vi "LabviewImageProcess with Matlab.vi"() -> ()   [LabVIEW 2015]
doc: "This is the interface, the one VI which loads all the others. Run this one first.\n\n(the line below ensures settings are saved)\n[Red Tweezers Save Settings]"
uses:
  red_tweezers_1_4_release/subvis/line_trapping.ctl
  red_tweezers_1_4_release/subvis/spot.ctl
  <vilib>/userdefined/High Color/IMAQdx.ctl
  red_tweezers_1_4_release/subvis/selection_element.ctl
  red_tweezers_1_4_release/subvis/mouse_info.ctl
  <vilib>/Analysis/baseanly.llb/Real A x B.vi
  red_tweezers_1_4_release/subvis/red_tweezers_globals_INTERNAL_VOLATILE.vi
  red_tweezers_1_4_release/subvis/red_tweezers_globals.vi
  <vilib>/Analysis/NI_AALBase.lvlib
  <vilib>/vision/driver/NI_Vision_Acquisition_Software.lvlib
  <vilib>/vision/NI_Vision_Development_Module.lvlib
panel:
  out "Spot Storage":T1[](array[typedef]) {"Amplitude Correction" step=0.1; "Line Trapping"."Phase Gradient" step=0.05; "Line Trapping"."Vector"."x" step=1e-06 format="%#_6p"; "Line Trapping"."Vector"."y" step=1e-06 format="%#_6p"; "Line Trapping"."Vector"."z" step=1e-06 format="%#_6p"; "NA Position"."r" step=1e-06; "NA Position"."y" step=1e-06; "NA Position"."x" step=1e-06; "Position"."z" step=1e-06; "Position"."y" step=1e-06; "Position"."x" step=1e-06; "Phase" step=0.7753; "Intensity" step=0.1}
  out "# selected":i16
  out "Last Pattern":T1[](array[typedef]) {"Amplitude Correction" step=0.1; "Line Trapping"."Phase Gradient" step=0.05; "Line Trapping"."Vector"."x" step=1e-06 format="%#_6p"; "Line Trapping"."Vector"."y" step=1e-06 format="%#_6p"; "Line Trapping"."Vector"."z" step=1e-06 format="%#_6p"; "NA Position"."r" step=1e-06; "NA Position"."y" step=1e-06; "NA Position"."x" step=1e-06; "Position"."z" step=1e-06; "Position"."y" step=1e-06; "Position"."x" step=1e-06; "Phase" step=0.7753; "Intensity" step=0.1}
  out "Plugins":T3(array[cluster])=[{"Name"="ASI Stage", "Folder"=path "C:/Users/Richard Bowman/Dropbox/red_tweezers_1_4_rc4/plugins/ASI Stage.llb", "vi reference"=refnum, "Needs to be run"=TRUE, "Error"={"status"=FALSE, "code"=0, "source"=""}}, {"Name"="iTweezers", "Folder"=path "C:/Users/Richard Bowman/Dropbox/red_tweezers_1_4_rc4/plugins/iTweezers.llb", "vi reference"=refnum, "Needs to be run"=TRUE, "Error"={"status"=FALSE, "code"=0, "source"=""}}, {"Name"="MightexLED", "Folder"=path "C:/Users/Richard Bowman/Dropbox/red_tweezers_1_4_rc4/plugins/MightexLED.llb", "vi reference"=refnum, "Needs to be run"=TRUE, "Error"={"status"=FALSE, "code"=0, "source"=""}}]
  in  "Tab":T4(tab)
  out "Play Pressed":bool
  out "Y":dbl
  out "X":dbl
  in  "O Button":bool
  in  "OK Button":bool
  in  "Bubble Size":dbl=50.0002
  out "Hit Indicator":bool
  in  "On":bool
  out "Induce check":bool
  out "Area+ Buffer":dbl
  in  "Area to check":dbl=0.00025
  out "Prev Current Spot":dbl
  out "spots selected 2":i32=4
  out "Spot # Check":dbl
  out "Orig Y SC":dbl
  out "Orig X SC":dbl
  out "ID num check":dbl
  out "Value Check":dbl
  out "ID":dbl[](array[numeric])
  out "Null array":dbl[](array[numeric])
  out "Potential Collisions":dbl
  out "What to Check":dbl[](array[numeric])
  out "Num":dbl
  out "Old Y":dbl
  out "Old X":dbl
  out "init":dbl
  out "Looper":bool
  in  "Output to SLM":bool
  out "Maximum":dbl
  out "Projected Distance":dbl
  out "Previous Distance":dbl
  out "Group ID #":dbl
  in  "Buffer Zone":dbl=7e-05
  out "# of Spots":dbl
  out "Distance":dbl
  out "Hit":bool
  out "Y Displacement":dbl
  out "X Displacement":dbl
  out "Current Spot #":dbl
  out "spots selected":i32=4
  in  "lock aspect ratio":bool=TRUE
  in  "Size":cluster{"x":dbl, "y":dbl, "z":dbl} {"z" step=1e-06 format="%#_4p"; "y" step=1e-06 format="%#_4p"; "x" step=1e-06 format="%#_4p"}
  in  "Position":cluster{"x":dbl, "y":dbl, "z":dbl}={"x"=1e-06, "y"=-6.3e-06, "z"=0.0} {"z" step=1e-06 format="%#_4p"; "y" step=1e-06 format="%#_4p"; "x" step=1e-06 format="%#_4p"}
  in  "phase":dbl step=0.7753
  in  "Vortex Charge":i8
  in  "Intensity":dbl=1.0 step=0.1
  in  "add to selection":bool
  in  "random position":bool
  in  "new spot":bool
  in  "delete":bool
  out "Execution Time":u32
  in  "rotate":bool
  in  "Rotation Axis":u16(ring)=2 items=["Z", "X", "Y", "Custom"]
  in  "Angle (degrees)":dbl=2.0
  in  "Custom Axis":cluster{dbl, dbl, dbl}
  in  "Spot Shape":enum32{"Normal", "Line", "NA", "Mixed"}(tab)=enum."Mixed"
  in  "Line Trapping":T2 {"Phase Gradient" step=0.05; "Vector"."x" step=1e-06 format="%#_4p"; "Vector"."y" step=1e-06 format="%#_4p"; "Vector"."z" step=1e-06 format="%#_4p"}
  in  "Scale back aperture":dbl=1.1 step=0.1
  in  "Scale BA":bool
  in  "Position on back aperture":cluster{"x":dbl, "y":dbl}={"x"=-5.84327907697451e-18, "y"=0.0} {"y" step=0.1 format="%#_4p"; "x" step=0.1 format="%#_4p"}
  in  "Radius on back aperture":dbl=1.1 step=0.1
  in  "Generate":bool
  in  "Pattern":T5(tab)
  in  "Spots across centre":i32=5
  in  "Reference Array?":bool
  in  "Fraction of SLM":dbl=1.0
  in  "Spots across centre":i32=5
  in  "N":cluster{i32, i32}
  in  "spacing/m":dbl=2.0
  in  "Iterations":i32=10
  out "non-uniformity":dbl(slide)=0.031119223416512406 scale=0.0..0.2
  out "efficiency":dbl(slide)=0.8985936267644501 scale=0.0..1.0
  in  "Optimise":bool
  in  "Reset Phase/Amplitude":bool
  in  "Fall-off/m":dbl=0.00025 min=0.0 step=1e-06 format="%#_4p"
  in  "Abort Plugin":bool
  in  "Plugin:":u16(ring)=1 items=["ASI Stage", "iTweezers", "MightexLED"]
  in  "Save Video":bool
  in  "Global ROI (requires restart)":i32[](array[numeric])=[0, 0, 1280, 512]
  in  "Zoom":bool
  in  "Draw ROI":bool
  in  "Zoom to Fit":bool
  out "Image Information":string="640x480 1.93X 8-bit image 255    (0,0)"
  in  "Camera":T6
  in  "Time per Frame (ms)":dbl
  in  "Edit Sequence Mode":bool
  in  "Manual Edit":bool
  in  "Bubble ID to Empty":dbl
  in  "Clearance Button":bool
  in  "Manual Sequence":bool
  in  "Play Sequence":bool
  in  "Reset":bool
  out "Sequence Instances":dbl
  out "Counter":dbl
  in  "Save State":bool
  out "Sequence On?":bool
  in  "Sequence Order":dbl
  out "Selection/Group":T7[](array[typedef])
  in  "Sequence Storer":T1[][](array[typedef]) {"Amplitude Correction" step=0.1; "Line Trapping"."Phase Gradient" step=0.05; "Line Trapping"."Vector"."x" step=1e-06 format="%#_6p"; "Line Trapping"."Vector"."y" step=1e-06 format="%#_6p"; "Line Trapping"."Vector"."z" step=1e-06 format="%#_6p"; "NA Position"."r" step=1e-06; "NA Position"."y" step=1e-06; "NA Position"."x" step=1e-06; "Position"."z" step=1e-06; "Position"."y" step=1e-06; "Position"."x" step=1e-06; "Phase" step=0.7753; "Intensity" step=0.1}
  out "NewXYRates":dbl[][](array[numeric])
  out "NewXYArraySize":dbl
  out "NewXYArray":dbl[][](array[numeric])
  out "Rates":dbl
  out "LCS Y":dbl
  out "LCS X":dbl
  out "LCS":dbl
  in  "Play":bool
  out "Initiate Creation 2":dbl
  out "Max Number of Bubbles 2":dbl
  in  "Number of Planned Sequence Frames 2":dbl
  in  "Add Additional Frames":bool
  in  "Frame Location":dbl
  in  "Additional Frames Wanted":dbl
  in  "Tab Control":enum32{"Line", "Arc"}(tab)
  out "X Rate":dbl
  out "Y Rate":dbl
  out "Degree Rate":dbl
  out "Radians":dbl
  out "Center Y":dbl
  out "Center X":dbl
  in  "Radius X":dbl
  in  "Theta":dbl
  in  "Lock Current Spot":bool
  out "Locked Current Spot":dbl
  out "Numeric":dbl
  out "probe":dbl
  in  "Insert":bool
  in  "Start at Which Frame?":dbl
  out "Original Y":dbl
  out "Original X":dbl
  in  "Mark Original Position":bool
  out "New Y":dbl
  out "New X":dbl
  out "Spot Storage 2":T1[](array[typedef]) {"Amplitude Correction" step=0.1; "Line Trapping"."Phase Gradient" step=0.05; "Line Trapping"."Vector"."x" step=1e-06 format="%#_6p"; "Line Trapping"."Vector"."y" step=1e-06 format="%#_6p"; "Line Trapping"."Vector"."z" step=1e-06 format="%#_6p"; "NA Position"."r" step=1e-06; "NA Position"."y" step=1e-06; "NA Position"."x" step=1e-06; "Position"."z" step=1e-06; "Position"."y" step=1e-06; "Position"."x" step=1e-06; "Phase" step=0.7753; "Intensity" step=0.1}
  in  "Save":bool
  in  "Load":bool
  in  "Camera Capture":bool
  out "Bubble y":dbl
  out "Bubble x":dbl
  out "Number of Matches Returned":dbl
  out "bottomry":dbl
  out "toply":dbl
  out "bottomrx":dbl
  out "toplx":dbl
  in  "Send Data":bool
  out "Camera 2":T8(plugin-control)
  out "Circles":T9(array[cluster]) {"Position"."Y" format="%.2f"; "Position"."X" format="%.2f"}
  out "Video Frame Rate":dbl(knob)=50.00000000000003 scale=0.0..100.0 scale format="%.1f"
  out "Interface Frame Rate":dbl(knob)=97.23240312927678 scale=0.0..100.0 scale format="%.1f"
  in  "stop":bool=TRUE
  out "MOP pressed":bool
  out "MOP pressed After":bool
  out "X Pos every 10 sec":dbl
  out "Elapsed Time":dbl
  out "Position Indicator":string
  out "Spot Checker":T1[](array[typedef]) {"Amplitude Correction" step=0.1; "Line Trapping"."Phase Gradient" step=0.05; "Line Trapping"."Vector"."x" step=1e-06 format="%#_6p"; "Line Trapping"."Vector"."y" step=1e-06 format="%#_6p"; "Line Trapping"."Vector"."z" step=1e-06 format="%#_6p"; "NA Position"."r" step=1e-06; "NA Position"."y" step=1e-06; "NA Position"."x" step=1e-06; "Position"."z" step=1e-06; "Position"."y" step=1e-06; "Position"."x" step=1e-06; "Phase" step=0.7753; "Intensity" step=0.1}
  out "Image":T8(plugin-control)
  # "Notes:\n\nIf you are doing non-sequence controls,\nthe delete function can be used as intended.\nHowever, do not use the delete function after\nrunning a sequence! Using it will prevent\nthe bubbles from appearing as the\nnumber of spots will change, which is\nessential for the sequence to work (it would\nbe displaying the maximum number of\nbubbles). \n\nIf you happen to delete a bubble, it can be \nrestored by inserting a new spot. Once enough\nspots have been restored, click on manual edit\nto correct the # of spots tracker. It should \nbe restored to where it originally was."
  # "The SLM can be used to shape spots; here you can restrict the NA of a spot (so it comes only from part of the back aperture), or create a line-trap"
  # "The traps do not have any spot-shaping applied (so they should just be diffraction-limited focal spots)."
  # "This shapes the amplitude (and phase) of the beam to create extended line traps.  The \"Phase Gradient\" control allows the Poynting vector to push things along the line.  Unfortunately, some work is needed on the scaling factors so the phase gradient control will need tweaking if the line trap has a nonzero z component."
  # "By default,each spot comes from the whole back aperture.  Here, you can limit a spot to come from a specific part of the back aperture."
  # "The control below allows you to scale the whole back aperture (i.e. the position and size of all the apertures).  It's a one-time operation, i.e. only changes things when you push \"ok\"."
  # "A Combination of line-trapping and NA restriction has been applied to these traps.  You can get at the line trap or NA parameters on the other tabs, switching to the NA tab does not delete the line-trap settings."
  # "This tab generates Shack-Hartmann type holograms, which are often useful when aligning the system, and arrays of spots."
  # "The controls above only work when using the \"IMAQdx with ROI Buttons\" case in the bottom loop.  You can save video regardless of camera code though."
  # "Manual Edit allows a user to\ngo to a specific sequence frame."
  # "To clear the sequence, you must\nclear the array. Right click on sequence\nstorer to do this."
  # "Use this to \"clear\" a \nspecific bubble. If\nworking on a sequence,\nuse this as your delete\nbutton! You can update\nthe view by using manual edit."
  # "Use the reset button\nto clear counter.\nIt becomes necessary\nwhen you clear the array,\nespecially in manual mode."
  # "Use the sequence creator tab to specify the\nnumber of bubbles you want along with\nthe number of frames.\n\nTo save at a specific interval, the sequence\norder can be used to place the state. If used\nto correct something, it will replace the\nentire sequence frame.\n\n\"Sequence On?\" is only used in auto mode."
  # "Frame Location must be\nwhere you want to add\nthe frames to (ie having \n4 as an input would have\nthe additional frames\nstart at array row 5."
  # "Multiple bubbles can  be done with the\nline function. One bubble at a time for the arc\nfunction."
  # "Using the Load/Save function:\n\nRed Tweezers itself is unable to save long \nsequences, but a separate program is able to\naccomplish this. To do this, follow these\nsteps:\n\n1. After creating your sequence, press the save\nbutton below.\n\n2. Then, go to the subvi folder and find\nSequenceSaver.vi.\n\n3. At the control \"Sequence Storer,\" right-click\nthe dimensions part of the array and go to\ndata operations.\n\n4. Press \"Make Current Values Default\" and save\nthe sequence.\n\n5. The next time you load the program, simply\npress load to re-acquire the sequence. You\nwill need to insert the bubbles again, but after\nthe first frame can be recovered by using\nSequenceControl.vi."
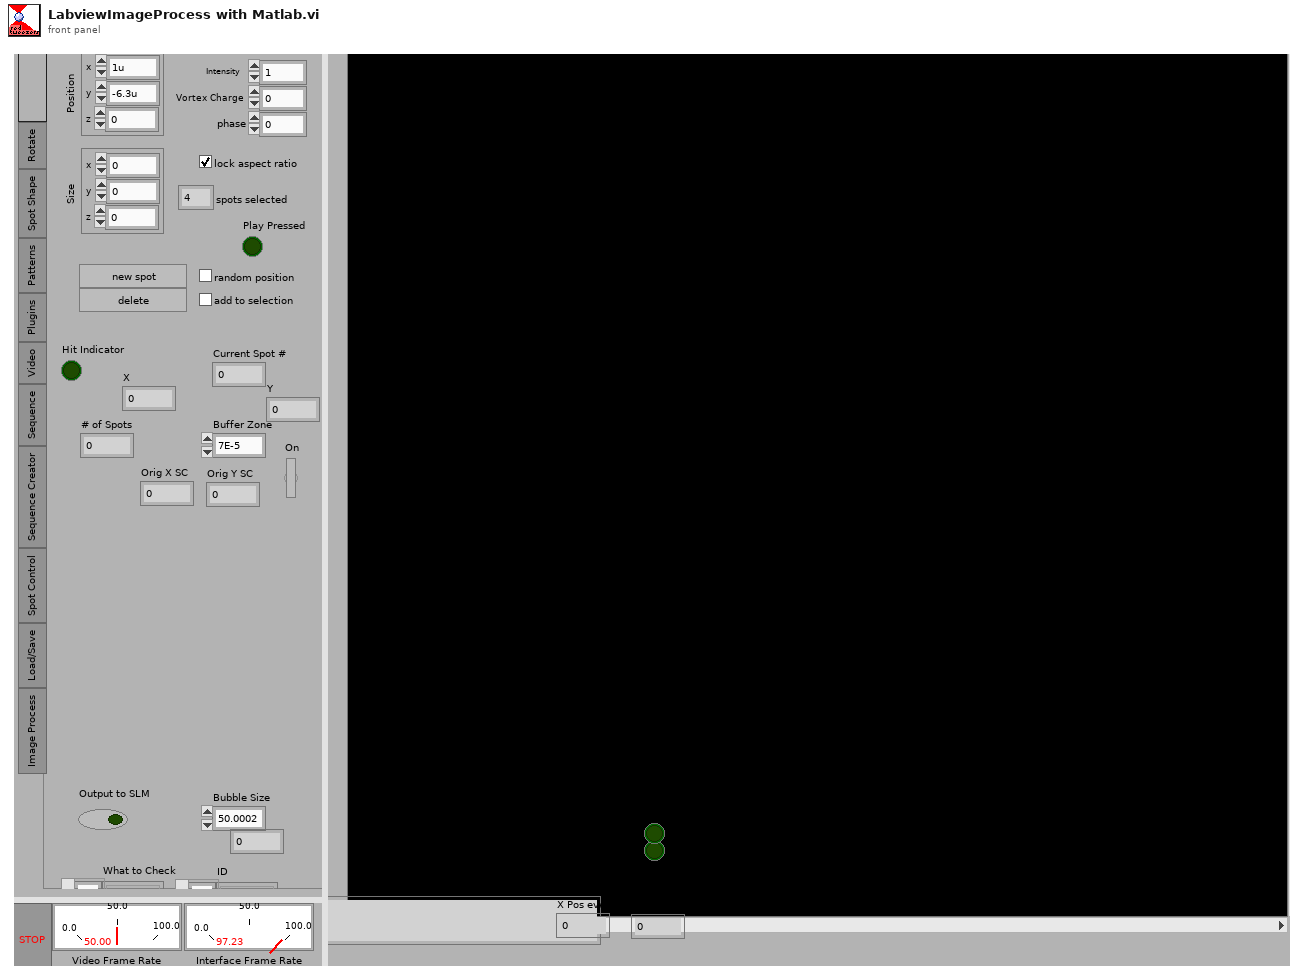
[diagram p1: front panel]
types:
  T1 = typedef "spot.ctl" = cluster{"Position":cluster{"x":dbl, "y":dbl, "z":dbl}, "Intensity":dbl, "Vortex Charge":i8, "Phase":dbl, "NA Position":cluster{"x":dbl, "y":dbl, "r":dbl}, "Line Trapping":T2, "Amplitude Correction":dbl}
  T2 = typedef "line_trapping.ctl" = cluster{"Vector":cluster{"x":dbl, "y":dbl, "z":dbl}, "Phase Gradient":dbl}
  T3 = cluster{"Name":string, "Folder":path, "vi reference":refnum<vi>, "Needs to be run":bool, "Error":errorcluster}[]
  T4 = enum32{"Current Spot", "Rotate", "Spot Shape", "Patterns", "Plugins", "Video", "Sequence", "Sequence Creator", "Spot Control", "Load/Save", "Image Process"}
  T5 = enum32{"HCP Shack-Hartmann", "Square Shack-Hartmann", "Rectangular Grid"}
  T6 = typedef "IMAQdx.ctl" = refnum<k21>
  T7 = typedef "selection_element.ctl" = cluster{"Group ID":i32, "Selected":bool}
  T8 = typedef "IMAQ Image.ctl" = refnum<image>
  T9 = cluster{"Position":cluster{"X":sgl, "Y":sgl}, "Radius":dbl, "Score":dbl}[]
  T10 = typedef "mouse_info.ctl" = cluster{"Button Down":bool, "Dragging":bool, "Position (Image Pixels)":cluster{"X":dbl, "Y":dbl}, "Previous Position (Image Pixels)":cluster{"X":dbl, "Y":dbl}, "Button":u16, "Mods":cluster{"Double Click":bool, "Menu Key":bool}, "PlatMods":cluster{"Shift":bool, "Ctrl":bool, "Alt":bool, "Cmd":bool, "Opt":bool}}
  T11 = cluster{"Position":cluster{"x":dbl, "y":dbl, "z":dbl}, "Intensity":dbl, "Vortex Charge":i8, "Phase":dbl, "NA Position":cluster{"x":dbl, "y":dbl, "r":dbl}, "Line Trapping":T2, "Amplitude Correction":dbl}
  T12 = enum16{"Set guide visibility", "Set grid visibility", "Show front panel", "Render on image"}
  T13 = enum32{"Current Spot", "Rotate", "Spot Shape", "Patterns", "Plugins", "Video"}
  T14 = enum16{"Left Button", "Center Button", "Right Button", "Window Close"}
  T15 = typedef "Image Type" = u32
  T16 = cluster{"number: 0 to 1":dbl, "number: 0 to 1":dbl}
  T17 = typedef "NI_Matrix.lvlib/RealMatrix.ctl" = dbl[][]
  T18 = typedef "overlay_element.ctl" = cluster{"Tool":enum16{"Lines", "Oval", "Rectangle", "Text"}, "Points":cluster{"X":dbl, "Y":dbl}[], "Drawing Mode":u32, "Color":u32, "String":string}
  T19 = enum32{"Current Spot", "Rotate", "Spot Shape", "Patterns", "Plugins", "Video", "Particle Tracking", "Clamping", "Blank"}[]
  T20 = typedef "LVMenuShortCut.ctl" = cluster{"include Shift key?":bool, "include Ctrl key?":bool, "shortcut key":string}
  T21 = typedef "LVPoint32TypeDef.ctl" = cluster{"Horizontal":i32, "Vertical":i32}
  T22 = cluster{"Shift":bool, "Ctrl":bool, "Alt":bool, "Cmd":bool, "Opt":bool}
  T23 = cluster{"Button Down":bool, "Dragging":bool, "Mouse Coords (image pixels)":cluster{dbl, dbl}, "Mouse Coords (image pixels)":cluster{dbl, dbl}, "Button":u16, "Mods":cluster{"Double Click":bool, "Menu Key":bool}, "PlatMods":cluster{"Shift":bool, "Ctrl":bool, "Alt":bool, "Cmd":bool, "Opt":bool}}
  T24 = cluster{"Position":cluster{"X":sgl, "Y":sgl}, "Radius":dbl, "Score":dbl}
  T25 = cluster{"[0]":dbl, "[1]":dbl, "[2]":dbl, "[3]":dbl}
  T26 = cluster{"NewXYArray[0]":dbl, "NewXYArray[1]":dbl, "NewXYArray[2]":dbl, "NewXYArray[3]":dbl, "NewXYArray[4]":dbl, "NewXYArray[5]":dbl, "NewXYArray[6]":dbl, "NewXYArray[7]":dbl, "NewXYArray[8]":dbl}
  T27 = cluster{"Average Frame Time":dbl, "millisecond timer value":u32}
  T28 = cluster{"Position":cluster{"x":dbl, "y":dbl, "z":dbl}, "Intensity":dbl, "Vortex Charge":i8, "Phase":dbl, "NA Position":cluster{"x":dbl, "y":dbl, "r":dbl}, "Line Trapping":T2, "Amplitude Correction":dbl}[]
  T29 = enum32{"Bad", "Idle", "Run top level", "Running"}
  T30 = typedef "AviRefnum.ctl" = refnum<k1>
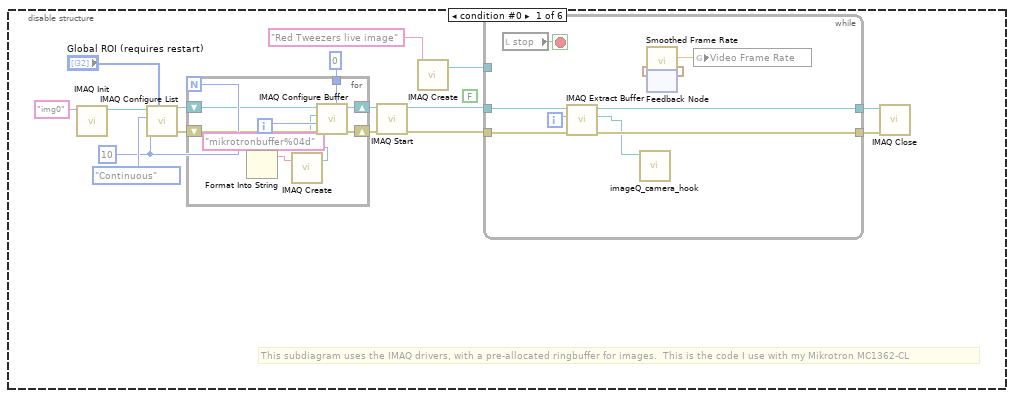
[diagram p3: hidden frame]
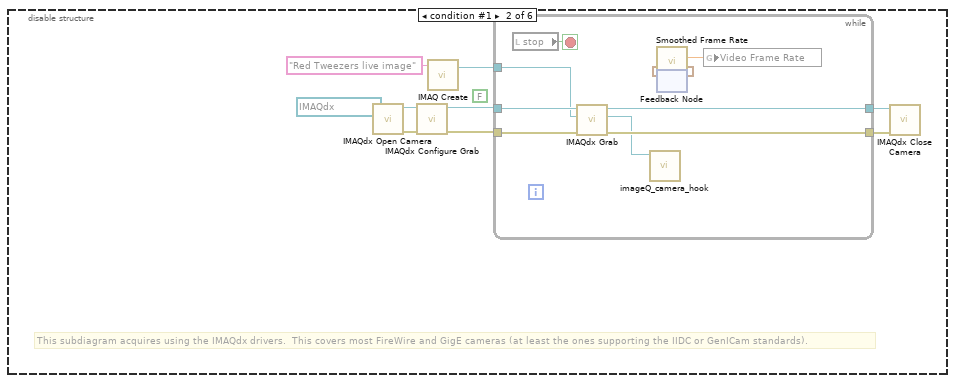
[diagram p4: hidden frame]
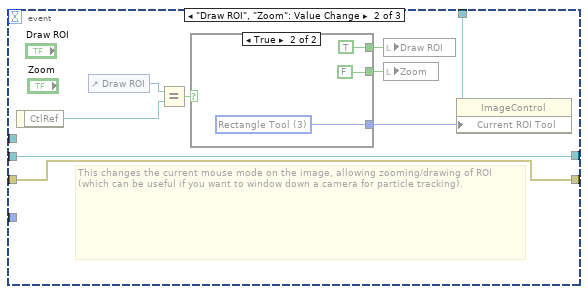
[diagram p5: hidden frame]
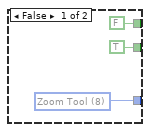
[diagram p6: hidden frame]
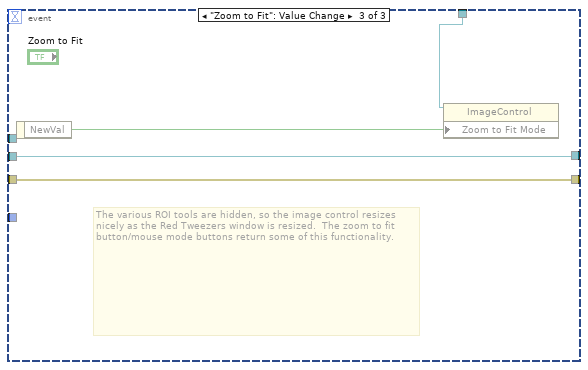
[diagram p7: hidden frame]
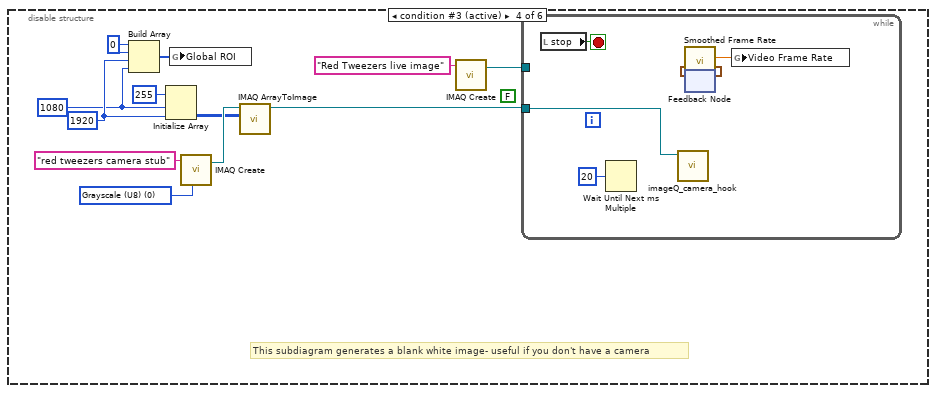
[diagram p8: hidden frame]
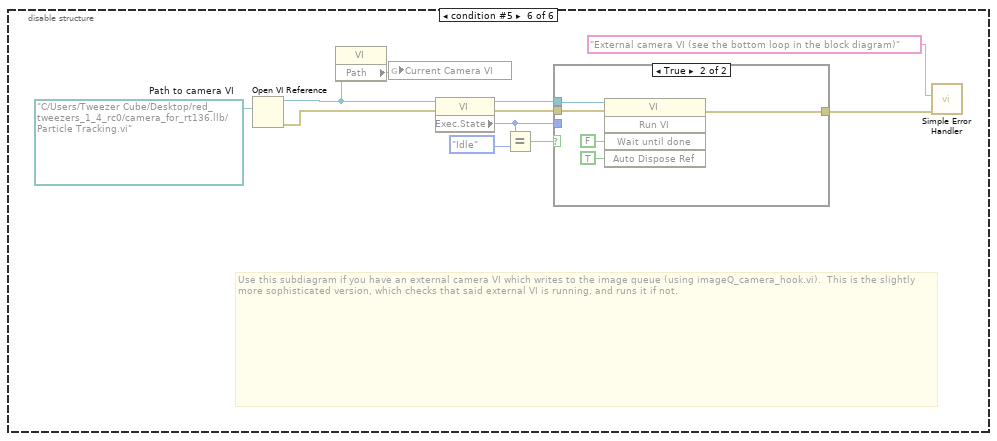
[diagram p10: hidden frame]
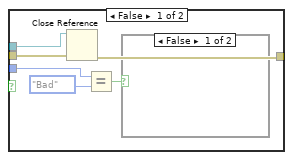
[diagram p11: hidden frame]
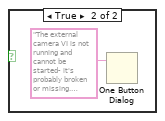
[diagram p12: hidden frame]
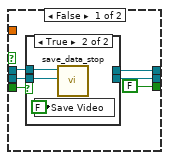
[diagram p13: hidden frame]
diagram:
  w14 = "red_tweezers_display_imageQ" ("Queue Name")
  w26 = T10 {"Button Down"=FALSE, "Dragging"=FALSE, "Position (Image Pixels)"={"X"=0.0, "Y"=0.0}, "Previous Position (Image Pixels)"={"X"=0.0, "Y"=0.0}, "Button"=0, "Mods"={"Double Click"=FALSE, "Menu Key"=FALSE}, "PlatMods"={"Shift"=FALSE, "Ctrl"=FALSE, "Alt"=FALSE, "Cmd"=FALSE, "Opt"=FALSE}}  # Mouse Information
  w27 = refnum<vi> refnum  # Image
  # "The funny looking feedback-node structure is deliberate (if odd).  We want to reload settings from the last used file (stored in the registry) only if this program has not been run since it was last loaded from file/recompiled.  That's why I use an uninitialised shift register: every time the program runs, it increments.  So, if it is zero, this is our first run (or we've been recently recompiled)."
  # "This loop handles the video that is displayed on-screen and saved to file."
  # "Initially, we only register to be told when the user clicks the image"
  # "This is the actual image control"
  # "This is a generic reference.\nIt is just a placeholder, so we can register for events later."
  # "This version of red tweezers uses two coordinate systems: \n1. Real Coordinates - corresponding to physical distances in 3D in microns\n2. Image Coordinates - position on the camera image, relative to the top left of the CURRENT ROI, measured in pixels. If the ROI changes, the relationship between \"real units\" and \"image pixels\" may change, so all values should be stored and presented to the user in REAL units unless there is a good reason to do otherwise."
  n1 = Tick Count (ms)() -> (millisecond timer value=w1:u32)
  n2 = control-ref of="Plugin Pnl"() -> (w23:refnum<vi>)
  n3 = flat-sequence {
    tunnel: [w30] -> w9
    tunnel: w7 -> [_]
    frame #0 {
      n4 = vi-ref "red_tweezers_globals_INTERNAL.vi"() -> (w31:refnum<vi>)
      n5 = property class="VI"(reference=w31) -> ("Path"=w30:path)  [unwired: 1 in, 2 out]
      n6 = global write "red_tweezers_globals_INTERNAL_VOLATILE.vi" "Current Camera VI"(w30) -> ()
    }
  }
  n7 = control-ref of="Plugin:"() -> (w24:refnum<vi>)
  n8 = feedback #1() -> (w17:dbl)  [unwired: 1 in]
  n9 = Equal To 0?(x=w17) -> (x = 0?=w16:bool)
  n10 = Increment(x=w17) -> (x+1=w15:dbl)
  n11 = feedback-in #1(w15) -> ()
  n12 = call "plugins_load.vi"("Sub Panel"=w23, "Plugin Chooser"=w24) -> ("error out"=w18:errorcluster, "Plugins"=w20:T3)  [unwired: 2 in, 2 out]
  "Plugins" <- w20
  n13 = control-ref of="Image"() -> (w8:refnum<vi>)
  n14 = case shown="True" w16 {
    tunnel: w18 -> [_ w32]
    tunnel: [_ w32] -> w7
    frame False {
    }
    frame True {
      n15 = call "settings_load_default_file.vi"("error out"=w32) -> ()
    }
  }
  n16 = flat-sequence {
    tunnel: w7 -> [_]
    tunnel: w5 -> [w34]
    frame #0 {
      # "ensure we don't accidentally start saving video, and run UDP Sender to set up the hologram window."
      n17 = local write "Save Video"(FALSE ("background subtraction")) -> ()
      n18 = call "UDP Sender generic_2.vi"("Spots"=w34) -> ()  [unwired: 2 in, 1 out]
    }
  }
  n19 = global read "red_tweezers_globals.vi" "Selection/Group"() -> (w25:T7[])
  n20 = register-events(w8, w27, w27, w27) -> (reference out=w28:refnum<event-registration>)  [unwired: 2 in, 1 out]
  n21 = global read "red_tweezers_globals.vi" "Spots"() -> (w5:T1[])
  n22 = local write "stop"(FALSE ("STOP")) -> ()
  n23 = call "ensure_selection_matches_spots.vi"("Selection and Groups in"=w25, "Spots"=w5) -> ("Selection and Groups out"=w29:T7[], "Spots (duplicate)"=w4:T1[])  [unwired: 4 in]
  n24 = call "IMAQ Create"("Image Name"=w14) -> ("New Image"=w12:T8)  [unwired: 4 in, 1 out]
  n25 = call "imageQ_create_return_queue.vi"("Queue Name"=w14) -> ("queue out"=w13:refnum<queue>)
  n26 = while {
    shift-right: [w124] -> _
    shift-left: w4 -> [w144]
    shift-right: [w143] -> _
    shift-left: w29 -> [w142]
    shift-right: [w146] -> _
    shift-left: _ -> [w137]
    shift-right: [w145] -> _
    shift-left: _ -> [w136]
    tunnel: w8 -> [w141]
    shift-right: [w135] -> _
    shift-left: w26 -> [w134]
    shift-right: [w138] -> _
    shift-left: w28 -> [w139]
    border: errorcluster {"status"=FALSE, "code"=0, "source"=""} ("error out") -> [_]
    tunnel: [errorcluster {"status"=FALSE, "code"=0, "source"=""} ("error in (no error)")] -> w21
    border: w20 -> [_]
    tunnel: w4 -> [w125]
    tunnel: [w36] -> w3
    stop <- w126 stop-if-true
    w44 = 7 items=["Red", "Green", "Blue", "Hue", "Saturation", "Luminance", "Value", "Intensity"] ("Color Plane")
    w48 = T15 0 items=["Grayscale (U8)", "Grayscale (I16)", "Grayscale (SGL)", "Complex (CSG)", "RGB (U32)", "HSL (U32)", "RGB (U64)", "Grayscale (U16)"] ("Image Type")
    # "The function inserts the newly generated sequence for the automatic sequence generator. It also contains the code\nthe code necessary to check whether the bubbles will intersect with each other in the sequence."
    # "This calculates the size of the area including the buffer zone length.\nThe bubble diameter will also be included in the near future."
    # "The statement to the right controls the area that are being chcecked and checks\nwhich bubbles need to be checked.  There are two instances where this activates\nin this case:\n\nWhen a new bubble is selected\nWhen a bubble is deselected, reverting to the last current spot #\n\nThe other case, when the bubble moves out of the area specified, is located\ninside the while loop controlling the bubble movement with a mouse."
    # "Timer function example"
    # "These functions help with the calculations for the sequence generator."
    # "This loads the sequence from the \"saver\" VI. The save function below \"saves\" the sequence into the saver VI."
    # "The VI above is SequenceSaver.vi which contains the\ncode necessary to create a sequence."
    # "This case structure is the Save State structure. This stores\nthe current state of the bubbles (ie position)."
    # "Reset sets the counter back to zero. This is particularly useful \nwhen using the manual sequence."
    # "This case structure helps to continue the sequence.\nThis takes the true case of the Sequence On? function\nor the true case for the Manual Sequence function\nin order to go to the next sequence frame."
    # "This case structure allows for the playing of the sequence.\nThe amount of time it takes to go through the sequence\ncan be edited on the current spot menu."
    # "We only write to the image overlay when we are in one of the tabs, to prevent it disappearing when we are (for example) using the mouse."
    # "These wires control saving undo info. See the VI below's tip strips for details."
    # "Setting these wires to false means:\n(1) dragging moves the selection\n(2) clicking spots changes selection\nset them to true to stop the default mouse behaviour, don't wire them straight through!"
    n27 = event shown="[0] Timeout" {
      selector: w139 -> [w504 w1175 w1180 w1402 w1430 w1447 w1544 _]
      dyn-events: [w504 w1174 w1180 w1400 w1427 w1448 w1544 _] -> w138
      timeout: 0 -> [_ _ _ _ _ _ _ _]
      tunnel: [w512 _ w1182 w1397 w1432 w1439 w1531 _] -> w146
      tunnel: [w511 _ w1181 w1396 w1431 w1438 w1535 _] -> w145
      tunnel: [w510 _ _ _ _ _ _ _] -> w97
      tunnel: w144 -> [w509 w1170 w1187 w1392 w1425 w1444 w1539 w1862]
      tunnel: [w508 w1170 w1185 w1392 w1425 w1435 w1537 w1862] -> w132
      tunnel: [w507 w1169 w1184 w1381 w1424 w1445 w1527 w1861] -> w131
      tunnel: w142 -> [w506 w1169 w1186 w1381 w1424 w1443 w1538 w1861]
      tunnel: w141 -> [w505 w1171 w1177 w1391 w1428 w1446 w1540 _]
      tunnel: [w503 _ w1179 w1401 T10 {"Button Down"=FALSE, "Dragging"=FALSE, "Position (Image Pixels)"={"X"=0.0, "Y"=0.0}, "Previous Position (Image Pixels)"={"X"=0.0, "Y"=0.0}, "Button"=0, "Mods"={"Double Click"=FALSE, "Menu Key"=FALSE}, "PlatMods"={"Shift"=FALSE, "Ctrl"=FALSE, "Alt"=FALSE, "Cmd"=FALSE, "Opt"=FALSE}} T10 {"Button Down"=FALSE, "Dragging"=FALSE, "Position (Image Pixels)"={"X"=0.0, "Y"=0.0}, "Previous Position (Image Pixels)"={"X"=0.0, "Y"=0.0}, "Button"=0, "Mods"={"Double Click"=FALSE, "Menu Key"=FALSE}, "PlatMods"={"Shift"=FALSE, "Ctrl"=FALSE, "Alt"=FALSE, "Cmd"=FALSE, "Opt"=FALSE}} w1543 _] -> w135
      tunnel: w134 -> [w503 _ w1179 _ _ w1442 w1534 _]
      tunnel: w137 -> [_ _ w1182 w1397 w1432 w1439 w1531 _]
      tunnel: w136 -> [_ _ w1181 w1396 w1431 w1438 w1535 _]
      tunnel: [w502 _ _ _ _ _ _ _] -> w133
      tunnel: [_ _ w1178 _ _ _ TRUE _] -> w130
      tunnel: [_ _ _ TRUE TRUE TRUE FALSE _] -> w129
      tunnel: [TRUE _ _ _ _ _ _ _] -> w127
      tunnel: [_ _ _ _ _ _ _ "stop"] -> w126
      tunnel: w125 -> [_ _ _ _ _ _ w1528 _]
      event Timeout {
        n28 = event-data() -> ()  [unwired: 1 in, 1 out]
        n29 = case shown="\"Current Spot\", Default" "Tab" {
          tunnel: [w527 w795 w942 w1044 w1125 w1163] -> w508
          tunnel: w509 -> [w524 w797 w943 w1046 w1125 w1163]
          tunnel: w506 -> [w513 w796 w940 w1045 w1124 w1162]
          tunnel: [w526 w794 w941 w1043 w1124 w1162] -> w507
          tunnel: [w514 _ TRUE _ _ _] -> w512
          tunnel: [w514 _ _ _ _ _] -> w511
          tunnel: [_ _ _ FALSE _ _] -> w510
          tunnel: w505 -> [_ _ _ _ _ w1159]
          tunnel: w503 -> [_ _ w922 _ _ _]
          tunnel: [_ _ w924 _ _ _] -> w502
          frame "Current Spot", Default {
            w514 = FALSE
            # "The function below contains the code necessary to use the automatic sequence generator to create specific movements. It also helps translate cases where the point is entered in not dragged.\nThis prevents bubbles from intersecting if the bubble is told not to intersect."
            # "If it's out of date, update front panel"
            n30 = call "find_centroid.vi"("Selection and Groups"=w513, "Spots"=w524) -> ("Mean Values"=w522:T1, "size"=w516:cluster{"x":dbl, "y":dbl, "z":dbl}, "centroid"=w517:cluster{"x":dbl, "y":dbl, "z":dbl}, "# selected"=w515:i16)  [unwired: 2 in, 1 out]
            n31 = stacked-sequence {
              tunnel: w515 -> [_ w529]
              frame #0 {
                n32 = local read "spots selected"() -> (→"spots selected 2":i32)
              }
              frame #1 {
                "spots selected" <- w529
              }
            }
            n33 = feedback-in #2(w522) -> ()
            n34 = feedback #2() -> (w523:T1)  [unwired: 1 in]
            n35 = feedback #3() -> (w521:cluster{"x":dbl, "y":dbl, "z":dbl})  [unwired: 1 in]
            n36 = feedback-in #3(w516) -> ()
            n37 = Not Equal?(x=w523, y=w522) -> (x != y?=w520:bool)
            n38 = Not Equal?(x=w521, y=w516) -> (x != y?=w519:bool)
            n39 = Or(x=w520, y=w519) -> (x .or. y?=w518:bool)
            n40 = case shown="True" w518 {
              tunnel: w522 -> [_ w535]
              tunnel: w516 -> [_ w531]
              frame False {
              }
              frame True {
                n41 = Unbundle By Name(w535) -> ("Position"=w530:cluster{"x":dbl, "y":dbl, "z":dbl}, "Intensity"=w533:dbl, "Vortex Charge"=w532:i8, "Phase"=w534:dbl)
                n42 = local write "Size"(w531) -> ()
                n43 = local write "Vortex Charge"(w532) -> ()
                n44 = local write "Intensity"(w533) -> ()
                n45 = local write "Position"(w530) -> ()
                n46 = local write "phase"(w534) -> ()
                n47 = Unbundle By Name(w530) -> ()  [unwired: 2 out]
              }
            }
            n48 = local write "Selection/Group"(w513) -> ()
            n49 = event shown="[3] \"Position\": Value Change" {
              selector: _ -> [_ _ _ _ _ _ _ _]
              dyn-events: _ -> [_ _ _ _ _ _ _ _]
              timeout: 10 -> [_ _ _ _ _ _ _ _]
              tunnel: w524 -> [w537 w541 w555 w578 w682 w727 w753 w776]
              tunnel: w513 -> [w536 w540 w558 w585 w669 w724 w750 w774]
              tunnel: [w537 w539 w556 w577 w670 w725 w751 w775] -> w527
              tunnel: [w536 w538 w557 w585 w669 w724 w750 w774] -> w526
              tunnel: w517 -> [_ _ _ _ w681 _ _ _]
              event Timeout {
                n50 = event-data() -> ()  [unwired: 3 out]
              }
              event "delete": Value Change {
                n51 = event-data() -> ()  [unwired: 7 out]
                n52 = call "delete_selected_spots.vi"("Selection/Group 3"=w540, "Spots 3"=w541) -> ("Selection/Group 2"=w538:T7[], "Spots 2"=w539:T1[])  [unwired: 4 in]
              }
              event "new spot": Value Change {
                # "If we're not adding it to the selection, de-select all the other spots"
                n53 = event-data() -> ()  [unwired: 7 out]
                n54 = call "coords_ROI_currentimage.vi"() -> ("Mono ROI"=w542:i32[])
                n55 = case shown="False" "add to selection" {
                  tunnel: w558 -> [w571 w576]
                  tunnel: [w570 w576] -> w553
                  frame False {
                    n56 = for {
                      tunnel: w571 -> [w574] mode=indexing
                      tunnel: [w575] -> w570 mode=indexing
                      n57 = Unbundle(w574) -> ("Group ID"=w573:i32)  [unwired: 1 out]
                      n58 = Bundle(cluster=w574, "Group ID"=w573, "Selected"=FALSE ("Label.Visible")) -> (w575:T7)
                    }
                  }
                  frame True {
                  }
                }
                n59 = Index Array(array=w542) -> (element #1=w548:i32, element #2=w549:i32, element #3=w547:i32, element #4=w546:i32)  [unwired: 4 in]
                n60 = Bundle("Numeric"=w548, "Numeric"=w549) -> (w543:cluster{"Numeric":i32, "Numeric":i32})  [unwired: 1 in]
                n61 = Bundle("Numeric"=w547, "Numeric"=w546) -> (w545:cluster{"Numeric":i32, "Numeric":i32})  [unwired: 1 in]
                n62 = Subtract(x=w545, y=w543) -> (x-y=w544:cluster{"Numeric":i32, "Numeric":i32})
                n63 = case shown="True" "random position" {
                  tunnel: [w560 w566] -> w551
                  tunnel: w544 -> [_ w562]
                  tunnel: w543 -> [_ w561]
                  frame False {
                    n64 = call "replace_position.vi"("Position"=cluster{"x":dbl, "y":dbl, "z":dbl} {"x"=0.0, "y"=0.0, "z"=0.0}) -> ("Spot"=w560:T1)  [unwired: 1 in, 2 out]
                  }
                  frame True {
                    n65 = Random Number (0-1)() -> (number: 0 to 1=w568:dbl)
                    n66 = Random Number (0-1)() -> (number: 0 to 1=w569:dbl)
                    n67 = Bundle("number: 0 to 1"=w569, "number: 0 to 1"=w568) -> (w567:T16)  [unwired: 1 out]
                    n68 = Multiply(x=w567, y=w562) -> (x*y=w564:cluster{dbl, dbl})
                    n69 = Add(x=w564, y=w561) -> (x+y=w563:cluster{dbl, dbl})
                    n70 = call "coords_image_to_real_currentimage.vi"("Position (pixels on image)"=w563) -> ("Position (real coords)"=w565:cluster{dbl, dbl, "Z":dbl})  [unwired: 9 in]
                    n71 = call "replace_position.vi"("Position"=w565) -> ("Spot"=w566:T1)  [unwired: 1 in, 2 out]
                  }
                }
                n72 = Build Array (concatenate)(w555, w551) -> (w556:T1[])
                n73 = Build Array (concatenate)(w553, cluster{i32, "Label.Visible":bool} {0, "Label.Visible"=TRUE}) -> (w557:T7[])
              }
              event "Position": Value Change {
                # "If the position has changed, translate the spots"
                n74 = event-data() -> ("OldVal"=w583:cluster{"x":dbl, "y":dbl, "z":dbl}, "NewVal"=w584:cluster{"x":dbl, "y":dbl, "z":dbl})  [unwired: 5 out]
                n75 = flat-sequence {
                  tunnel: w585 -> [w589]
                  tunnel: w582 -> [w588]
                  tunnel: w578 -> [w587]
                  tunnel: [w586] -> w579
                  frame #0 {
                    n76 = for {
                      tunnel: w587 -> [w594] mode=indexing
                      tunnel: w589 -> [w591] mode=indexing
                      tunnel: [w593] -> w586 mode=indexing
                      tunnel: w588 -> [w592]
                      n77 = Unbundle(w591) -> ("Selected"=w590:bool)  [unwired: 1 out]
                      n78 = case shown="True" w590 {
                        tunnel: w594 -> [w595 w600]
                        tunnel: [w595 w599] -> w593
                        tunnel: w592 -> [_ w596]
                        frame False {
                        }
                        frame True {
                          n79 = call "extract_position.vi"("Spot"=w600) -> ("Position"=w597:cluster{"x":dbl, "y":dbl, "z":dbl})
                          n80 = Add(x=w597, y=w596) -> (x+y=w598:cluster{"x":dbl, "y":dbl, "z":dbl})
                          n81 = call "replace_position.vi"("Position"=w598, "Spot in"=w600) -> ("Spot"=w599:T1)  [unwired: 2 out]
                        }
                      }
                    }
                  }
                }
                n82 = Subtract(x=w584, y=w583) -> (x-y=w582:cluster{"x":dbl, "y":dbl, "z":dbl})
                n83 = local read "# of Spots"() -> (w581:dbl)
                n84 = stacked-sequence {
                  tunnel: w578 -> [_ w605 _]
                  tunnel: w579 -> [_ w604 _]
                  tunnel: w581 -> [_ w603 _]
                  tunnel: [_ _ w652] -> w580
                  tunnel: w579 -> [_ _ w651]
                  tunnel: w578 -> [_ _ w650]
                  tunnel: [_ _ w649] -> w577
                  frame #0 {
                    n85 = local write "Looper"(FALSE) -> ()
                    "init" <- 0
                  }
                  frame #1 {
                    n86 = for {
                      N: w603 -> [_]
                      tunnel: w605 -> [w610]
                      tunnel: w604 -> [w615]
                      stop <- w616 stop-if-true
                      n87 = local read "init"() -> (w609:dbl)
                      n88 = Index Array(array=w615, index=w609) -> (element=w614:T1)
                      n89 = Index Array(array=w610, index=w609) -> (element=w608:T1)
                      n90 = Unbundle By Name(w614) -> ("Position.x"=w613:dbl, "Position.y"=w612:dbl)
                      n91 = local read "# of Spots"() -> (w611:dbl)
                      n92 = Unbundle By Name(w608) -> ("Position.x"=→"Old X":dbl, "Position.y"=→"Old Y":dbl)
                      n93 = local write "New X"(w613) -> ()
                      n94 = local write "New Y"(w612) -> ()
                      n95 = stacked-sequence {
                        tunnel: w610 -> [w621 _]
                        tunnel: w613 -> [w620 _]
                        tunnel: w612 -> [w619 _]
                        tunnel: w611 -> [w618 _]
                        tunnel: w609 -> [w617 _]
                        frame #0 {
                          n96 = for {
                            N: w618 -> [_]
                            tunnel: w621 -> [w643]
                            tunnel: w620 -> [w642]
                            tunnel: w619 -> [w640]
                            tunnel: w617 -> [w625]
                            i -> [w627]
                            stop <- w626 stop-if-true
                            n97 = Index Array(array=w643, index=w627) -> (element=w644:T1)
                            n98 = Unbundle By Name(w644) -> ("Position.x"=w641:dbl, "Position.y"=w639:dbl)
                            n99 = Subtract(x=w642, y=w641) -> (x-y=w638:dbl)
                            n100 = Subtract(x=w640, y=w639) -> (x-y=w637:dbl)
                            n101 = Square(x=w638) -> (x^2=w636:dbl)
                            n102 = Square(x=w637) -> (x^2=w635:dbl)
                            n103 = local read "# of Spots"() -> (w629:dbl)
                            n104 = Add(x=w636, y=w635) -> (x+y=w634:dbl)
                            n105 = local read "Buffer Zone"() -> (w624:dbl)
                            n106 = Square Root(x=w634) -> (sqrt(x)=w633:dbl)
                            n107 = Multiply(x=2, y=w624) -> (x*y=w622:dbl)
                            n108 = Less?(x=w633, y=w622) -> (x < y?=w631:bool)
                            n109 = Not Equal?(x=w625, y=w627) -> (x != y?=w630:bool)
                            n110 = Equal?(x=w629, y=w627) -> (x = y?=w632:bool)
                            n111 = And(x=w630, y=w631) -> (x .and. y?=w628:bool)
                            "Looper" <- w628
                            n112 = Or(x=w628, y=w632) -> (x .or. y?=w626:bool)
                          }
                        }
                        frame #1 {
                          n113 = local read "Looper"() -> (w645:bool)
                          n114 = case shown="False" w645 {
                            frame False {
                              n115 = local read "init"() -> (w646:dbl)
                              n116 = Add(x=w646, y=1) -> (x+y=w648:dbl)
                              n117 = local write "init"(w648) -> ()
                            }
                            frame True {
                            }
                          }
                        }
                      }
                      n118 = local read "Looper"() -> (w616:bool)
                    }
                  }
                  frame #2 {
                    n119 = local read "Looper"() -> (w653:bool)
                    n120 = case shown="False" w653 {
                      tunnel: w651 -> [w657 _]
                      tunnel: w650 -> [_ w665]
                      tunnel: ["This is an acceptable entry." "ERROR: A bubble will intersect the buffer zone."] -> w652
                      tunnel: [w657 w665] -> w649
                      frame False {
                        n121 = local write "Looper"(FALSE) -> ()
                        n122 = local read "Current Spot #"() -> (w658:dbl)
                        n123 = Index Array(array=w657, index=w658) -> (element=w656:T1)
                        n124 = Unbundle By Name(w656) -> ("Position.x"=w655:dbl, "Position.y"=w654:dbl)
                        n125 = local write "New Y"(w654) -> ()
                        n126 = local write "New X"(w655) -> ()
                      }
                      frame True {
                        # "Restore original position"
                        n127 = local write "Looper"(FALSE) -> ()
                        n128 = local read "Old Y"() -> (w662:dbl)
                        n129 = local read "Old X"() -> (w663:dbl)
                        n130 = local read "Position"() -> (w661:cluster{"x":dbl, "y":dbl, "z":dbl})
                        n131 = Bundle By Name(cluster=w661, "x"=w663, "y"=w662) -> (w664:cluster{"x":dbl, "y":dbl, "z":dbl})
                        n132 = local write "Position"(w664) -> ()
                      }
                    }
                  }
                }
                "Position Indicator" <- w580
              }
              event "Size": Value Change {
                # "If we were constraining the aspect ratio, or preventing a divide by zero, the size control on the FP may be incorrect.  We refresh it in here to stop it displaying a wrong value."
                # "If the size has changed, scale the spots"
                n133 = event-data() -> ("OldVal"=w674:cluster{"x":dbl, "y":dbl, "z":dbl}, "NewVal"=w680:cluster{"x":dbl, "y":dbl, "z":dbl})  [unwired: 5 out]
                n134 = Not Equal?(x=w674, y=w680) -> (x != y?=w673:cluster{"x":bool, "y":bool, "z":bool})
                n135 = Divide(x=w680, y=w674) -> (x/y=w679:cluster{"x":dbl, "y":dbl, "z":dbl})
                n136 = Not Equal To 0?(x=w674) -> (x != 0?=w672:cluster{"x":bool, "y":bool, "z":bool})
                n137 = And(x=w673, y=w672) -> (x .and. y?=w671:cluster{"x":bool, "y":bool, "z":bool})
                n138 = Cluster To Array(cluster=w671) -> (array=w678:bool[])
                n139 = Cluster To Array(cluster=w679) -> (array=w677:dbl[])
                n140 = case shown="True" "lock aspect ratio" {
                  tunnel: w678 -> [w686 w703]
                  tunnel: w677 -> [w685 w701]
                  tunnel: [w683 w693] -> w676
                  frame False {
                    # "We are not constraining the aspect ratio here, so just check we're not introducing NAs"
                    n141 = for {
                      tunnel: w686 -> [w692] mode=indexing
                      tunnel: w685 -> [w688] mode=indexing
                      tunnel: [w690] -> w684 mode=indexing
                      n142 = Not A Number/Path/Refnum?(number/path/refnum=w688) -> (NaN/Path/Refnum?=w689:bool)
                      n143 = Compound Arithmetic op=AND(w692, invert w689) -> (w691:bool)
                      n144 = Select(t=w688, s=w691, f=1.0) -> (s? t:f=w690:dbl)
                    }
                    n145 = Array To Cluster(array=w684) -> (cluster=w683:cluster{"[0]":dbl, "[1]":dbl, "[2]":dbl})
                  }
                  frame True {
                    # "Pick the first element that changed and use it.  Also need to make sure (1) an element did change and (2) everything's valid (no divide by zeros)"
                    n146 = Search 1D Array(1D array=w703, element=TRUE) -> (index of element=w700:i32)  [unwired: 1 in]
                    n147 = Index Array(array=w701, index=w700) -> (element=w696:dbl)
                    n148 = Not A Number/Path/Refnum?(number/path/refnum=w696) -> (NaN/Path/Refnum?=w699:bool)
                    n149 = Less Than 0?(x=w700) -> (x < 0?=w698:bool)
                    n150 = Or(x=w699, y=w698) -> (x .or. y?=w697:bool)
                    n151 = Select(t=1.0, s=w697, f=w696) -> (s? t:f=w694:dbl)
                    n152 = Bundle("x"=w694, "x"=w694, "x"=w694) -> (w693:cluster{"x":dbl, "x":dbl, "x":dbl})  [unwired: 1 in]
                  }
                }
                n153 = for {
                  tunnel: w682 -> [w709] mode=indexing
                  tunnel: w669 -> [w706] mode=indexing
                  tunnel: [w708] -> w670 mode=indexing
                  tunnel: w676 -> [w707]
                  tunnel: w681 -> [w704]
                  n154 = Unbundle(w706) -> ("Selected"=w705:bool)  [unwired: 1 out]
                  n155 = case shown="True" w705 {
                    tunnel: w709 -> [w710 w718]
                    tunnel: [w710 w717] -> w708
                    tunnel: w707 -> [_ w716]
                    tunnel: w704 -> [_ w712]
                    frame False {
                    }
                    frame True {
                      n156 = call "extract_position.vi"("Spot"=w718) -> ("Position"=w714:cluster{"x":dbl, "y":dbl, "z":dbl})
                      n157 = Subtract(x=w714, y=w712) -> (x-y=w715:cluster{"x":dbl, "y":dbl, "z":dbl})
                      n158 = Multiply(x=w715, y=w716) -> (x*y=w713:cluster{"x":dbl, dbl, dbl})
                      n159 = Add(x=w712, y=w713) -> (x+y=w711:cluster{"x":dbl, dbl, dbl})
                      n160 = call "replace_position.vi"("Position"=w711, "Spot in"=w718) -> ("Spot"=w717:T1)  [unwired: 2 out]
                    }
                  }
                }
                n161 = call "find_centroid.vi"("Selection and Groups"=w669, "Spots"=w670) -> ("size"=w668:cluster{"x":dbl, "y":dbl, "z":dbl})  [unwired: 2 in, 4 out]
                n162 = local write "Size"(w668) -> ()
              }
              event "Intensity": Value Change {
                # "When  the user changes intensity, scale all the spots selected so the new mean is correct but keep the ratio between the selected spots.\n\nThe exception to this is when the mean intensity is zero, in which case multiplying makes no sense- in that case we just replace with the new value."
                n163 = event-data() -> ("NewVal"=w719:dbl, "OldVal"=w726:dbl)  [unwired: 5 out]
                n164 = Equal To 0?(x=w726) -> (x = 0?=w722:bool)
                n165 = Not A Number/Path/Refnum?(number/path/refnum=w726) -> (NaN/Path/Refnum?=w721:bool)
                n166 = Or(x=w722, y=w721) -> (x .or. y?=w720:bool)
                n167 = Divide(x=w719, y=w726) -> (x/y=w723:dbl)
                n168 = for {
                  tunnel: w727 -> [w732] mode=indexing
                  tunnel: w724 -> [w734] mode=indexing
                  tunnel: [w731] -> w725 mode=indexing
                  tunnel: w723 -> [w730]
                  tunnel: w720 -> [w729]
                  tunnel: w719 -> [w728]
                  n169 = Unbundle(w734) -> ("Selected"=w733:bool)  [unwired: 1 out]
                  n170 = case shown="True" w733 {
                    tunnel: w732 -> [w735 w742]
                    tunnel: [w735 w739] -> w731
                    tunnel: w730 -> [_ w738]
                    tunnel: w729 -> [_ w737]
                    tunnel: w728 -> [_ w736]
                    frame False {
                    }
                    frame True {
                      n171 = Unbundle By Name(w742) -> ("Intensity"=w740:dbl)
                      n172 = case shown="True" w737 {
                        tunnel: [w745 w746] -> w741
                        tunnel: w740 -> [w744 _]
                        tunnel: w738 -> [w743 _]
                        tunnel: w736 -> [_ w746]
                        frame False {
                          n173 = Multiply(x=w744, y=w743) -> (x*y=w745:dbl)
                        }
                        frame True {
                        }
                      }
                      n174 = Bundle By Name(cluster=w742, "Intensity"=w741) -> (w739:T1)
                    }
                  }
                }
              }
              event "phase": Value Change {
                # "When  the user changes phase, translate the phase of all spots selectedd"
                n175 = event-data() -> ("NewVal"=w748:dbl, "OldVal"=w752:dbl)  [unwired: 5 out]
                n176 = Not A Number/Path/Refnum?(number/path/refnum=w752) -> (NaN/Path/Refnum?=w747:bool)
                n177 = Subtract(x=w748, y=w752) -> (x-y=w749:dbl)
                n178 = for {
                  tunnel: w753 -> [w758] mode=indexing
                  tunnel: w750 -> [w760] mode=indexing
                  tunnel: [w757] -> w751 mode=indexing
                  tunnel: w749 -> [w756]
                  tunnel: w747 -> [w755]
                  tunnel: w748 -> [w754]
                  n179 = Unbundle(w760) -> ("Selected"=w759:bool)  [unwired: 1 out]
                  n180 = case shown="False" w759 {
                    tunnel: w758 -> [w761 w768]
                    tunnel: [w761 w765] -> w757
                    tunnel: w756 -> [_ w764]
                    tunnel: w755 -> [_ w763]
                    tunnel: w754 -> [_ w762]
                    frame False {
                    }
                    frame True {
                      n181 = Unbundle By Name(w768) -> ("Phase"=w766:dbl)
                      n182 = case shown="False" w763 {
                        tunnel: [w771 w772] -> w767
                        tunnel: w766 -> [w770 _]
                        tunnel: w764 -> [w769 _]
                        tunnel: w762 -> [_ w772]
                        frame False {
                          n183 = Add(x=w770, y=w769) -> (x+y=w771:dbl)
                        }
                        frame True {
                        }
                      }
                      n184 = Bundle By Name(cluster=w768, "Phase"=w767) -> (w765:T1)
                    }
                  }
                }
              }
              event "Vortex Charge": Value Change {
                # "When  the user changes l, just set all selected spots to have that value of l."
                n185 = event-data() -> ("NewVal"=w773:i8)  [unwired: 6 out]
                n186 = for {
                  tunnel: w776 -> [w779] mode=indexing
                  tunnel: w774 -> [w781] mode=indexing
                  tunnel: [w778] -> w775 mode=indexing
                  tunnel: w773 -> [w777]
                  n187 = Unbundle(w781) -> ("Selected"=w780:bool)  [unwired: 1 out]
                  n188 = case shown="True" w780 {
                    tunnel: w779 -> [w782 w785]
                    tunnel: [w782 w784] -> w778
                    tunnel: w777 -> [_ w783]
                    frame False {
                    }
                    frame True {
                      n189 = Bundle By Name(cluster=w785, "Vortex Charge"=w783) -> (w784:T1)
                    }
                  }
                }
              }
            }
          }
          frame "Spot Shape" {
            # "We update the spot shape tab only when spots have changed OUTSIDE this tab.  This avoids unnecessary jumping about of the tab control."
            n190 = call "find_centroid.vi"("Selection and Groups"=w796, "Spots"=w797) -> ("Mean Values"=w792:T1)  [unwired: 2 in, 4 out]
            n191 = Wait (ms)(milliseconds to wait=u32 10) -> ()  [unwired: 1 out]
            n192 = call "spots_shape.vi"("Selection and Groups"=w796, "Spots"=w797) -> ("Spot Shape"=w799:enum32{"Normal", "Line", "NA", "Mixed"})  [unwired: 7 in]
            n193 = feedback-in #4(w792) -> ()
            n194 = feedback #4() -> (w793:T1)  [unwired: 1 in]
            n195 = Not Equal?(x=w793, y=w792) -> (x != y?=w798:bool)
            n196 = feedback #5() -> (w788:enum32{"Normal", "Line", "NA", "Mixed"})  [unwired: 1 in]
            n197 = feedback #6() -> (w790:T1)  [unwired: 1 in]
            n198 = Not Equal?(x=w790, y=w792) -> (x != y?=w789:bool)
            n199 = case shown="False" w789 {
              tunnel: w799 -> [_ w918]
              tunnel: ["Spot Shape" w918] -> w787
              frame False {
              }
              frame True {
                n200 = local write "Spot Shape"(w918) -> ()
              }
            }
            n201 = feedback-in #5(w787) -> ()
            n202 = Not Equal?(x=w787, y=w788) -> (x != y?=w786:bool)
            n203 = case shown="\"Normal\", Default" w787 {
              tunnel: w797 -> [w803 w820 w846 w916]
              tunnel: w796 -> [w802 w819 w845 w915]
              tunnel: [w802 w818 w843 w915] -> w794
              tunnel: [w801 w817 w844 w916] -> w795
              tunnel: w792 -> [_ w816 w842 _]
              tunnel: w798 -> [_ w815 w841 _]
              tunnel: w786 -> [_ w813 w839 _]
              frame "Normal", Default {
                # "If \"normal\" is selected, don't allow any NA or line-trapping stuff"
                n204 = for {
                  tunnel: w803 -> [w806] mode=indexing
                  tunnel: w802 -> [w805] mode=indexing
                  tunnel: [w807] -> w801 mode=indexing
                  n205 = Unbundle(w805) -> ("Selected"=w804:bool)  [unwired: 1 out]
                  n206 = case shown="True" w804 {
                    tunnel: [w808 w812] -> w807
                    tunnel: w806 -> [w808 w811]
                    frame False {
                    }
                    frame True {
                      n207 = Bundle By Name(cluster=w811, "NA Position"=cluster{"x":dbl, "y":dbl, "r":dbl} {"x"=0.0, "y"=0.0, "r"=1.0} ("x"), "Line Trapping"=T2 {"Vector"={"x"=0.0, "y"=0.0, "z"=0.0}, "Phase Gradient"=0.0}) -> (w812:T1)
                    }
                  }
                }
              }
              frame "Line" {
                # "If it's out of date, update front panel"
                n208 = Or(x=w815, y=w813) -> (x .or. y?=w814:bool)
                n209 = case shown="True" w814 {
                  tunnel: w816 -> [_ w823]
                  frame False {
                  }
                  frame True {
                    n210 = Unbundle By Name(w823) -> ("Line Trapping"=w822:T2)
                    n211 = local write "Line Trapping"(w822) -> ()
                  }
                }
                n212 = event shown="[1] \"Line Trapping\": Value Change" {
                  selector: _ -> [_ _]
                  dyn-events: _ -> [_ _]
                  timeout: 10 -> [_ _]
                  tunnel: w820 -> [w825 w829]
                  tunnel: w819 -> [w824 w827]
                  tunnel: [w825 w828] -> w817
                  tunnel: [w824 w827] -> w818
                  event Timeout {
                    n213 = event-data() -> ()  [unwired: 3 out]
                  }
                  event Value Change {
                    # "If the line vector has changed, update it"
                    n214 = event-data() -> ("NewVal"=w826:T2)  [unwired: 6 out]
                    n215 = for {
                      tunnel: w829 -> [w834] mode=indexing
                      tunnel: w827 -> [w831] mode=indexing
                      tunnel: [w833] -> w828 mode=indexing
                      tunnel: w826 -> [w832]
                      n216 = Unbundle(w831) -> ("Selected"=w830:bool)  [unwired: 1 out]
                      n217 = case shown="True" w830 {
                        tunnel: w834 -> [w835 w837]
                        tunnel: [w835 w838] -> w833
                        tunnel: w832 -> [_ w836]
                        frame False {
                        }
                        frame True {
                          n218 = Bundle By Name(cluster=w837, "Line Trapping"=w836) -> (w838:T1)
                        }
                      }
                    }
                  }
                }
              }
              frame "NA" {
                n219 = Or(x=w839, y=w841) -> (x .or. y?=w840:bool)
                n220 = case shown="True" w840 {
                  tunnel: w842 -> [_ w851]
                  frame False {
                  }
                  frame True {
                    n221 = Unbundle By Name(w851) -> ("NA Position"=w850:cluster{"x":dbl, "y":dbl, "r":dbl})
                    n222 = call "xyz_to_xy.vi"("Position"=w850) -> ("Position (2D)"=w849:cluster{"x":dbl, "y":dbl}, "z"=w848:dbl)  [unwired: 6 out]
                    n223 = local write "Position on back aperture"(w849) -> ()
                    n224 = local write "Radius on back aperture"(w848) -> ()
                  }
                }
                n225 = event shown="[3] \"Scale BA\": Value Change" {
                  selector: _ -> [_ _ _ _]
                  dyn-events: _ -> [_ _ _ _]
                  timeout: 10 -> [_ _ _ _]
                  tunnel: w846 -> [w853 w859 w880 w902]
                  tunnel: w845 -> [w852 w857 w877 w903]
                  tunnel: [w853 w858 w878 w900] -> w844
                  tunnel: [w852 w857 w877 w903] -> w843
                  event Timeout {
                    n226 = event-data() -> ()  [unwired: 3 out]
                  }
                  event "Position on back aperture": Value Change {
                    # "If the position has changed, translate the spots"
                    n227 = event-data() -> ("OldVal"=w855:cluster{"x":dbl, "y":dbl}, "NewVal"=w856:cluster{"x":dbl, "y":dbl})  [unwired: 5 out]
                    n228 = Subtract(x=w856, y=w855) -> (x-y=w854:cluster{"x":dbl, "y":dbl})
                    n229 = for {
                      tunnel: w859 -> [w864] mode=indexing
                      tunnel: w857 -> [w861] mode=indexing
                      tunnel: [w863] -> w858 mode=indexing
                      tunnel: w854 -> [w862]
                      n230 = Unbundle(w861) -> ("Selected"=w860:bool)  [unwired: 1 out]
                      n231 = case shown="True" w860 {
                        tunnel: w864 -> [w865 w867]
                        tunnel: [w865 w868] -> w863
                        tunnel: w862 -> [_ w869]
                        frame False {
                        }
                        frame True {
                          n232 = Unbundle By Name(w867) -> ("NA Position"=w871:cluster{"x":dbl, "y":dbl, "r":dbl})
                          n233 = call "xy_to_xyz.vi"("Position (2D)"=w869) -> ("Position (3D)"=w870:cluster{dbl, dbl, dbl})  [unwired: 1 in, 2 out]
                          n234 = Add(x=w871, y=w870) -> (x+y=w866:cluster{dbl, dbl, dbl})
                          n235 = Bundle By Name(cluster=w867, "NA Position"=w866) -> (w868:T1)
                        }
                      }
                    }
                  }
                  event "Radius on back aperture": Value Change {
                    # "When  the user changes intensity, scale all the spots selected so the new mean is correct but keep the ratio between the selected spots.\n\nThe exception to this is when the mean intensity is zero, in which case multiplying makes no sense- in that case we just replace with the new value."
                    n236 = event-data() -> ("NewVal"=w872:dbl, "OldVal"=w879:dbl)  [unwired: 5 out]
                    n237 = Equal To 0?(x=w879) -> (x = 0?=w875:bool)
                    n238 = Not A Number/Path/Refnum?(number/path/refnum=w879) -> (NaN/Path/Refnum?=w874:bool)
                    n239 = Or(x=w875, y=w874) -> (x .or. y?=w873:bool)
                    n240 = Divide(x=w872, y=w879) -> (x/y=w876:dbl)
                    n241 = for {
                      tunnel: w880 -> [w885] mode=indexing
                      tunnel: w877 -> [w887] mode=indexing
                      tunnel: [w884] -> w878 mode=indexing
                      tunnel: w876 -> [w883]
                      tunnel: w873 -> [w882]
                      tunnel: w872 -> [w881]
                      n242 = Unbundle(w887) -> ("Selected"=w886:bool)  [unwired: 1 out]
                      n243 = case shown="True" w886 {
                        tunnel: w885 -> [w888 w895]
                        tunnel: [w888 w892] -> w884
                        tunnel: w883 -> [_ w891]
                        tunnel: w882 -> [_ w890]
                        tunnel: w881 -> [_ w889]
                        frame False {
                        }
                        frame True {
                          n244 = Unbundle By Name(w895) -> ("NA Position.r"=w893:dbl)
                          n245 = case shown="False" w890 {
                            tunnel: [w898 w899] -> w894
                            tunnel: w893 -> [w897 _]
                            tunnel: w891 -> [w896 _]
                            tunnel: w889 -> [_ w899]
                            frame False {
                              n246 = Multiply(x=w897, y=w896) -> (x*y=w898:dbl)
                            }
                            frame True {
                            }
                          }
                          n247 = Bundle By Name(cluster=w895, "NA Position.r"=w894) -> (w892:T1)
                        }
                      }
                    }
                  }
                  event "Scale BA": Value Change {
                    n248 = event-data() -> ()  [unwired: 7 out]
                    n249 = for {
                      tunnel: w903 -> [w908] mode=indexing
                      tunnel: w902 -> [w906] mode=indexing
                      tunnel: "Scale back aperture" -> [w905]
                      tunnel: [w904] -> w900 mode=indexing
                      n250 = Unbundle(w908) -> ("Selected"=w907:bool)  [unwired: 1 out]
                      n251 = case shown="True" w907 {
                        tunnel: w906 -> [w909 w910]
                        tunnel: w905 -> [_ w913]
                        tunnel: [w909 w911] -> w904
                        frame False {
                        }
                        frame True {
                          n252 = Unbundle By Name(w910) -> ("NA Position"=w914:cluster{"x":dbl, "y":dbl, "r":dbl})
                          n253 = Multiply(x=w913, y=w914) -> (x*y=w912:cluster{"x":dbl, "y":dbl, "r":dbl})
                          n254 = Bundle By Name(cluster=w910, "NA Position"=w912) -> (w911:T1)
                        }
                      }
                    }
                  }
                }
              }
              frame "Mixed" {
              }
            }
            n255 = call "find_centroid.vi"("Selection and Groups"=w794, "Spots"=w795) -> ("Mean Values"=w791:T1)  [unwired: 2 in, 4 out]
            n256 = feedback-in #6(w791) -> ()
          }
          frame "Rotate" {
            w929 = u32 0 items=["Frame", "Fill", "Highlight"] ("Drawing Mode")
            w928 = u32 0 ("Color")
            w925 = i16 100 ("radius")
            # "It's necessary to check this has changed to stop us unintentionally \"spinning\" the spots..."
            # "Draw the centroid as a spot, then a large circle+cross"
            # "It's important that this loop doesn't go too fast- it hogs the CPU.  However, each tab can have a different loop speed."
            n257 = Unbundle By Name(w922) -> ("Position (Image Pixels)"=w938:cluster{"X":dbl, "Y":dbl}, "Previous Position (Image Pixels)"=w937:cluster{"X":dbl, "Y":dbl}, "Dragging"=w939:bool)
            n258 = feedback-in #7(w922) -> ()
            n259 = feedback #7() -> (w923:T10)  [unwired: 1 in]
            n260 = call "find_centroid.vi"("Selection and Groups"=w940, "Spots"=w943) -> ("centroid"=w936:cluster{"x":dbl, "y":dbl, "z":dbl})  [unwired: 2 in, 4 out]
            n261 = Not Equal?(x=w922, y=w923) -> (x != y?=w920:bool)
            n262 = Wait (ms)(milliseconds to wait=u32 10) -> ()  [unwired: 1 out]
            n263 = And(x=w920, y=w939) -> (x .and. y?=w921:bool)
            n264 = call "coords_real_to_image_currentview.vi"("Position (real coords)"=w936) -> ("Position (pixels, relative to the top left of the image)"=w919:cluster{dbl, dbl})  [unwired: 7 in, 1 out]
            n265 = case shown="True" w921 {
              tunnel: w943 -> [w952 w996]
              tunnel: [w954 w995] -> w942
              tunnel: w940 -> [w953 w997]
              tunnel: [w953 w997] -> w941
              tunnel: w936 -> [w951 w988]
              tunnel: w938 -> [_ w987]
              tunnel: w937 -> [_ w986]
              tunnel: w919 -> [_ w985]
              frame False {
                n266 = event shown="[1] Timeout" {
                  selector: _ -> [_ _]
                  dyn-events: _ -> [_ _]
                  timeout: 10 -> [_ _]
                  tunnel: [w967 w984] -> w954
                  tunnel: w953 -> [w966 _]
                  tunnel: w952 -> [w965 w984]
                  tunnel: w951 -> [w961 _]
                  event "rotate": Value Change {
                    n267 = event-data() -> ()  [unwired: 6 out]
                    n268 = case shown="3" "Rotation Axis" {
                      tunnel: [cluster{dbl, dbl, dbl} {0.0, 0.0, 1.0} ("Custom Axis") cluster{dbl, dbl, dbl} {1.0, 0.0, 0.0} ("Custom Axis") cluster{dbl, dbl, dbl} {0.0, 1.0, 0.0} ("Custom Axis") "Custom Axis"] -> w962
                      frame 0, Default {
                        # "Z"
                      }
                      frame 1 {
                        # "X"
                      }
                      frame 2 {
                        # "Y"
                      }
                      frame 3 {
                      }
                    }
                    n269 = call "normalise_3d_vector.vi"("Vector"=w962) -> ("Unit Vector"=w964:cluster{dbl, dbl, dbl})  [unwired: 3 out]
                    n270 = Divide(x=6.283185307179586, y=360.0) -> (x/y=w959:dbl)
                    n271 = Multiply(x="Angle (degrees)", y=w959) -> (x*y=w956:dbl)
                    n272 = call "arb_rotation_matrix.vi"("Unit Vector"=w964, "theta"=w956) -> ("Real Matrix"=w968:T17)
                    n273 = for {
                      tunnel: w966 -> [w978] mode=indexing
                      tunnel: w965 -> [w973] mode=indexing
                      tunnel: [w974] -> w967 mode=indexing
                      tunnel: w961 -> [w976]
                      tunnel: w968 -> [w975]
                      n274 = Unbundle(w978) -> ("Selected"=w977:bool)  [unwired: 1 out]
                      n275 = case shown="True" w977 {
                        tunnel: w976 -> [_ w983]
                        tunnel: [w979 w982] -> w974
                        tunnel: w973 -> [w979 w981]
                        tunnel: w975 -> [_ w980]
                        frame False {
                        }
                        frame True {
                          n276 = call "apply_matrix_transformation_to_spots.vi"("Transform centre (i.e. transform about this point)"=w983, "Transformation Matrix (3x3)"=w980, "Spot In"=w981) -> ("Spot Out"=w982:T1)  [unwired: 5 out]
                        }
                      }
                    }
                  }
                  event Timeout {
                    n277 = event-data() -> ()  [unwired: 4 out]
                  }
                }
              }
              frame True {
                # "if the mouse has not moved, stuff will be NaN, so let's make like a leopard and not change our spots"
                # "the magnitude of the change in our direction vector gives the rotation angle in radians"
                # "If it's within 100px of the centroid, pretend the mouse is on the surface of a sphere, and synthesize Z accordingly (z^2=100^2-x^2-y^2).  This allows rotation in 3d :)  The output should always be a unit vector."
                n278 = Build Array(w987, w986) -> (w1002:cluster{"X":dbl, "Y":dbl}[])
                n279 = for {
                  tunnel: w985 -> [w1035]
                  tunnel: w1002 -> [w1031] mode=indexing
                  tunnel: [w1021] -> w1001 mode=indexing
                  n280 = Subtract(x=w1031, y=w1035) -> (x-y=w1026:cluster{dbl, dbl})
                  n281 = Divide(x=w1026, y=100.0 ("x")) -> (x/y=w1027:cluster{dbl, dbl})
                  n282 = Square(x=w1027) -> (x^2=w1034:cluster{dbl, dbl})
                  n283 = Unbundle(w1034) -> (w1032:dbl, w1033:dbl)
                  n284 = Add(x=w1032, y=w1033) -> (x+y=w1023:dbl)
                  n285 = Subtract(x=1.0, y=w1023) -> (x-y=w1029:dbl)
                  n286 = Square Root(x=w1023) -> (sqrt(x)=w1024:dbl)
                  n287 = Greater Than 0?(x=w1029) -> (x > 0?=w1030:bool)
                  n288 = case shown="False" w1030 {
                    tunnel: w1029 -> [_ w1042]
                    tunnel: [0.0 w1041] -> w1020
                    tunnel: w1027 -> [w1039 w1040]
                    tunnel: w1024 -> [w1038 _]
                    tunnel: [w1037 w1040] -> w1022
                    frame False {
                      n289 = Divide(x=w1039, y=w1038) -> (x/y=w1037:cluster{dbl, dbl})
                    }
                    frame True {
                      n290 = Square Root(x=w1042) -> (sqrt(x)=w1041:dbl)
                    }
                  }
                  n291 = call "xy_to_xyz.vi"("z"=w1020, "Position (2D)"=w1022) -> ("Position (3D)"=w1021:cluster{dbl, dbl, dbl})  [unwired: 2 out]
                }
                n292 = Index Array(array=w1001) -> (element #1=w1000:cluster{dbl, dbl, dbl}, element #2=w991:cluster{dbl, dbl, dbl})  [unwired: 2 in]
                n293 = Add(x=w1000, y=w991) -> (x+y=w990:cluster{dbl, dbl, dbl})
                n294 = Subtract(x=w1000, y=w991) -> (x-y=w989:cluster{dbl, dbl, dbl})
                n295 = call "cross_product.vi"("b"=w990, "a"=w989) -> ("a cross b"=w999:cluster{dbl, dbl, dbl})
                n296 = call "normalise_3d_vector.vi"("Vector"=w999) -> ("Unit Vector"=w998:cluster{dbl, dbl, dbl})  [unwired: 3 out]
                n297 = call "normalise_3d_vector.vi"("Vector"=w989) -> ("magnitude"=w993:dbl)  [unwired: 3 out]
                n298 = Not Equal To 0?(x=w993) -> (x != 0?=w992:bool)
                n299 = call "arb_rotation_matrix.vi"("Unit Vector"=w998, "theta"=w993) -> ("Real Matrix"=w994:T17)
                n300 = case shown="True" w992 {
                  tunnel: w997 -> [_ w1008]
                  tunnel: w996 -> [w1003 w1007]
                  tunnel: [w1003 w1006] -> w995
                  tunnel: w994 -> [_ w1005]
                  tunnel: w988 -> [_ w1004]
                  frame False {
                  }
                  frame True {
                    n301 = for {
                      tunnel: w1008 -> [w1014] mode=indexing
                      tunnel: w1007 -> [w1011] mode=indexing
                      tunnel: [w1010] -> w1006 mode=indexing
                      tunnel: w1005 -> [w1012]
                      tunnel: w1004 -> [w1009]
                      n302 = Unbundle(w1014) -> ("Selected"=w1013:bool)  [unwired: 1 out]
                      n303 = case shown="True" w1013 {
                        tunnel: [w1015 w1018] -> w1010
                        tunnel: w1011 -> [w1015 w1019]
                        tunnel: w1012 -> [_ w1016]
                        tunnel: w1009 -> [_ w1017]
                        frame False {
                        }
                        frame True {
                          n304 = call "apply_matrix_transformation_to_spots.vi"("Transform centre (i.e. transform about this point)"=w1017, "Transformation Matrix (3x3)"=w1016, "Spot In"=w1019) -> ("Spot Out"=w1018:T1)  [unwired: 5 out]
                        }
                      }
                    }
                  }
                }
              }
            }
            n305 = call "coords_real_to_image_currentview.vi"("Position (real coords)"=w936) -> ("Position (pixels, relative to the top left of the image)"=w931:cluster{dbl, dbl}, "z (real coords)"=w935:dbl)  [unwired: 7 in]
            n306 = expression code="z*1e7+20"(w935) -> (w947:dbl)
            n307 = In Range and Coerce(upper limit=100.0, x=w947, lower limit=2.0) -> (coerced(x)=w934:dbl)  [unwired: 1 out]
            n308 = Bundle("upper limit"=w934, "upper limit"=w934) -> (w927:cluster{"upper limit":dbl, "upper limit":dbl})  [unwired: 1 in]
            n309 = call "myoverlay_oval.vi"("Color"=w928, "Drawing Mode"=w929, "Size"=w927, "Centre Position (pixels on image)"=w931) -> ("Overlay Elements Out"=w933:T18[])  [unwired: 5 in]
            n310 = Bundle("radius"=w925, "radius"=w925) -> (w926:cluster{"radius":i16, "radius":i16})  [unwired: 1 in]
            n311 = call "myoverlay_oval.vi"("Color"=w928, "Drawing Mode"=w929, "Size"=w926, "Centre Position (pixels on image)"=w931, "Overlay Elements In"=w933) -> ("Overlay Elements Out"=w932:T18[])  [unwired: 4 in]
            n312 = Multiply(x=w925, y=cluster{dbl, dbl}[] [{0.0, 0.0}, {1.0, 0.0}, {0.0, 0.0}, {0.0, 1.0}, {0.0, 0.0}, {-1.0, 0.0}, {0.0, 0.0}, {0.0, -1.0}, {0.0, 0.0}]) -> (x*y=w944:cluster{dbl, dbl}[])
            n313 = Add(x=w931, y=w944) -> (x+y=w930:cluster{dbl, dbl}[])
            n314 = call "myoverlay_lines.vi"("Color"=w928, "Drawing Mode"=w929, "Line Endpoints"=w930, "Overlay Elements In"=w932) -> ("Overlay Elements Out"=w924:T18[])  [unwired: 5 in]
          }
          frame "Patterns" {
            n315 = event shown="[3] \"Optimise\": Value Change" {
              selector: _ -> [_ _ _ _ _]
              dyn-events: _ -> [_ _ _ _ _]
              timeout: u32 10 ("milliseconds to wait") -> [_ _ _ _ _]
              tunnel: [w1061 w1091 w1095 w1098 w1109] -> w1044
              tunnel: [w1060 w1092 w1094 w1101 w1110] -> w1043
              tunnel: w1046 -> [w1059 w1091 w1095 w1099 w1108]
              tunnel: w1045 -> [w1058 w1092 w1094 w1101 w1110]
              event "Generate": Value Change {
                # "If there were previous spots, centre the pattern on the spots"
                n316 = event-data() -> ()  [unwired: 1 in, 1 out]
                n317 = call "find_centroid.vi"("Selection and Groups"=w1058, "Spots"=w1059) -> ("size"=w1054:cluster{"x":dbl, "y":dbl, "z":dbl}, "centroid"=w1050:cluster{"x":dbl, "y":dbl, "z":dbl}, "# selected"=w1056:i16)  [unwired: 2 in, 2 out]
                n318 = Greater?(x=w1056, y=i16 1) -> (0:w1051:bool)
                n319 = case shown="False" w1051 {
                  tunnel: w1054 -> [_ w1077]
                  tunnel: [cluster{"x":dbl, "y":dbl, "z":dbl} {"x"=2e-05, "y"=2e-05, "z"=2e-05} ("size") w1077] -> w1053
                  frame False {
                  }
                  frame True {
                  }
                }
                n320 = case shown="\"HCP Shack-Hartmann\"" "Pattern" {
                  tunnel: [w1079 w1082 w1088] -> w1052
                  tunnel: w1053 -> [_ w1081 _]
                  frame "Square Shack-Hartmann" {
                    n321 = call "patterns_square_shack_hartmann.vi"("N"="Spots across centre") -> ("Spots"=w1079:T1[])
                  }
                  frame "HCP Shack-Hartmann" {
                    n322 = Unbundle By Name(w1081) -> ("x"=w1080:dbl)
                    n323 = call "pattern_hcp_shack_hartmann.vi"("Width"=w1080, "Reference Array?"="Reference Array?", "Fraction of SLM"="Fraction of SLM", "N"="Spots across centre") -> ("Shack-Hartmann Spots"=w1082:T1[])  [unwired: 7 in]
                  }
                  frame "Rectangular Grid" {
                    n324 = call "patterns_rectangular_grid.vi"("spacing/m"="spacing/m", "N"="N") -> ("Spots"=w1088:T1[])
                  }
                }
                n325 = local write "Generate"(FALSE ("Generate")) -> ()
                n326 = case shown="True" w1051 {
                  tunnel: w1052 -> [w1064 w1068]
                  tunnel: w1050 -> [_ w1070]
                  tunnel: [w1064 w1066] -> w1062
                  frame False {
                  }
                  frame True {
                    n327 = call "find_centroid.vi"("Spots"=w1068) -> ("centroid"=w1069:cluster{"x":dbl, "y":dbl, "z":dbl}, "# selected"=→"# selected":i16)  [unwired: 3 in, 3 out]
                    n328 = Subtract(x=w1070, y=w1069) -> (x-y=w1067:cluster{"x":dbl, "y":dbl, "z":dbl})
                    n329 = for {
                      tunnel: w1068 -> [w1073] mode=indexing
                      tunnel: w1067 -> [w1072]
                      tunnel: [w1071] -> w1066 mode=indexing
                      n330 = call "extract_position.vi"("Spot"=w1073) -> ("Position"=w1074:cluster{"x":dbl, "y":dbl, "z":dbl})
                      n331 = Add(x=w1074, y=w1072) -> (x+y=w1075:cluster{"x":dbl, "y":dbl, "z":dbl})
                      n332 = call "replace_position.vi"("Position"=w1075, "Spot in"=w1073) -> ("Spot"=w1071:T1)  [unwired: 2 out]
                    }
                  }
                }
                "Last Pattern" <- w1062
                n333 = call "ensure_selection_matches_spots.vi"("Select All (default: no)"=TRUE ("Select All (default: true)"), "Spots"=w1062) -> ("Selection and Groups out"=w1060:T7[], "Spots (duplicate)"=w1061:T1[])  [unwired: 4 in]
              }
              event "Spots across centre", "Fraction of SLM", "Reference Array?", "N", "spacing/m", "Spots across centre": Value Change {
                n334 = event-data() -> ()  [unwired: 1 in, 1 out]
                n335 = local read "Last Pattern"() -> (w1090:T1[])
                n336 = Equal?(x=w1091, y=w1090) -> (x = y?=w1089:bool)
                n337 = case shown="True" w1089 {
                  selector: w1089 -> [_ w1093]
                  frame False {
                  }
                  frame True {
                    n338 = property on="Generate" class="Bool (strict)"("Val(Sgnl)"=w1093) -> ()  [unwired: 2 in, 2 out]
                  }
                }
              }
              event Timeout {
                n339 = event-data() -> ()  [unwired: 1 in, 1 out]
              }
              event "Optimise": Value Change {
                n340 = event-data() -> ()  [unwired: 1 in, 1 out]
                n341 = for {
                  N: "Iterations" -> [_]
                  tunnel: 203 ("Optimisation Resolution") -> [w1105]
                  shift-right: [w1106] -> w1098
                  shift-left: w1099 -> [w1107]
                  tunnel: "Fall-off/m" -> [w1102]
                  n342 = call "do_gsw_step.vi"("Optimisation Resolution"=w1105, "Sinc Zero"=w1102, "Spots In"=w1107) -> ("non-uniformity"=→"non-uniformity":dbl, "efficiency"=→"efficiency":dbl, "Spots Out"=w1106:T1[])  [unwired: 6 in]
                }
              }
              event "Reset Phase/Amplitude": Value Change {
                n343 = event-data() -> ()  [unwired: 1 in, 1 out]
                n344 = for {
                  tunnel: [w1113] -> w1109 mode=indexing
                  tunnel: w1108 -> [w1114] mode=indexing
                  n345 = Bundle By Name(cluster=w1114, "Phase"=0.0, "Amplitude Correction"=0.0) -> (w1113:T1)
                }
              }
            }
          }
          frame "Plugins" {
            # "The local variable ensures the references are  correct when they make it through to the \"close plugins\" block."
            # "This is the error from loading/unloading VIs on the front panel"
            n346 = control-ref of="Plugin Pnl"() -> (w1118:refnum<vi>)
            n347 = Wait (ms)(milliseconds to wait=u32 10) -> ()  [unwired: 1 out]
            n348 = feedback #8() -> (w1117:T3)
            n349 = feedback #9() -> (w1119:errorcluster)
            n350 = event shown="[1] \"Plugin:\": Value Change" {
              selector: _ -> [_ _ _]
              dyn-events: _ -> [_ _ _]
              timeout: 10 -> [_ _ _]
              tunnel: "Abort Plugin" -> [w1126 _ _]
              tunnel: "Plugin:" -> [w1131 _ w1147]
              tunnel: w1119 -> [w1130 w1145 w1149]
              tunnel: [w1129 w1140 w1148] -> w1120
              tunnel: [w1128 w1141 w1151] -> w1116
              tunnel: w1117 -> [w1132 w1142 w1150]
              tunnel: w1118 -> [_ w1143 _]
              event Timeout {
                n351 = event-data() -> ()  [unwired: 1 in, 2 out]
                n352 = Not(x=w1126) -> (.not. x?=w1127:bool)
                n353 = case shown="True" w1127 {
                  tunnel: w1132 -> [w1134 w1139]
                  tunnel: w1131 -> [_ w1138]
                  tunnel: w1130 -> [w1133 w1137]
                  tunnel: [w1133 w1136] -> w1129
                  tunnel: [w1134 w1135] -> w1128
                  frame False {
                  }
                  frame True {
                    n354 = call "plugins_run.vi"("Error In"=w1137, "Plugin Index"=w1138, "Plugins In"=w1139) -> ("Error Out"=w1136:errorcluster, "Plugins"=w1135:T3)  [unwired: 7 in]
                  }
                }
              }
              event "Plugin:": Value Change {
                n355 = event-data() -> ("NewVal"=w1144:u16)  [unwired: 1 in]
                n356 = call "plugins_switch.vi"("error in"=w1145, "Plugin Pnl"=w1143, "Plugin Index"=w1144, "Plugins In"=w1142) -> ("error out"=w1140:errorcluster, "Plugins Out"=w1141:T3)  [unwired: 4 in]
              }
              event "Abort Plugin": Value Change {
                n357 = event-data() -> ("NewVal"=w1146:bool)  [unwired: 1 in]
                n358 = case shown="True" w1146 {
                  tunnel: [w1153 w1158] -> w1151
                  tunnel: w1150 -> [w1153 w1157]
                  tunnel: w1149 -> [w1152 w1156]
                  tunnel: [w1152 w1155] -> w1148
                  tunnel: w1147 -> [_ w1154]
                  frame False {
                  }
                  frame True {
                    n359 = call "plugins_abort.vi"("Error In"=w1156, "Plugin Index"=w1154, "Plugins In"=w1157) -> ("Error Out"=w1155:errorcluster, "Plugins Out"=w1158:T3)  [unwired: 7 in]
                  }
                }
              }
            }
            n360 = feedback-in #8(w1116) -> ()
            n361 = feedback-in #9(w1120) -> ()
            n362 = local write "Plugins"(w1116) -> ()
          }
          frame "Video" {
            # "All the controls on this tab are in the bottom (camera) loop."
            n363 = Wait (ms)(milliseconds to wait=u32 10) -> ()  [unwired: 1 out]
            n364 = property on="Property Node" class="ImageControl"(reference=w1159) -> ("Image Information String"=→"Image Information":string)  [unwired: 1 in, 2 out]
          }
        }
      }
      event "Tab": Value Change {
        w1167 = T19 [enum."Video", enum."Particle Tracking"] items=["Current Spot", "Rotate", "Spot Shape", "Patterns", "Plugins", "Video", "Particle Tracking", "Clamping", "Blank"]
        w1172 = refnum<vi> refnum  # Image
        # "This allows us to disable custom mouse-handling for certain tabs.  It can also be done from within the \"mouse down\" event case."
        n365 = event-data() -> ("NewVal"=w1168:T4)  [unwired: 1 in, 3 out]
        n366 = Equal?(x=w1167, y=w1168) -> (x = y?=w1166:bool[])
        n367 = Or Array Elements(Boolean array=w1166) -> (logical OR=w1165:bool)
        n368 = Not(x=w1165) -> (.not. x?=w1164:bool)
        n369 = Select(t=w1171, s=w1164, f=w1172) -> (s? t:f=w1173:refnum<vi>)
        n370 = register-events(reference=w1175, w1173, w1172, w1172, w1172) -> (reference out=w1174:refnum<event-registration>)  [unwired: 1 in, 1 out]
      }
      event Menu Selection (User) {
        n371 = event-data() -> ("ItemTag"=w1183:string, "MenuRef"=w1176:refnum<k9>)  [unwired: 1 in]
        n372 = case shown="\"ToggleSavingData\"" w1183 {
          tunnel: w1187 -> [w1191 w1201 w1210 w1224 w1243 w1247 w1250 w1257 w1264 w1266 w1269 w1298 w1324 w1345 w1356 w1367 w1370 w1372 w1377 w1380]
          tunnel: w1186 -> [w1190 w1200 w1209 w1233 w1242 w1246 w1248 w1255 w1263 w1265 w1268 w1297 w1323 w1344 w1355 w1366 w1369 w1373 w1378 w1379]
          tunnel: [w1191 w1201 w1210 w1224 w1241 w1244 w1250 w1257 w1264 w1266 w1269 w1298 w1324 w1345 w1356 w1367 w1370 w1372 w1377 w1380] -> w1185
          tunnel: [w1190 w1200 w1209 w1233 w1240 w1245 w1249 w1256 w1262 w1267 w1270 w1297 w1323 w1344 w1355 w1366 w1369 w1373 w1378 w1379] -> w1184
          tunnel: [_ _ _ _ TRUE _ _ _ _ _ _ _ _ _ _ _ _ _ _ _] -> w1178
          tunnel: w1177 -> [_ _ _ _ _ _ _ _ _ _ _ w1296 w1322 w1336 _ _ _ _ _ _]
          tunnel: w1176 -> [_ _ _ _ _ _ _ _ _ _ _ w1287 w1316 w1339 w1350 w1361 _ _ _ _]
          frame "ToggleSavingData" {
            # "Data is saved from the middle loop: look there for an explanation."
            n373 = local read "Save Video"() -> (w1189:bool)
            n374 = Not(x=w1189) -> (.not. x?=w1188:bool)
            n375 = local write "Save Video"(w1188) -> ()
          }
          frame "SaveStateToFile" {
            # "Save the current settings (i.e. the values of all the controls in VIs that have [Red Tweezers Save Settings] in their documentation string) to a file."
            n376 = call "File Dialog"("prompt"="Please select a location to save the settings", "button label"="Save", "default name"="red_tweezers_settings.xml", "pattern (all files)"="*.xml" ("pattern label"), "pattern label"="XML Settings Files") -> ("selected path"=w1199:path, "cancelled"=w1192:bool)  [unwired: 7 in, 2 out]
            n377 = Not(x=w1192) -> (.not. x?=w1193:bool)
            n378 = case shown="True" w1193 {
              tunnel: w1199 -> [_ w1203]
              frame False {
              }
              frame True {
                n379 = Path To String(path=w1203) -> (string=w1202:string)
                n380 = call "settings_save_to_file.vi"("XML File Path"=w1203) -> ()  [unwired: 11 in]
                n381 = call "settings_filename_to_registry.vi"("Last Used Settings File"=w1202) -> ()  [unwired: 11 in]
              }
            }
          }
          frame "SaveStateToCurrentFile" {
            # "As SaveStateToFile, but using the current file (i.e. Save not Save As...)."
            n382 = global read "red_tweezers_globals_INTERNAL_VOLATILE.vi" "Current Settings File"() -> (w1208:path)
            n383 = call <vilib>:"Check if File or Folder Exists.vi"("path"=w1208) -> ("file or folder exists?"=w1207:bool, "dup path"=w1206:path)  [unwired: 8 in, 1 out]
            n384 = case shown="True" w1207 {
              selector: w1207 -> [_ w1221]
              tunnel: w1206 -> [_ w1222]
              tunnel: [w1213 w1222] -> w1205
              tunnel: [w1214 w1221] -> w1204
              frame False {
                n385 = call "File Dialog3"("prompt"="Please select a location to save the settings", "button label"="Save", "default name"="red_tweezers_settings.xml", "pattern (all files)"="*.xml" ("pattern label"), "pattern label"="XML Settings Files") -> ("selected path"=w1213:path, "cancelled"=w1220:bool)  [unwired: 7 in, 2 out]
                n386 = Not(x=w1220) -> (.not. x?=w1214:bool)
              }
              frame True {
              }
            }
            n387 = case shown="True" w1204 {
              tunnel: w1205 -> [_ w1212]
              frame False {
              }
              frame True {
                n388 = Path To String(path=w1212) -> (string=w1211:string)
                n389 = call "settings_save_to_file.vi"("XML File Path"=w1212) -> ()  [unwired: 11 in]
                n390 = call "settings_filename_to_registry.vi"("Last Used Settings File"=w1211) -> ()  [unwired: 11 in]
              }
            }
          }
          frame "LoadStateFromFile" {
            # "Load a file, and use it to reset the values of all the front panel controls."
            # "We need to re-run the initialisation stuff in UDP sender after changing settings\n(for example, this synchronises the settings like camera pixel size with the\nrelevant global variable)"
            n391 = call "File Dialog2"("prompt"="Please select a settings file", "button label"="Open", "default name"="red_tweezers_settings.xml", "pattern (all files)"="*.xml" ("pattern label"), "pattern label"="XML Settings Files") -> ("selected path"=w1225:path, "cancelled"=w1232:bool)  [unwired: 7 in, 2 out]
            n392 = Not(x=w1232) -> (.not. x?=w1231:bool)
            n393 = case shown="False" w1231 {
              selector: w1231 -> [w1234 w1235]
              tunnel: w1225 -> [_ w1236]
              tunnel: [w1234 w1235] -> w1223
              frame False {
              }
              frame True {
                n394 = call "settings_load_from_file.vi"("XML File Path"=w1236) -> ()  [unwired: 9 in, 2 out]
                n395 = Path To String(path=w1236) -> (string=w1237:string)
                n396 = call "settings_filename_to_registry.vi"("Last Used Settings File"=w1237) -> ()  [unwired: 11 in]
              }
            }
            n397 = call "UDP Sender generic_2.vi"("re-initialise"=w1223, "Spots"=w1224) -> ()  [unwired: 1 in, 1 out]
          }
          frame "Undo" {
            # "This should get the last undo vector and replace the spots with it :)"
            n398 = call "red_tweezers_UNDO.vi"("Selection/Group"=w1242, "Undo/Store (store, False)"=TRUE, "Spots"=w1243) -> ("Selection/Group Out (Undo only)"=w1240:T7[], "Spots Out (Undo only)"=w1241:T1[])  [unwired: 7 in]
          }
          frame "Delete" {
            n399 = call "delete_selected_spots.vi"("Selection/Group 3"=w1246, "Spots 3"=w1247) -> ("Selection/Group 2"=w1245:T7[], "Spots 2"=w1244:T1[])  [unwired: 4 in]
          }
          frame "SelectAllSpots" {
            n400 = for {
              tunnel: w1248 -> [w1253] mode=indexing
              tunnel: [w1254] -> w1249 mode=indexing
              n401 = Unbundle(w1253) -> ("Group ID"=w1252:i32)  [unwired: 1 out]
              n402 = Bundle(cluster=w1253, "Group ID"=w1252, "Selected"=TRUE ("Label.Visible")) -> (w1254:T7)
            }
          }
          frame "SelectNoSpots" {
            n403 = for {
              tunnel: w1255 -> [w1260] mode=indexing
              tunnel: [w1261] -> w1256 mode=indexing
              n404 = Unbundle(w1260) -> ("Group ID"=w1259:i32)  [unwired: 1 out]
              n405 = Bundle(cluster=w1260, "Group ID"=w1259, "Selected"=FALSE ("Label.Visible")) -> (w1261:T7)
            }
          }
          frame "SelectSpecificSpots" {
            n406 = call "select_by_id.vi"("Selection/Group"=w1263, "Spots"=w1264) -> ("Selection/Group Out"=w1262:T7[])  [unwired: 9 in]
          }
          frame "Group" {
            # "Group the currently selected spots"
            n407 = call "group_selected_spots.vi"("Selection/Group 2"=w1265) -> ("Array"=w1267:T7[])
          }
          frame "Ungroup" {
            # "Ungroup the currently selected spots"
            n408 = for {
              tunnel: [w1274] -> w1270 mode=indexing
              tunnel: w1268 -> [w1273] mode=indexing
              tunnel: 0 -> [w1272]
              n409 = Unbundle(w1273) -> ("Selected"=w1275:bool)  [unwired: 1 out]
              n410 = case shown="False" w1275 {
                tunnel: [w1276 w1279] -> w1274
                tunnel: w1273 -> [w1276 w1278]
                tunnel: w1272 -> [_ w1277]
                frame False {
                }
                frame True {
                  n411 = Unbundle(w1278) -> ("Selected"=w1280:bool)  [unwired: 1 out]
                  n412 = Bundle(cluster=w1278, "Group ID"=w1277, "Selected"=w1280) -> (w1279:T7)
                }
              }
            }
          }
          frame "ZoomIn" {
            w1281 = "ZoomToFit" ("item tag")
            # "turn off \"zoom to fit\""
            n413 = property class="ImageControl"(reference=w1296) -> (reference out=w1290:refnum<vi>, "ZoomSingle"=w1295:cluster{"X":sgl, "Y":sgl}, "Image Center Position"=w1288:cluster{"X":u32, "Y":u32})  [unwired: 1 in, 1 out]
            n414 = Unbundle(w1295) -> ("X"=w1293:sgl)  [unwired: 1 out]
            n415 = Round To Nearest(number=w1293) -> (nearest integer value=w1289:sgl)
            n416 = Greater Than 0?(x=w1289) -> (x > 0?=w1294:bool)
            n417 = case shown="True" w1294 {
              tunnel: w1293 -> [w1303 w1306]
              tunnel: [w1302 w1304] -> w1292
              frame False {
                n418 = Reciprocal(x=w1303) -> (1/x=w1300:sgl)
                n419 = Round Toward +Infinity(x=w1300) -> (ceil(x): smallest int >= x=w1301:sgl)
                n420 = Decrement(x=w1301) -> (x-1=w1299:sgl)
                n421 = Reciprocal(x=w1299) -> (1/x=w1302:sgl)
              }
              frame True {
                n422 = Round Toward -Infinity(1:w1306) -> (0:w1305:sgl)
                n423 = Increment(x=w1305) -> (x+1=w1304:sgl)
              }
            }
            n424 = Bundle(w1292, w1292) -> (w1291:cluster{sgl, sgl})  [unwired: 1 in]
            n425 = property class="ImageControl"(reference=w1290, "ZoomSingle"=w1291, "Image Center Position"=w1288) -> ()  [unwired: 1 in, 2 out]
            n426 = Get Menu Item Info(7:w1281, 11:w1287) -> (1:w1284:bool, 2:w1285:string, 3:w1286:refnum<k9>, 6:w1283:T20)  [unwired: 1 in, 3 out]
            n427 = Set Menu Item Info(4:w1283, 6:FALSE ("checked"), 7:w1281, 9:w1284, 10:w1285, 11:w1286) -> ()  [unwired: 1 in, 2 out]
          }
          frame "ZoomOut" {
            w1310 = "ZoomToFit" ("item tag")
            # "turn off \"zoom to fit\""
            n428 = property class="ImageControl"(reference=w1322) -> (reference out=w1318:refnum<vi>, "ZoomSingle"=w1321:cluster{"X":sgl, "Y":sgl}, "Image Center Position"=w1317:cluster{"X":u32, "Y":u32})  [unwired: 1 in, 1 out]
            n429 = Unbundle(w1321) -> ("X"=w1307:sgl)  [unwired: 1 out]
            n430 = Greater?(x=w1307, y=1.0) -> (0:w1309:bool)
            n431 = case shown="False" w1309 {
              tunnel: w1307 -> [w1331 w1334]
              tunnel: [w1330 w1332] -> w1320
              frame False {
                n432 = Reciprocal(x=w1331) -> (1/x=w1328:sgl)
                n433 = Add(x=w1328, y=sgl 0.01 ("x")) -> (x+y=w1326:sgl)
                n434 = Round Toward -Infinity(1:w1326) -> (0:w1329:sgl)
                n435 = Increment(x=w1329) -> (x+1=w1327:sgl)
                n436 = Reciprocal(x=w1327) -> (1/x=w1330:sgl)
              }
              frame True {
                n437 = Round Toward +Infinity(x=w1334) -> (ceil(x): smallest int >= x=w1333:sgl)
                n438 = Decrement(x=w1333) -> (x-1=w1332:sgl)
              }
            }
            n439 = Bundle(w1320, w1320) -> (w1319:cluster{sgl, sgl})  [unwired: 1 in]
            n440 = property class="ImageControl"(reference=w1318, "ZoomSingle"=w1319, "Image Center Position"=w1317) -> ()  [unwired: 1 in, 2 out]
            n441 = Get Menu Item Info(7:w1310, 11:w1316) -> (1:w1313:bool, 2:w1314:string, 3:w1315:refnum<k9>, 6:w1312:T20)  [unwired: 1 in, 3 out]
            n442 = Set Menu Item Info(4:w1312, 6:FALSE ("checked"), 7:w1310, 9:w1313, 10:w1314, 11:w1315) -> ()  [unwired: 1 in, 2 out]
          }
          frame "ZoomToFit" {
            w1340 = "ZoomToFit" ("item tag")
            # "and make sure the image obeys the result"
            # "Toggle menu checkmark"
            n443 = Get Menu Item Info(7:w1340, 11:w1339) -> (1:w1338:bool, 2:w1342:string, 3:w1343:refnum<k9>, 4:w1337:bool, 6:w1341:T20)  [unwired: 1 in, 2 out]
            n444 = Not(x=w1337) -> (.not. x?=w1335:bool)
            n445 = Set Menu Item Info(4:w1341, 6:w1335, 7:w1340, 9:w1338, 10:w1342, 11:w1343) -> ()  [unwired: 1 in, 2 out]
            n446 = property class="ImageControl"(reference=w1336, "Zoom to Fit Mode"=w1335) -> ()  [unwired: 1 in, 2 out]
          }
          frame "ShowGrid" {
            w1351 = "ShowGrid" ("item tag")
            # "Toggle menu checkmark"
            n447 = Get Menu Item Info(7:w1351, 11:w1350) -> (1:w1349:bool, 2:w1353:string, 3:w1354:refnum<k9>, 4:w1348:bool, 6:w1352:T20)  [unwired: 1 in, 2 out]
            n448 = Not(x=w1348) -> (.not. x?=w1347:bool)
            n449 = Set Menu Item Info(4:w1352, 6:w1347, 7:w1351, 9:w1349, 10:w1353, 11:w1354) -> ()  [unwired: 1 in, 2 out]
            n450 = call "grid_and_guides.vi"("Boolean"=w1347, "Operation"=T12."Set grid visibility") -> ()  [unwired: 9 in, 1 out]
          }
          frame "ShowGuides" {
            w1362 = "ShowGuides" ("item tag")
            # "Toggle menu checkmark"
            n451 = Get Menu Item Info(7:w1362, 11:w1361) -> (1:w1360:bool, 2:w1364:string, 3:w1365:refnum<k9>, 4:w1359:bool, 6:w1363:T20)  [unwired: 1 in, 2 out]
            n452 = Not(x=w1359) -> (.not. x?=w1358:bool)
            n453 = Set Menu Item Info(4:w1363, 6:w1358, 7:w1362, 9:w1360, 10:w1364, 11:w1365) -> ()  [unwired: 1 in, 2 out]
            n454 = call "grid_and_guides.vi"("Boolean"=w1358, "Operation"=T12."Set guide visibility") -> ()  [unwired: 9 in, 1 out]
          }
          frame "ConfigureGridAndGuides" {
            n455 = call "grid_and_guides.vi"("Operation"=T12."Show front panel") -> ()  [unwired: 10 in, 1 out]
          }
          frame "ShowSettings" {
            n456 = call "UDP Sender generic_2.vi"("Show panel"=TRUE, "Spots"=w1372) -> ()  [unwired: 1 in, 1 out]
          }
          frame "CameraSettings" {
            n457 = global read "red_tweezers_globals_INTERNAL_VOLATILE.vi" "Current Camera VI"() -> (w1375:path)
            n458 = Open VI Reference(vi path=w1375) -> (vi reference=w1374:refnum<vi>)  [unwired: 5 in, 1 out]
            n459 = property class="VI"(reference=w1374, "Front Panel.Open"=TRUE ("Front Panel Window:Open")) -> ()  [unwired: 1 in, 2 out]
          }
          frame Default {
          }
        }
      }
      event Mouse Down? {
        # "We don't process clicks when the user is on the video tab, so that we can set ROIs."
        # "When the mouse button goes down over the image, we save where it went down, etc. and wait to see what happens next.  We also register to be told when the mouse leaves the control, goes up, or moves.  \"click\" or \"drag\" are only detected once the mouse moves or goes up."
        n460 = event-data() -> ("Coords"=w1395:T21, "Button"=w1390:u16, "Mods"=w1399:cluster{"Double Click":bool, "Menu Key":bool}, "PlatMods"=w1398:T22)  [unwired: 1 in]
        n461 = call "mouse_to_image_coords.vi"("Mouse Coords (screen/pane units)"=w1395, "Image Control"=w1391) -> ("Cursor is on Display Area"=w1389:bool, "Mouse Coords (image pixels)"=w1394:cluster{dbl, dbl})  [unwired: 4 in]
        n462 = disable-structure shown="Enabled" {
          disable-tunnel: w1390 -> [w1407 _]
          disable-tunnel: w1389 -> [w1405 w1408]
          disable-tunnel: [w1404 w1408] -> w1385
          frame Enabled {
            n463 = Equal?(x=u16 1, y=w1407) -> (x = y?=w1406:bool)
            n464 = And(x=w1405, y=w1406) -> (x .and. y?=w1404:bool)
          }
          frame Disabled {
            # "use other pane to allow right-clicking on image"
          }
        }
        n465 = local read "Tab"() -> (w1386:T4)
        n466 = Not Equal?(x=w1386, y=T13."Video" ("Tab")) -> (x != y?=w1384:bool)
        n467 = And(x=w1385, y=w1384) -> (x .and. y?=w1383:bool)
        n468 = case shown="False" w1383 {
          tunnel: w1402 -> [w1411 w1422]
          tunnel: [T10 {"Button Down"=FALSE, "Dragging"=FALSE, "Position (Image Pixels)"={"X"=0.0, "Y"=0.0}, "Previous Position (Image Pixels)"={"X"=0.0, "Y"=0.0}, "Button"=0, "Mods"={"Double Click"=FALSE, "Menu Key"=FALSE}, "PlatMods"={"Shift"=FALSE, "Ctrl"=FALSE, "Alt"=FALSE, "Cmd"=FALSE, "Opt"=FALSE}} w1421] -> w1401
          tunnel: [w1411 w1418] -> w1400
          tunnel: w1390 -> [_ w1417]
          tunnel: w1399 -> [_ w1416]
          tunnel: w1398 -> [_ w1415]
          tunnel: w1394 -> [_ w1414]
          tunnel: [FALSE TRUE] -> w1393
          tunnel: w1391 -> [_ w1412]
          frame False {
            # "If the user clicked on a scrollbar, ignore it and let LabVIEW handle it. (this keeps the scrollbars working)"
          }
          frame True {
            w1420 = FALSE  # Dragging
            w1419 = TRUE  # Button Down
            n469 = register-events(reference=w1422, w1412, w1412, w1412, w1412) -> (reference out=w1418:refnum<event-registration>)  [unwired: 1 in, 1 out]
            n470 = Bundle("Button Down"=w1419, "Dragging"=w1420, "Mouse Coords (image pixels)"=w1414, "Mouse Coords (image pixels)"=w1414, "Button"=w1417, "Mods"=w1416, "PlatMods"=w1415) -> (w1421:T23)  [unwired: 1 in]
          }
        }
        n471 = Array Size(array=w1381) -> (size(s)=w1382:i32)
        n472 = local write "# of Spots"(w1382) -> ()
        n473 = local write "Selection/Group"(w1381) -> ()
        n474 = event-data("Discard?"=w1393) -> ()  [unwired: 4 in, 1 out]
      }
      event Mouse Leave {
        w1429 = refnum<vi> refnum  # Dummy
        # "When the mouse leaves, we reset things."
        n475 = event-data() -> ()  [unwired: 1 in, 2 out]
        n476 = register-events(reference=w1430, w1428, w1429, w1429, w1429) -> (reference out=w1427:refnum<event-registration>)  [unwired: 1 in, 1 out]
      }
      event Mouse Up {
        w1449 = refnum<vi> refnum  # Dummy
        # "Double clicking adds a spot at the mouse position."
        # "deregister"
        # "If we get here the mouse has gone down and up again.  If we've not moved in between, we have a Click.\nEither way we're no longer interested in mouse leave/move/up events."
        n477 = event-data() -> ("Mods"=w1436:cluster{"Double Click":bool, "Menu Key":bool})  [unwired: 1 in, 5 out]
        n478 = Unbundle By Name(w1442) -> ("Dragging"=w1451:bool)
        n479 = Unbundle By Name(w1436) -> ("Double Click"=w1433:bool)
        n480 = Not(x=w1451) -> (.not. x?=w1450:bool)
        n481 = Not(x=w1438) -> (.not. x?=w1440:bool)
        n482 = And(x=w1450, y=w1440) -> (x .and. y?=w1434:bool)
        n483 = case shown="True" w1434 {
          tunnel: w1442 -> [_ w1457]
          tunnel: w1444 -> [w1452 w1456]
          tunnel: w1443 -> [w1453 w1459]
          tunnel: [w1453 w1458] -> w1445
          tunnel: w1433 -> [_ w1454]
          tunnel: [w1452 w1455] -> w1435
          frame False {
          }
          frame True {
            n484 = case shown="False" w1454 {
              tunnel: w1459 -> [w1466 w1516]
              tunnel: [w1464 w1522] -> w1458
              tunnel: w1456 -> [w1460 w1523]
              tunnel: w1457 -> [w1463 w1518]
              tunnel: [w1460 w1514] -> w1455
              frame False {
                w1470 = 400.0  # 20^2 px
                # "If the user clicked, determine which spots should be selected: if we've clicked a spot/group then select it.  Shift-clicking toggles selection for that spot, and leaves the rest of the selection unchanged."
                # "check we're close enough"
                # "find closest"
                n485 = Unbundle By Name(w1463) -> ("Position (Image Pixels)"=w1462:cluster{"X":dbl, "Y":dbl}, "PlatMods.Shift"=w1461:bool)
                n486 = for {
                  tunnel: [w1506] -> w1468 mode=indexing
                  tunnel: w1462 -> [w1505]
                  tunnel: w1460 -> [w1504] mode=indexing
                  # "calculate distances between mouse position and spot positions"
                  n487 = call "extract_position.vi"("Spot"=w1504) -> ("Position"=w1503:cluster{"x":dbl, "y":dbl, "z":dbl})
                  n488 = call "coords_real_to_image_currentview.vi"("Position (real coords)"=w1503) -> ("Position (pixels, relative to the top left of the image)"=w1502:cluster{dbl, dbl})  [unwired: 7 in, 1 out]
                  n489 = Subtract(x=w1502, y=w1505) -> (x-y=w1509:cluster{dbl, dbl})
                  n490 = Multiply(x=w1509, y=w1509) -> (x*y=w1508:cluster{dbl, dbl})
                  n491 = Cluster To Array(cluster=w1508) -> (array=w1507:dbl[])
                  n492 = Add Array Elements(numeric array=w1507) -> (sum=w1506:dbl)
                }
                n493 = Array Max & Min(array=w1468) -> (min value=w1469:dbl, min index (indices)=w1465:i32)  [unwired: 2 out]
                n494 = Less Or Equal?(x=w1469, y=w1470) -> (x <= y?=w1467:bool)
                n495 = case shown="True" w1467 {
                  tunnel: w1466 -> [w1471 w1478]
                  tunnel: w1465 -> [_ w1472]
                  tunnel: w1461 -> [_ w1474]
                  tunnel: [w1471 w1473] -> w1464
                  frame False {
                    # "If we didn't click a spot, do nothing."
                  }
                  frame True {
                    # "If the spot is in a group, act on all spots in that group, not just the spot we clicked."
                    # "This case statement toggles the selection of the spot/group we clicked, and leaves other spots unchanged if we're holding shift.  Otherwise, we select the spot/group that was clicked and deselect everything else."
                    n496 = stacked-sequence {
                      tunnel: w1472 -> [_ w1480]
                      frame #0 {
                        n497 = local read "Current Spot #"() -> (→"Prev Current Spot":dbl)
                      }
                      frame #1 {
                        "Current Spot #" <- w1480
                      }
                    }
                    n498 = Index Array(array=w1478, index=w1472) -> (element=w1477:T7)
                    n499 = Unbundle(w1477) -> ("Group ID"=w1475:i32)  [unwired: 1 out]
                    n500 = Greater Than 0?(x=w1475) -> (x > 0?=w1476:bool)
                    n501 = for {
                      tunnel: w1478 -> [w1491] mode=indexing
                      tunnel: w1476 -> [w1488]
                      tunnel: w1475 -> [w1487]
                      tunnel: w1472 -> [w1486]
                      tunnel: w1474 -> [w1484]
                      tunnel: [w1482] -> w1473 mode=indexing
                      i -> [w1485]
                      n502 = Unbundle(w1491) -> ("Group ID"=w1481:i32, "Selected"=w1489:bool)
                      n503 = case shown="True" w1488 {
                        tunnel: w1481 -> [_ w1495]
                        tunnel: [w1493 w1497] -> w1483
                        tunnel: w1487 -> [_ w1496]
                        tunnel: w1486 -> [w1494 _]
                        tunnel: w1485 -> [w1492 _]
                        frame False {
                          n504 = Equal?(x=w1492, y=w1494) -> (x = y?=w1493:bool)
                        }
                        frame True {
                          n505 = Equal?(x=w1495, y=w1496) -> (x = y?=w1497:bool)
                        }
                      }
                      n506 = case shown="True" w1484 {
                        tunnel: [w1498 w1499] -> w1490
                        tunnel: w1489 -> [_ w1500]
                        tunnel: w1483 -> [w1498 w1501]
                        frame False {
                        }
                        frame True {
                          n507 = Exclusive Or(1:w1501, 2:w1500) -> (0:w1499:bool)
                        }
                      }
                      n508 = Bundle("Group ID"=w1481, w1490) -> (w1482:cluster{"Group ID":i32, bool})  [unwired: 1 out]
                    }
                  }
                }
              }
              frame True {
                # "convert mouse position to real coords, and add a spot there."
                # "Double-click detected"
                n509 = Unbundle By Name(w1518) -> ("Position (Image Pixels)"=w1517:cluster{"X":dbl, "Y":dbl})
                n510 = for {
                  tunnel: w1516 -> [w1526] mode=indexing
                  tunnel: [w1525] -> w1515 mode=indexing
                  n511 = Bundle(cluster=w1526, "Selected"=FALSE) -> (w1525:T7)  [unwired: 1 in]
                }
                n512 = call "coords_image_to_real_currentimage.vi"("Position (pixels on image)"=w1517) -> ("Position (real coords)"=w1519:cluster{dbl, dbl, "Z":dbl})  [unwired: 9 in]
                n513 = call "replace_position.vi"("Position"=w1519) -> ("Spot"=w1521:T1)  [unwired: 3 in]
                n514 = Build Array (concatenate)(w1523, w1521) -> (w1514:T1[])
                n515 = Build Array (concatenate)(w1515, T7 {"Group ID"=0, "Selected"=TRUE} ("selection_element")) -> (w1522:T7[])
                n516 = Array Size(array=w1514) -> (size(s)=w1513:i32)
                n517 = local write "Induce check"(TRUE) -> ()
                n518 = Subtract(x=w1513, y=1) -> (x-y=w1512:i32)
                n519 = local write "Current Spot #"(w1512) -> ()
              }
            }
          }
        }
        n520 = register-events(reference=w1447, w1446, w1449, w1449, w1449) -> (reference out=w1448:refnum<event-registration>)  [unwired: 1 in, 1 out]
      }
      event Mouse Move {
        n521 = event-data() -> ("Coords"=w1541:T21)  [unwired: 1 in, 2 out]
        n522 = call "mouse_to_image_coords.vi"("Mouse Coords (screen/pane units)"=w1541, "Image Control"=w1540) -> ("Mouse Coords (image pixels)"=w1532:cluster{dbl, dbl})  [unwired: 4 in, 1 out]
        n523 = Not(x=w1531) -> (.not. x?=w1536:bool)
        n524 = case shown="True" w1536 {
          tunnel: w1534 -> [_ w1554]
          tunnel: w1539 -> [w1546 w1556]
          tunnel: w1538 -> [w1545 w1555]
          tunnel: [w1545 w1555] -> w1527
          tunnel: [w1546 w1557] -> w1537
          tunnel: w1532 -> [_ w1548]
          tunnel: w1528 -> [_ w1547]
          frame False {
          }
          frame True {
            # "this is the displacement of the mouse, since the last iteration, in \"real\" coordinates (NB the conversions go before subtracting, as it may involve adding a constant as well as multiplying, which would confuse things as we're only interested in displacements here."
            # "The \"position\" local variable is there just in case we're on the \"current spot\" tab, so that the position updates nicely"
            # "If the user is dragging, translate the spots.\nHolding down shift causes the mouse's motion to be transformed into scaling about the centroid of the spots and rotation about the same point"
            n525 = Unbundle By Name(w1554) -> ("Position (Image Pixels)"=w1549:cluster{"X":dbl, "Y":dbl})
            n526 = call "find_centroid.vi"("Selection and Groups"=w1555, "Spots"=w1556) -> ("centroid"=w1550:cluster{"x":dbl, "y":dbl, "z":dbl})  [unwired: 2 in, 4 out]
            n527 = Unbundle By Name(w1554) -> ("PlatMods.Shift"=w1553:bool)
            n528 = disable-structure shown="Disabled" {
              disable-tunnel: w1550 -> [w1558 _]
              frame Disabled {
                n529 = local write "Position"(w1558) -> ()
              }
              frame Enabled {
              }
            }
            n530 = call "coords_image_to_real_currentimage.vi"("Position (pixels on image)"=w1548) -> ("Position (real coords)"=w1551:cluster{dbl, dbl, "Z":dbl})  [unwired: 9 in]
            n531 = call "coords_image_to_real_currentimage.vi"("Position (pixels on image)"=w1549) -> ("Position (real coords)"=w1552:cluster{dbl, dbl, "Z":dbl})  [unwired: 9 in]
            n532 = case shown="False" w1553 {
              tunnel: [w1563 w1837] -> w1557
              tunnel: w1556 -> [w1569 w1838]
              tunnel: w1555 -> [w1568 w1836]
              tunnel: w1552 -> [w1567 w1823]
              tunnel: w1550 -> [_ w1833]
              tunnel: w1551 -> [w1564 w1824]
              tunnel: w1547 -> [_ _]
              frame False {
                # "Spot Checker passes on information for the bubble collision,system so proper calculations can be made."
                n533 = while {
                  tunnel: w1567 -> [w1608]
                  tunnel: [w1598] -> w1565
                  tunnel: w1564 -> [w1597]
                  i -> [w1591]
                  stop <- w1593 stop-if-true
                  w1583 = 0
                  # "This while loop statement makes sure\nthat every spot gets checked before \nallowing any spot to move."
                  # "Buffer zone controls the amount of space between the\ncenter of a spot compared to the center of another spot.\nThis is used to prevent bubbles from colliding with each other."
                  # "Projected distance calculates the distance between two spots- this is used for when a \"hit\" occurs. If the projected distance becomes larger than the previous distance, the program will assume that the spot is being pulled from the buffer zone and as a result will allow the bubble to exit."
                  # "This subVI leads to the distance function, which outputs the distance between a spot being checked compared to the current spot number."
                  n534 = control-ref of="Value Check"() -> (w1588:refnum<vi>)
                  n535 = control-ref of="ID num check"() -> (w1587:refnum<vi>)
                  n536 = control-ref of="Spot Checker"() -> (w1604:refnum<vi>)
                  n537 = Subtract(x=w1597, y=w1608) -> (x-y=w1598:cluster{dbl, dbl, "Z":dbl})
                  n538 = call "DistanceFunction.vi"("Condition Driver"=FALSE, "Position (real coords)"=w1608, "Current Spot Number"=w1587, "Spot Checker"=w1604, "Spot Number Being Checked"=w1588) -> ("Distance"=w1572:dbl)  [unwired: 6 in]
                  n539 = stacked-sequence {
                    tunnel: w1572 -> [_ w1613]
                    frame #0 {
                      n540 = local read "Distance"() -> (→"Previous Distance":dbl)
                    }
                    frame #1 {
                      "Distance" <- w1613
                    }
                  }
                  n541 = Unbundle(w1598) -> (→"X Displacement":dbl, →"Y Displacement":dbl)  [unwired: 1 out]
                  n542 = control-ref of="ID num check"() -> (w1589:refnum<vi>)
                  n543 = control-ref of="Spot Checker"() -> (w1602:refnum<vi>)
                  n544 = control-ref of="Y Displacement"() -> (w1600:refnum<vi>)
                  n545 = control-ref of="Value Check"() -> (w1590:refnum<vi>)
                  n546 = control-ref of="X Displacement"() -> (w1601:refnum<vi>)
                  n547 = call "ProjectedDistance.vi"("X Displacement"=w1601, "Spot Number Check"=w1590, "Current Spot #"=w1589, "Spot Checker"=w1602, "Y Displacement"=w1600) -> ("Numeric"=→"Projected Distance":dbl)  [unwired: 6 in]
                  n548 = Multiply(x="Buffer Zone", y=2) -> (x*y=w1607:dbl)
                  n549 = local read "ID num check"() -> (w1584:dbl)
                  n550 = local read "Value Check"() -> (w1585:dbl)
                  n551 = local read "Projected Distance"() -> (w1576:dbl)
                  n552 = Equal?(x=w1572, y=0) -> (x = y?=w1573:bool)
                  n553 = case shown="True" w1573 {
                    frame False {
                      n554 = local read "Hit"() -> (w1610:bool)
                      n555 = local write "Hit Indicator"(w1610) -> ()
                    }
                    frame True {
                      "Hit Indicator" <- FALSE
                    }
                  }
                  n556 = Not Equal?(x=w1576, y=0) -> (x != y?=w1574:bool)
                  n557 = Less Or Equal?(x=w1572, y=w1607) -> (x <= y?=w1577:bool)
                  n558 = Equal?(x=w1584, y=w1583) -> (x = y?=w1582:bool)
                  n559 = And(x=w1577, y=w1574) -> (x .and. y?=w1570:bool)
                  "Hit" <- w1570
                  n560 = Equal?(x=w1583, y=w1585) -> (x = y?=w1581:bool)
                  n561 = Not(x=w1570) -> ()  [unwired: 1 out]
                  n562 = And(x=w1582, y=w1581) -> (x .and. y?=w1580:bool)
                  n563 = Or(x=w1570, y=w1580) -> (x .or. y?=w1586:bool)
                  n564 = case shown="True" w1586 {
                    frame False {
                      n565 = stacked-sequence {
                        frame #0 {
                          n566 = local read "Potential Collisions"() -> (w1616:dbl)
                          n567 = local read "Spot # Check"() -> (w1618:dbl)
                          n568 = Subtract(x=w1616, y=1) -> (x-y=w1614:dbl)
                          n569 = Less Or Equal?(x=w1618, y=w1614) -> (x <= y?=w1617:bool)
                          n570 = case shown="True" w1617 {
                            frame False {
                              # "Spot # Check resets if the the number of potential collisons is more than Spot # Check."
                              n571 = local write "Spot # Check"(0) -> ()
                            }
                            frame True {
                              n572 = stacked-sequence {
                                frame #0 {
                                # "Spot # Check increments by 1 every time it is greater than the # of potential collisions."
                                n573 = local read "Spot # Check"() -> (w1622:dbl)
                                n574 = Add(x=w1622, y=1) -> (x+y=→"Spot # Check":dbl)
                                }
                                frame #1 {
                                # "Spot # Check resets if the Spot # Check is eqaul to the # of potential collisions."
                                n575 = local read "Potential Collisions"() -> (w1623:dbl)
                                n576 = local read "Spot # Check"() -> (w1624:dbl)
                                n577 = Equal?(x=w1624, y=w1623) -> (x = y?=w1625:bool)
                                n578 = case shown="True" w1625 {
                                frame False {
                                }
                                frame True {
                                n579 = local write "Spot # Check"(0) -> ()
                                }
                                }
                                }
                                frame #2 {
                                n580 = local read "Spot Checker"() -> (w1640:T1[])
                                n581 = local read "Current Spot #"() -> (w1641:dbl)
                                n582 = local read "Area to check"() -> (w1627:dbl)
                                n583 = Index Array(array=w1640, index=w1641) -> (element=w1639:T1)
                                n584 = local read "Orig Y SC"() -> (w1636:dbl)
                                n585 = Unbundle By Name(w1639) -> ("Position.x"=w1637:dbl, "Position.y"=w1635:dbl)
                                n586 = local read "Orig X SC"() -> (w1638:dbl)
                                n587 = Subtract(x=w1635, y=w1636) -> (x-y=w1628:dbl)
                                n588 = Absolute Value(x=w1628) -> (abs(x)=w1629:dbl)
                                n589 = Subtract(x=w1637, y=w1638) -> (x-y=w1631:dbl)
                                n590 = Greater?(x=w1629, y=w1627) -> (0:w1633:bool)
                                n591 = Absolute Value(x=w1631) -> (abs(x)=w1630:dbl)
                                n592 = Greater?(x=w1630, y=w1627) -> (0:w1632:bool)
                                n593 = Or(x=w1632, y=w1633) -> (x .or. y?=w1634:bool)
                                n594 = case shown="True" w1634 {
                                frame False {
                                }
                                frame True {
                                n595 = stacked-sequence {
                                frame #0 {
                                n596 = local read "Null array"() -> (w1646:dbl[])
                                n597 = local write "What to Check"(w1646) -> ()
                                n598 = local write "ID"(w1646) -> ()
                                n599 = local read "Current Spot #"() -> (w1648:dbl)
                                n600 = local write "Potential Collisions"(0) -> ()
                                n601 = local read "Spot Checker"() -> (w1647:T1[])
                                n602 = Index Array(array=w1647, index=w1648) -> (element=w1649:T1)
                                n603 = Wait (ms)(milliseconds to wait=100) -> ()  [unwired: 1 out]
                                n604 = Unbundle By Name(w1649) -> ("Position.x"=w1643:dbl, "Position.y"=w1644:dbl)
                                n605 = local write "Orig Y SC"(w1644) -> ()
                                n606 = local write "Orig X SC"(w1643) -> ()
                                }
                                frame #1 {
                                # "All this is a  statement checking whether the microrobot is within the area being checked using absolute value statements. The number of potential collisions gets added by 1 every time a bubble is detected within the area."
                                n607 = local read "# of Spots"() -> (w1650:dbl)
                                n608 = for {
                                N: w1650 -> [_]
                                tunnel: w1650 -> [w1655]
                                i -> [w1651]
                                n609 = local read "Selection/Group"() -> (w1654:T7[])
                                n610 = Index Array(array=w1654, index=w1651) -> (element=w1653:T7)
                                n611 = Unbundle By Name(w1653) -> ("Selected"=w1652:bool)
                                n612 = case shown="True" w1652 {
                                tunnel: w1655 -> [_ w1657]
                                tunnel: w1651 -> [_ w1656]
                                frame False {
                                }
                                frame True {
                                n613 = for {
                                N: w1657 -> [_]
                                tunnel: w1656 -> [w1658]
                                i -> [w1659]
                                n614 = local read "Selection/Group"() -> (w1663:T7[])
                                n615 = Index Array(array=w1663, index=w1659) -> (element=w1662:T7)
                                n616 = Unbundle By Name(w1662) -> ("Selected"=w1660:bool)
                                n617 = Not(x=w1660) -> (.not. x?=w1661:bool)
                                n618 = case shown="True" w1661 {
                                tunnel: w1659 -> [_ w1667]
                                tunnel: w1658 -> [_ w1666]
                                tunnel: w1658 -> [_ w1665]
                                frame False {
                                }
                                frame True {
                                n619 = local read "Spot Checker"() -> (w1684:T1[])
                                n620 = Index Array(array=w1684, index=w1667) -> (element=w1685:T1)
                                n621 = Index Array(array=w1684, index=w1666) -> (element=w1683:T1)
                                n622 = Unbundle By Name(w1683) -> ("Position.x"=w1680:dbl, "Position.y"=w1676:dbl)
                                n623 = Unbundle By Name(w1685) -> ("Position.x"=w1677:dbl, "Position.y"=w1673:dbl)
                                n624 = local read "Area+ Buffer"() -> (w1664:dbl)
                                n625 = Subtract(x=w1680, y=w1664) -> (x-y=w1681:dbl)
                                n626 = Greater Or Equal?(x=w1677, y=w1681) -> (x >= y?=w1682:bool)
                                n627 = Add(x=w1676, y=w1664) -> (x+y=w1675:dbl)
                                n628 = Subtract(x=w1676, y=w1664) -> (x-y=w1674:dbl)
                                n629 = Add(x=w1680, y=w1664) -> (x+y=w1678:dbl)
                                n630 = Less Or Equal?(x=w1673, y=w1675) -> (x <= y?=w1672:bool)
                                n631 = Greater Or Equal?(x=w1673, y=w1674) -> (x >= y?=w1671:bool)
                                n632 = Less Or Equal?(x=w1677, y=w1678) -> (x <= y?=w1679:bool)
                                n633 = And(x=w1682, y=w1679) -> (x .and. y?=w1669:bool)
                                n634 = And(x=w1672, y=w1671) -> (x .and. y?=w1670:bool)
                                n635 = And(x=w1669, y=w1670) -> (x .and. y?=w1668:bool)
                                n636 = case shown="True" w1668 {
                                tunnel: w1667 -> [_ _]
                                tunnel: w1667 -> [_ w1687]
                                tunnel: w1665 -> [_ w1686]
                                frame False {
                                }
                                frame True {
                                n637 = stacked-sequence {
                                tunnel: w1687 -> [w1688 _]
                                tunnel: w1686 -> [w1689 _]
                                frame #0 {
                                n638 = local read "Potential Collisions"() -> (w1692:dbl)
                                n639 = local read "What to Check"() -> (w1693:dbl[])
                                n640 = Insert Into Array(array=w1693, index=w1692, new element=w1688) -> (w1694:dbl[])
                                n641 = local read "ID"() -> (w1691:dbl[])
                                n642 = local write "What to Check"(w1694) -> ()
                                n643 = Insert Into Array(array=w1691, index=w1692, new element=w1689) -> (w1690:dbl[])
                                n644 = local write "ID"(w1690) -> ()
                                }
                                frame #1 {
                                n645 = local read "Potential Collisions"() -> (w1697:dbl)
                                n646 = Add(x=w1697, y=1) -> (x+y=w1695:dbl)
                                n647 = local write "Potential Collisions"(w1695) -> ()
                                }
                                }
                                }
                                }
                                }
                                }
                                }
                                }
                                }
                                }
                                }
                                frame #2 {
                                n648 = local read "Current Spot #"() -> (w1698:dbl)
                                n649 = local write "Prev Current Spot"(w1698) -> ()
                                }
                                }
                                }
                                }
                                }
                              }
                            }
                          }
                        }
                        frame #1 {
                          # "This updates the ID and Value being checked at the beginning of IDs and values being checked."
                          n650 = local read "Spot # Check"() -> (w1701:dbl)
                          n651 = local read "What to Check"() -> (w1702:dbl[])
                          n652 = local read "ID"() -> (w1703:dbl[])
                          n653 = Index Array(array=w1703, index=w1701) -> (element=w1700:dbl)
                          n654 = Index Array(array=w1702, index=w1701) -> (element=w1699:dbl)
                          n655 = local write "Value Check"(w1699) -> ()
                          n656 = local write "ID num check"(w1700) -> ()
                        }
                      }
                    }
                    frame True {
                      n657 = stacked-sequence {
                        frame #0 {
                          # "This section activate a case statement which allows us to change the area being checked. Orig X/Y SC holds the position of the area to check and changes after the bubble exits the area beig checked."
                          # "This statement controls the areas selected and finds which bubbles needs to be checked. This activates when the bubble\nmoves out of the area specified."
                          n658 = local read "# of Spots"() -> (w1723:dbl)
                          n659 = local read "Current Spot #"() -> (w1722:dbl)
                          n660 = Subtract(x=w1723, y=1) -> (x-y=w1724:dbl)
                          n661 = Equal?(x=w1722, y=w1724) -> (x = y?=w1720:bool)
                          n662 = case shown="True" w1720 {
                            tunnel: [w1783 w1786] -> w1721
                            frame True {
                              n663 = local read "# of Spots"() -> (w1784:dbl)
                              n664 = Subtract(x=w1784, y=2) -> (x-y=w1783:dbl)
                            }
                            frame False {
                              n665 = local read "# of Spots"() -> (w1785:dbl)
                              n666 = Subtract(x=w1785, y=1) -> (x-y=w1786:dbl)
                            }
                          }
                          "Maximum" <- w1721
                          n667 = local read "Spot Checker"() -> (w1719:T1[])
                          n668 = local read "Current Spot #"() -> (w1718:dbl)
                          n669 = Index Array(array=w1719, index=w1718) -> (element=w1717:T1)
                          n670 = Unbundle By Name(w1717) -> ("Position.x"=w1716:dbl, "Position.y"=w1715:dbl)
                          n671 = local read "Orig Y SC"() -> (w1713:dbl)
                          n672 = local read "Orig X SC"() -> (w1714:dbl)
                          n673 = Subtract(x=w1715, y=w1713) -> (x-y=w1710:dbl)
                          n674 = Subtract(x=w1716, y=w1714) -> (x-y=w1712:dbl)
                          n675 = Absolute Value(x=w1710) -> (abs(x)=w1709:dbl)
                          n676 = Absolute Value(x=w1712) -> (abs(x)=w1711:dbl)
                          n677 = local read "Area to check"() -> (w1705:dbl)
                          n678 = local read "Area to check"() -> (w1704:dbl)
                          n679 = Greater?(x=w1711, y=w1705) -> (0:w1708:bool)
                          n680 = Greater?(x=w1709, y=w1704) -> (0:w1707:bool)
                          n681 = Or(x=w1708, y=w1707) -> (x .or. y?=w1706:bool)
                          n682 = case shown="True" w1706 {
                            frame False {
                            }
                            frame True {
                              n683 = stacked-sequence {
                                frame #0 {
                                # "A small time delay of 100 ms is provided to allow the data to pass throguh properly."
                                n684 = Wait (ms)(milliseconds to wait=100) -> ()  [unwired: 1 out]
                                n685 = local read "Null array"() -> (→"What to Check" →"ID":dbl[])
                                n686 = local read "Spot Checker"() -> (w1731:T1[])
                                n687 = local read "Current Spot #"() -> (w1730:dbl)
                                n688 = Index Array(array=w1731, index=w1730) -> (element=w1729:T1)
                                n689 = Unbundle By Name(w1729) -> ("Position.x"=→"Orig X SC":dbl, "Position.y"=→"Orig Y SC":dbl)
                                "Potential Collisions" <- 0
                                }
                                frame #1 {
                                n690 = local read "# of Spots"() -> (w1734:dbl)
                                n691 = for {
                                N: w1734 -> [_]
                                tunnel: w1734 -> [w1739]
                                i -> [w1735]
                                n692 = local read "Selection/Group"() -> (w1738:T7[])
                                n693 = Index Array(array=w1738, index=w1735) -> (element=w1737:T7)
                                n694 = Unbundle By Name(w1737) -> ("Selected"=w1736:bool)
                                n695 = case shown="True" w1736 {
                                tunnel: w1739 -> [_ w1741]
                                tunnel: w1735 -> [_ w1740]
                                frame False {
                                }
                                frame True {
                                n696 = for {
                                N: w1741 -> [_]
                                tunnel: w1740 -> [w1742]
                                i -> [w1743]
                                n697 = local read "Selection/Group"() -> (w1747:T7[])
                                n698 = Index Array(array=w1747, index=w1743) -> (element=w1746:T7)
                                n699 = Unbundle By Name(w1746) -> ("Selected"=w1744:bool)
                                n700 = Not(x=w1744) -> (.not. x?=w1745:bool)
                                n701 = case shown="True" w1745 {
                                tunnel: w1743 -> [_ w1751]
                                tunnel: w1742 -> [_ w1750]
                                tunnel: w1742 -> [_ w1749]
                                frame False {
                                }
                                frame True {
                                n702 = local read "Spot Checker"() -> (w1768:T1[])
                                n703 = Index Array(array=w1768, index=w1751) -> (element=w1769:T1)
                                n704 = Index Array(array=w1768, index=w1750) -> (element=w1767:T1)
                                n705 = Unbundle By Name(w1767) -> ("Position.x"=w1764:dbl, "Position.y"=w1760:dbl)
                                n706 = Unbundle By Name(w1769) -> ("Position.x"=w1761:dbl, "Position.y"=w1757:dbl)
                                n707 = local read "Area+ Buffer"() -> (w1748:dbl)
                                n708 = Subtract(x=w1764, y=w1748) -> (x-y=w1765:dbl)
                                n709 = Greater Or Equal?(x=w1761, y=w1765) -> (x >= y?=w1766:bool)
                                n710 = Add(x=w1760, y=w1748) -> (x+y=w1759:dbl)
                                n711 = Subtract(x=w1760, y=w1748) -> (x-y=w1758:dbl)
                                n712 = Add(x=w1764, y=w1748) -> (x+y=w1762:dbl)
                                n713 = Less Or Equal?(x=w1757, y=w1759) -> (x <= y?=w1756:bool)
                                n714 = Greater Or Equal?(x=w1757, y=w1758) -> (x >= y?=w1755:bool)
                                n715 = Less Or Equal?(x=w1761, y=w1762) -> (x <= y?=w1763:bool)
                                n716 = And(x=w1766, y=w1763) -> (x .and. y?=w1753:bool)
                                n717 = And(x=w1756, y=w1755) -> (x .and. y?=w1754:bool)
                                n718 = And(x=w1753, y=w1754) -> (x .and. y?=w1752:bool)
                                n719 = case shown="True" w1752 {
                                tunnel: w1751 -> [_ _]
                                tunnel: w1751 -> [_ w1771]
                                tunnel: w1749 -> [_ w1770]
                                frame False {
                                }
                                frame True {
                                n720 = stacked-sequence {
                                tunnel: w1771 -> [w1772 _]
                                tunnel: w1770 -> [w1773 _]
                                frame #0 {
                                n721 = local read "Potential Collisions"() -> (w1776:dbl)
                                n722 = local read "What to Check"() -> (w1777:dbl[])
                                n723 = Insert Into Array(array=w1777, index=w1776, new element=w1772) -> (w1778:dbl[])
                                n724 = local read "ID"() -> (w1775:dbl[])
                                n725 = Insert Into Array(array=w1775, index=w1776, new element=w1773) -> (w1774:dbl[])
                                n726 = local write "What to Check"(w1778) -> ()
                                n727 = local write "ID"(w1774) -> ()
                                }
                                frame #1 {
                                n728 = local read "Potential Collisions"() -> (w1781:dbl)
                                n729 = Add(x=w1781, y=1) -> (x+y=w1779:dbl)
                                n730 = local write "Potential Collisions"(w1779) -> ()
                                }
                                }
                                }
                                }
                                }
                                }
                                }
                                }
                                }
                                }
                                }
                              }
                            }
                          }
                        }
                        frame #1 {
                          n731 = local read "# of Spots"() -> (w1790:dbl)
                          n732 = Not Equal?(x=w1790, y=1) -> (x != y?=w1788:bool)
                          n733 = case shown="True" w1788 {
                            frame False {
                            }
                            frame True {
                              n734 = stacked-sequence {
                                frame #0 {
                                n735 = local read "Potential Collisions"() -> (w1793:dbl)
                                n736 = local read "Spot # Check"() -> (w1795:dbl)
                                n737 = Subtract(x=w1793, y=1) -> (x-y=w1791:dbl)
                                n738 = Less Or Equal?(x=w1795, y=w1791) -> (x <= y?=w1794:bool)
                                n739 = case shown="False" w1794 {
                                frame False {
                                n740 = local write "Spot # Check"(0) -> ()
                                }
                                frame True {
                                }
                                }
                                }
                                frame #1 {
                                n741 = local read "What to Check"() -> (w1801:dbl[])
                                n742 = local read "ID"() -> (w1799:dbl[])
                                n743 = local read "Spot # Check"() -> (w1797:dbl)
                                n744 = Index Array(array=w1801, index=w1797) -> (element=→"Value Check":dbl)
                                n745 = Index Array(array=w1799, index=w1797) -> (element=→"ID num check":dbl)
                                }
                              }
                            }
                          }
                        }
                      }
                    }
                  }
                  n746 = local read "Potential Collisions"() -> (w1578:dbl)
                  n747 = Subtract(x=w1578, y=1) -> (x-y=w1579:dbl)
                  n748 = local read "Hit"() -> (w1596:bool)
                  n749 = Equal?(x=w1591, y=w1579) -> (x = y?=w1595:bool)
                  n750 = Or(x=w1596, y=w1595) -> (x .or. y?=w1593:bool)
                }
                n751 = for {
                  tunnel: w1568 -> [w1815] mode=indexing
                  tunnel: w1569 -> [w1812] mode=indexing
                  tunnel: [w1814] -> w1563 mode=indexing
                  tunnel: w1565 -> [w1813]
                  # "If the projected distance is greater than the\nprevious distance, then the selected spots will move. \nThis situation only occurs if the bubble is about to/crossing \nthe buffer zone of another bubble. \n\nThe selected spots will also move if none of the bubbles\nare near/crossing the buffer zone of another bubble."
                  n752 = local read "Hit"() -> (w1805:bool)
                  n753 = Unbundle By Name(w1812) -> ()  [unwired: 1 out]
                  n754 = local read "Projected Distance"() -> (w1804:dbl)
                  n755 = Unbundle(w1815) -> ("Group ID"=→"Group ID #":i32, "Selected"=w1809:bool)
                  n756 = local read "Previous Distance"() -> (w1807:dbl)
                  n757 = Not(x=w1805) -> (.not. x?=w1803:bool)
                  n758 = Greater?(x=w1804, y=w1807) -> (0:w1806:bool)
                  n759 = And(x=w1805, y=w1806) -> (x .and. y?=w1802:bool)
                  n760 = Or(x=w1803, y=w1802) -> (x .or. y?=w1808:bool)
                  n761 = And(x=w1809, y=w1808) -> (x .and. y?=w1810:bool)
                  n762 = case shown="True" w1810 {
                    tunnel: w1812 -> [w1816 w1820]
                    tunnel: [w1816 w1819] -> w1814
                    tunnel: w1813 -> [_ w1821]
                    frame False {
                      # "otherwise, leave it alone!"
                    }
                    frame True {
                      # "If the spot is selected, move it by the same amount as the mouse"
                      n763 = call "extract_position.vi"("Spot"=w1820) -> ("Position"=w1818:cluster{"x":dbl, "y":dbl, "z":dbl})
                      n764 = Add(x=w1818, y=w1821) -> (x+y=w1817:cluster{dbl, dbl, dbl})
                      n765 = call "replace_position.vi"("Position"=w1817, "Spot in"=w1820) -> ("Spot"=w1819:T1)  [unwired: 2 out]
                    }
                  }
                }
                "Spot Checker" <- w1563
                n766 = local read "Locked Current Spot"() -> (w1559:dbl)
                n767 = Index Array(array=w1563, index=w1559) -> (element=w1562:T1)
                n768 = Unbundle By Name(w1562) -> ("Position.x"=→"New X":dbl, "Position.y"=→"New Y":dbl)  [unwired: 1 out]
                n769 = Array Size(array=w1563) -> (size(s)=→"# of Spots":i32)
              }
              frame True {
                # "coordinate conversion to find the rotation and scaling done by the mouse, about the centroid of the spots"
                n770 = Subtract(x=w1823, y=w1833) -> (x-y=w1842:cluster{dbl, dbl, dbl})
                n771 = Subtract(x=w1824, y=w1833) -> (x-y=w1841:cluster{dbl, dbl, dbl})
                n772 = Unbundle(w1841) -> (w1827:dbl, w1828:dbl)  [unwired: 1 out]
                n773 = Unbundle(w1842) -> (w1832:dbl, w1831:dbl)  [unwired: 1 out]
                n774 = Re/Im To Polar(2:w1828, 3:w1827) -> (0:w1825:dbl, 1:w1826:dbl)
                n775 = Re/Im To Polar(2:w1831, 3:w1832) -> (0:w1829:dbl, 1:w1830:dbl)
                n776 = Divide(x=w1826, y=w1830) -> (x/y=w1822:dbl)
                n777 = Subtract(x=w1825, y=w1829) -> (x-y=w1834:dbl)
                n778 = Bundle(w1822, w1822, w1822) -> (w1844:cluster{dbl, dbl, dbl})  [unwired: 1 out]
                n779 = call "scale_matrix.vi"("Scale Factors"=w1844) -> ("Scale Matrix"=w1840:T17)
                n780 = call "arb_rotation_matrix.vi"("Unit Vector"=cluster{dbl, dbl, dbl} {0.0, 0.0, 1.0}, "theta"=w1834) -> ("Real Matrix"=w1839:T17)
                n781 = call-poly <vilib>:"A x B.vi"("B"=w1839, "A"=w1840) -> ("A x B"=w1835:T17)  [unwired: 1 out]
                n782 = for {
                  tunnel: w1838 -> [w1850] mode=indexing
                  tunnel: [w1849] -> w1837 mode=indexing
                  tunnel: w1836 -> [w1848] mode=indexing
                  tunnel: w1833 -> [w1846]
                  tunnel: w1835 -> [w1845]
                  n783 = Unbundle(w1848) -> ("Selected"=w1847:bool)  [unwired: 1 out]
                  n784 = case shown="True" w1847 {
                    tunnel: w1850 -> [w1851 w1855]
                    tunnel: [w1851 w1854] -> w1849
                    tunnel: w1846 -> [_ w1853]
                    tunnel: w1845 -> [_ w1852]
                    frame False {
                    }
                    frame True {
                      n785 = call "apply_matrix_transformation_to_spots.vi"("Transform centre (i.e. transform about this point)"=w1853, "Transformation Matrix (3x3)"=w1852, "Spot In"=w1855) -> ("Spot Out"=w1854:T1)  [unwired: 5 out]
                    }
                  }
                }
              }
            }
          }
        }
        "Selection/Group" <- w1527
        n786 = Unbundle By Name(w1534) -> ("Position (Image Pixels)"=w1533:cluster{"X":dbl, "Y":dbl})
        n787 = Bundle By Name(cluster=w1534, "Dragging"=TRUE, "Previous Position (Image Pixels)"=w1533, "Position (Image Pixels)"=w1532) -> (w1543:T10)
      }
      event "stop": Value Change {
        n788 = event-data() -> ()  [unwired: 1 in, 4 out]
        n789 = global read "red_tweezers_globals_INTERNAL_VOLATILE.vi" "Current Settings File"() -> (w1859:path)
        n790 = call <vilib>:"Check if File or Folder Exists.vi"("path"=w1859) -> ("file or folder exists?"=w1858:bool)  [unwired: 8 in, 2 out]
        n791 = case shown="False" w1858 {
          tunnel: [w1866 w1870] -> w1860
          frame False {
            n792 = Two Button Dialog(message="Save current settings?", 1:"Don't Save" ("F button name (\"Cancel\")"), 2:"Save As..." ("T button name (\"OK\")")) -> (T button?=w1863:bool)
            n793 = Select(t=T14."Center Button" ("Which Button?"), s=w1863, f=T14."Right Button" ("Which Button?")) -> (s? t:f=w1866:T14)
          }
          frame True {
            n794 = call <vilib>:"Three Button Dialog.vi"("Allow user to close window? (TRUE)"=TRUE, "Window Title (\"\")"="Save Settings?" ("Window Title (\"\")"), "Right Button Text (\"Cancel\")"="No" ("Right Button Text (\"Cancel\")"), "Center Button Text (\"No\")"="Save As..." ("Center Button Text (\"No\")"), "Left Button Text (\"Yes\")"="Save" ("Left Button Text (\"Yes\")"), "message"="Would you like to save the current settings? You can choose to use the current settings file or save to a new location.") -> ("Which Button?"=w1870:T14)  [unwired: 5 in]
          }
        }
        n795 = case shown="\"Center Button\"" w1860 {
          tunnel: [TRUE TRUE FALSE FALSE] -> w1857
          frame "Left Button", Default {
          }
          frame "Center Button" {
            n796 = call "File Dialog5"("prompt"="Please select a location to save the settings", "button label"="Save", "default name"="red_tweezers_settings.xml", "pattern (all files)"="*.xml" ("pattern label"), "pattern label"="XML Settings Files") -> ("selected path"=w1878:path)  [unwired: 7 in, 3 out]
            n797 = global write "red_tweezers_globals_INTERNAL_VOLATILE.vi" "Current Settings File"(w1878) -> ()
          }
          frame "Right Button" {
          }
          frame "Window Close" {
          }
        }
        n798 = global write "red_tweezers_globals_INTERNAL_VOLATILE.vi" "Save Settings On Exit"(w1857) -> ()
      }
    }
    n799 = case shown="True" "Play" {
      frame False {
      }
      frame True {
        n800 = stacked-sequence {
          frame #0 {
            n801 = local read "NewXYArray"() -> (w150:dbl[][])
            n802 = Array Size(array=w150) -> (size(s)=w151:i32[])
            n803 = Index Array(array=w151, index=0) -> (element=w153:i32)
            "NewXYArraySize" <- w153
            n804 = for {
              N: w153 -> [w156]
              i -> [w155]
              stop <- w154 stop-if-true
              n805 = stacked-sequence {
                tunnel: w156 -> [_ w161]
                tunnel: w155 -> [_ w160]
                tunnel: [w157 _] -> w154
                frame #0 {
                  n806 = local read "Insert"() -> (w157:bool)
                  n807 = local write "Insert"(TRUE) -> ()
                }
                frame #1 {
                  n808 = local write "Locked Current Spot"(w160) -> ()
                  n809 = local write "# of Spots"(w161) -> ()
                  n810 = local write "Rates"(1) -> ()
                  n811 = local write "LCS"(0) -> ()
                }
              }
            }
          }
          frame #1 {
            w163 = TRUE
            w164 = 1
            n812 = local write "Insert"(w163) -> ()
            n813 = stacked-sequence {
              frame #0 {
                n814 = local read "toply"() -> (w170:dbl)
                n815 = local read "Bubble x"() -> (w171:dbl)
                n816 = Bundle("Bubble x"=w171, "toply"=w170) -> (w169:cluster{"Bubble x":dbl, "toply":dbl})  [unwired: 1 in]
                n817 = local read "NewXYArray"() -> (w172:dbl[][])
                n818 = Cluster To Array(cluster=w169) -> (array=w168:dbl[])
                n819 = Insert Into Array(array=w172, index (row)=0, new element=w168) -> (w166:dbl[][])  [unwired: 1 in]
                n820 = local write "NewXYArray"(w166) -> ()
              }
              frame #1 {
                n821 = local read "Bubble x"() -> (w179:dbl)
                n822 = local read "bottomry"() -> (w178:dbl)
                n823 = Bundle("Bubble x"=w179, "bottomry"=w178) -> (w177:cluster{"Bubble x":dbl, "bottomry":dbl})  [unwired: 1 in]
                n824 = local read "NewXYArray"() -> (w176:dbl[][])
                n825 = Cluster To Array(cluster=w177) -> (array=w175:dbl[])
                n826 = Insert Into Array(array=w176, index (row)=1, new element=w175) -> (w173:dbl[][])  [unwired: 1 in]
                n827 = local write "NewXYArray"(w173) -> ()
              }
              frame #2 {
                n828 = local read "bottomrx"() -> (w186:dbl)
                n829 = local read "Bubble y"() -> (w185:dbl)
                n830 = Bundle("bottomrx"=w186, "Bubble y"=w185) -> (w184:cluster{"bottomrx":dbl, "Bubble y":dbl})  [unwired: 1 in]
                n831 = local read "NewXYArray"() -> (w182:dbl[][])
                n832 = Cluster To Array(cluster=w184) -> (array=w183:dbl[])
                n833 = Insert Into Array(array=w182, index (row)=2, new element=w183) -> (w180:dbl[][])  [unwired: 1 in]
                n834 = local write "NewXYArray"(w180) -> ()
              }
              frame #3 {
                n835 = local read "Bubble y"() -> (w192:dbl)
                n836 = local read "toplx"() -> (w193:dbl)
                n837 = Bundle("toplx"=w193, "Bubble y"=w192) -> (w191:cluster{"toplx":dbl, "Bubble y":dbl})  [unwired: 1 in]
                n838 = Cluster To Array(cluster=w191) -> (array=w190:dbl[])
                n839 = local read "NewXYArray"() -> (w189:dbl[][])
                n840 = Insert Into Array(array=w189, index (row)=3, new element=w190) -> (w187:dbl[][])  [unwired: 1 in]
                n841 = local write "NewXYArray"(w187) -> ()
              }
            }
            "Max Number of Bubbles 2" <- 4
            "Initiate Creation 2" <- w164
            "LCS" <- w164
            "Rates" <- w164
            "Play Pressed" <- w163
          }
        }
      }
    }
    n842 = call "IMAQ Create"("Image Name"="untitled", "Image Type"=w48) -> ("New Image"=w47:T8)  [unwired: 3 in, 1 out]
    n843 = call "Vision Acquisition"() -> ("Image Out"=w45:T8)  [unwired: 26 in, 1 out]
    n844 = local read "Number of Matches Returned"() -> (w39:dbl)
    n845 = case shown="True" "Camera Capture" {
      frame False {
      }
      frame True {
        n846 = local read "Circles"() -> (w198:T9)
        n847 = Index Array(array=w198) -> (element=w197:T24)  [unwired: 1 in]
        n848 = Unbundle(w197) -> ("Position"=w196:cluster{"X":sgl, "Y":sgl})  [unwired: 2 out]
        n849 = Unbundle(w196) -> ("X"=→"Bubble x":sgl, "Y"=→"Bubble y":sgl)
      }
    }
    n850 = Add(x=w39, y=1.0 ("x+y")) -> (x+y=w41:dbl)
    n851 = call "IMAQ ExtractSingleColorPlane"("Color Plane"=w44, "Image Dst"=w47, "Image Src"=w45) -> ("Image Dst Out"=w42:T8)  [unwired: 7 in, 1 out]
    n852 = for {
      N: w41 -> [_]
      tunnel: w42 -> [w207]
      i -> [w203]
      n853 = local read "Circles"() -> (w219:T9)
      n854 = Number To Decimal String(number=w203) -> (decimal integer string=w202:string)  [unwired: 1 in]
      n855 = Index Array(array=w219) -> (element=w218:T24)  [unwired: 1 in]
      n856 = Unbundle(w218) -> ("Position"=w201:cluster{"X":sgl, "Y":sgl}, "Radius"=w217:dbl)  [unwired: 1 out]
      n857 = Unbundle(w201) -> ("X"=w205:sgl, "Y"=w204:sgl)
      n858 = Subtract(x=w205, y=w217) -> (x-y=→"toplx":dbl)
      n859 = Add(x=w205, y=w217) -> (x+y=→"bottomrx":dbl)
      n860 = Add(x=w204, y=w217) -> (x+y=→"bottomry":dbl)
      n861 = Subtract(x=w204, y=w217) -> (x-y=→"toply":dbl)
      n862 = local read "bottomry"() -> (w209:dbl)
      n863 = local read "bottomrx"() -> (w210:dbl)
      n864 = local read "toply"() -> (w211:dbl)
      n865 = local read "toplx"() -> (w212:dbl)
      n866 = Build Array(w212, w211, w210, w209) -> (w206:dbl[])
      n867 = Array To Cluster(array=w206) -> (cluster=w208:T25)
      n868 = call "IMAQ Overlay Oval"("Bounding Rectangle"=w208, "Image"=w207) -> ("Image Out"=w200:T8)  [unwired: 8 in, 1 out]
      n869 = call "IMAQ Overlay Text"("String"=w202, "Origin"=w201, "Image"=w200) -> ("Image Out"=→"Camera 2":T8)  [unwired: 7 in, 1 out]
    }
    n870 = case shown="True" "Lock Current Spot" {
      frame False {
      }
      frame True {
        n871 = global read "red_tweezers_globals.vi" "Spots"() -> (w430:T1[])
        n872 = local read "Current Spot #"() -> (w431:dbl)
        "Locked Current Spot" <- w431
        n873 = Index Array(array=w430, index=w431) -> (element=w432:T1)
        n874 = local write "LCS"(0) -> ()
        n875 = Unbundle By Name(w432) -> ("Position.x"=→"LCS X":dbl, "Position.y"=→"LCS Y":dbl)
      }
    }
    n876 = call-poly "IMAQ Detect Shapes"("Image"=w42) -> ("Number of Matches Returned"=→"Number of Matches Returned":i32, "Circles"=→"Circles":T9)  [unwired: 8 in, 1 out]
    n877 = case shown="True" "Mark Original Position" {
      frame False {
      }
      frame True {
        w433 = TRUE
        n878 = local write "Mark Original Position"(FALSE) -> ()
        n879 = local read "New X"() -> (→"Original X":dbl)
        n880 = local read "New Y"() -> (→"Original Y":dbl)
        "MOP pressed After" <- w433
        "MOP pressed" <- w433
      }
    }
    n881 = local read "Rates"() -> (w52:dbl)
    n882 = Equal?(x=w52, y=1.0) -> (x = y?=w50:bool)
    n883 = case shown="True" "Send Data" {
      frame False {
      }
      frame True {
        # "Pass data from Image Assistant to \nRed Tweezer New X & Y position"
        n884 = local read "Bubble y"() -> (w220:dbl)
        n885 = local read "Bubble x"() -> (w221:dbl)
        n886 = local write "New Y"(w220) -> ()
        n887 = local write "New X"(w221) -> ()
      }
    }
    n888 = case shown="True" w50 {
      frame False {
      }
      frame True {
        n889 = stacked-sequence {
          frame #0 {
            n890 = local read "Tab Control"() -> (w303:enum32{"Line", "Arc"})
            n891 = case shown="\"Line\"" w303 {
              tunnel: "Number of Planned Sequence Frames 2" -> [w304 w323]
              frame "Arc" {
                n892 = stacked-sequence {
                  tunnel: w304 -> [_ w317 _]
                  frame #0 {
                    n893 = expression code="(x/180.0)*pi" "degrees to radians"("Theta") -> (→"Radians":dbl)
                    n894 = local read "Radians"() -> (w316:dbl)
                    n895 = local read "Original Y"() -> (w310:dbl)
                    n896 = local read "Original X"() -> (w308:dbl)
                    n897 = Cosine(x=w316) -> (cos(x)=w305:dbl)
                    n898 = Sine(x=w316) -> (sin(x)=w307:dbl)
                    n899 = Multiply(x=w305, y="Radius X") -> (x*y=w309:dbl)
                    n900 = Multiply(x="Radius X", y=w307) -> (x*y=w311:dbl)
                    n901 = Subtract(x=w308, y=w309) -> (x-y=→"Center X":dbl)
                    n902 = Subtract(x=w310, y=w311) -> (x-y=→"Center Y":dbl)
                  }
                  frame #1 {
                    n903 = local read "Radians"() -> (w321:dbl)
                    n904 = Subtract(x=w317, y=1) -> (x-y=w319:dbl)
                    n905 = Divide(x=w321, y=w319) -> (x/y=→"Degree Rate":dbl)
                  }
                  frame #2 {
                  }
                }
              }
              frame "Line" {
                n906 = local read "Max Number of Bubbles 2"() -> (w322:dbl)
                n907 = for {
                  N: w322 -> [_]
                  tunnel: w323 -> [w325]
                  i -> [w324]
                  n908 = stacked-sequence {
                    tunnel: w325 -> [_ w343]
                    tunnel: w324 -> [w330 w337]
                    frame #0 {
                      n909 = local read "NewXYArray"() -> (w331:dbl[][])
                      n910 = Index Array(array=w331, index (row)=w330) -> (element=w329:dbl[])  [unwired: 1 in]
                      n911 = Array To Cluster(array=w329) -> (cluster=w328:T26)
                      n912 = Unbundle By Name(w328) -> ("NewXYArray[0]"=w327:dbl, "NewXYArray[1]"=w326:dbl)
                      n913 = global read "red_tweezers_globals.vi" "Spots"() -> (w335:T1[])
                      n914 = Index Array(array=w335, index=w330) -> (element=w334:T1)
                      n915 = local write "New X"(w327) -> ()
                      n916 = local write "New Y"(w326) -> ()
                      n917 = Unbundle By Name(w334) -> ("Position.x"=w333:dbl, "Position.y"=w332:dbl)
                      n918 = local write "Original Y"(w332) -> ()
                      n919 = local write "Original X"(w333) -> ()
                    }
                    frame #1 {
                      n920 = local read "Original X"() -> (w351:dbl)
                      n921 = local read "Original Y"() -> (w349:dbl)
                      n922 = Subtract(x=w343, y=1) -> (x-y=w345:dbl)
                      n923 = local read "New Y"() -> (w348:dbl)
                      n924 = local read "New X"() -> (w350:dbl)
                      n925 = Subtract(x=w349, y=w348) -> (x-y=w346:dbl)
                      n926 = Subtract(x=w351, y=w350) -> (x-y=w347:dbl)
                      n927 = Divide(x=w346, y=w345) -> (x/y=w341:dbl)
                      "Y Rate" <- w341
                      n928 = Divide(x=w347, y=w345) -> (x/y=w342:dbl)
                      "X Rate" <- w342
                      n929 = Bundle(w342, w341) -> (w340:cluster{dbl, dbl})  [unwired: 1 in]
                      n930 = local read "NewXYRates"() -> (w338:dbl[][])
                      n931 = Cluster To Array(cluster=w340) -> (array=w339:dbl[])
                      n932 = Insert Into Array(array=w338, index (row)=w337, new element=w339) -> (→"NewXYRates":dbl[][])  [unwired: 1 in]
                    }
                  }
                }
              }
            }
          }
          frame #1 {
            n933 = local write "Rates"(0) -> ()
          }
        }
      }
    }
    n934 = local read "Sequence Instances"() -> (w108:dbl)
    n935 = case shown="True" w127 {
      tunnel: w133 -> [_ w499]
      frame False {
      }
      frame True {
        n936 = global write "red_tweezers_globals_INTERNAL.vi" "Image Overlay (extras from control loop)"(w499) -> ()
      }
    }
    n937 = local read "Counter"() -> (w107:dbl)
    n938 = call "red_tweezers_UNDO.vi"("Force Save"=w129, "This change is inconsequential (don't save it)"=w130, "Selection/Group"=w131, "Spots"=w132) -> ()  [unwired: 6 in, 2 out]
    n939 = call "sync_with_globals.vi"("Selection/Group"=w131, "Spots"=w132) -> ("Selection/Group 2"=w143:T7[], "Spots 2"=w94:T1[])  [unwired: 4 in]
    n940 = local read "Sequence Storer"() -> (w103:T1[][])
    n941 = local read "Sequence On?"() -> (w106:bool)
    n942 = local read "Sequence On?"() -> (w121:bool)
    n943 = call "SequenceControl.vi"("Sequence On? 2"=w106, "Counter 2"=w107, "Sequence Instances 2"=w108, "Sequence Storer"=w103) -> ("Time per Frame (ms) 2"=w101:dbl, "Sequence Order 2"=w104:dbl, "Reset 2"=w105:bool, "Sequence Storer 2"=w116:T1[][], "Clearance Button 2"=w115:bool, "Manual Edit 2"=w114:bool, "Save State 2"=w113:bool, "Play Sequence 2"=w110:bool, "Bubble ID to Empty 2"=w109:dbl, "Manual Sequence 2"=w111:bool, "Edit Sequence Mode 2"=w112:bool)  [unwired: 1 in]
    n944 = local write "Play Sequence"(w110) -> ()
    n945 = local write "Bubble ID to Empty"(w109) -> ()
    n946 = local write "Manual Sequence"(w111) -> ()
    n947 = local write "Reset"(w105) -> ()
    n948 = local write "Edit Sequence Mode"(w112) -> ()
    n949 = local write "Clearance Button"(w115) -> ()
    n950 = local write "Sequence Storer"(w116) -> ()
    n951 = local write "Save State"(w113) -> ()
    n952 = local write "Manual Edit"(w114) -> ()
    n953 = Or(x=w121, y="Manual Sequence") -> (x .or. y?=w120:bool)
    n954 = local write "Time per Frame (ms)"(w101) -> ()
    n955 = case shown="False" w120 {
      tunnel: [w469 w474] -> w124
      tunnel: w94 -> [w468 _]
      frame False {
        n956 = Or(x="Manual Edit", y="Edit Sequence Mode") -> (x .or. y?=w467:bool)
        n957 = case shown="False" w467 {
          tunnel: w468 -> [w470 _]
          tunnel: [w470 w471] -> w469
          frame False {
          }
          frame True {
            n958 = local read "Sequence Order"() -> (w472:dbl)
            n959 = local read "Sequence Storer"() -> (w473:T1[][])
            n960 = Index Array(array=w473, index (row)=w472) -> (element=w471:T1[])  [unwired: 1 in]
          }
        }
      }
      frame True {
        n961 = stacked-sequence {
          tunnel: [w476 _] -> w474
          frame #0 {
            n962 = local read "Counter"() -> (w477:dbl)
            n963 = local read "Sequence Storer"() -> (w478:T1[][])
            n964 = Index Array(array=w478, index (row)=w477) -> (element=w476:T1[])  [unwired: 1 in]
            n965 = Wait (ms)(milliseconds to wait="Time per Frame (ms)") -> ()  [unwired: 1 out]
          }
          frame #1 {
            n966 = local read "Sequence Instances"() -> (w480:dbl)
            n967 = local read "Counter"() -> (w483:dbl)
            n968 = Subtract(x=w480, y=1) -> (x-y=w481:dbl)
            n969 = Equal?(x=w483, y=w481) -> (x = y?=w482:bool)
            n970 = case shown="True" w482 {
              frame False {
                n971 = local read "Counter"() -> (w486:dbl)
                n972 = Add(x=w486, y=1) -> (x+y=→"Counter":dbl)
              }
              frame True {
                w487 = FALSE
                n973 = local write "Counter"(0) -> ()
                n974 = local write "Play Sequence"(w487) -> ()
                n975 = local write "Sequence On?"(w487) -> ()
              }
            }
          }
        }
      }
    }
    n976 = case shown="True" "Save State" {
      tunnel: w94 -> [_ w490]
      frame False {
      }
      frame True {
        n977 = local write "Save State"(FALSE) -> ()
        n978 = stacked-sequence {
          tunnel: w490 -> [w491 _]
          frame #0 {
            "Spot Storage" <- w491
          }
          frame #1 {
            n979 = local read "Spot Storage"() -> (w497:T1[])
            n980 = Replace Array Subset(array="Sequence Storer", new element=w497, index (row)="Sequence Order") -> (w495:T1[][])  [unwired: 1 in]
            n981 = Array Size(array=w495) -> (size(s)=w494:i32[])
            n982 = local write "Sequence Storer"(w495) -> ()
            n983 = Index Array(array=w494, index=0) -> (element=→"Sequence Instances":i32)
          }
        }
      }
    }
    n984 = feedback #10() -> (w148:T27)  [unwired: 1 out]
    n985 = call "Smoothed Frame Rate.vi"("Feedback In"=w148) -> ("Feedback Out"=w147:T27, "Frame Rate"=→"Interface Frame Rate":dbl)  [unwired: 1 in, 4 out]
    n986 = feedback-in #10(w147) -> ()
    n987 = local write "Sequence Order"(w104) -> ()
    n988 = case shown="True" "Clearance Button" {
      frame False {
      }
      frame True {
        # "This is the Bubble ID to Empty tool- this \"deletes\" the bubble in a sequence."
        n989 = local read "Sequence Order"() -> (w460:dbl)
        n990 = local read "Sequence Storer"() -> (w461:T1[][])
        n991 = Replace Array Subset(array=w461, new element=T11 {"Position"={"x"=nan, "y"=nan, "z"=nan}, "Intensity"=1.0, "Vortex Charge"=1, "Phase"=1.0, "NA Position"={"x"=0.0, "y"=0.0, "r"=1.0}, "Line Trapping"={"Vector"={"x"=0.0, "y"=0.0, "z"=0.0}, "Phase Gradient"=0.0}, "Amplitude Correction"=0.0} ("Cluster"), index (row)=w460, index (col)="Bubble ID to Empty") -> (w457:T1[][])
        n992 = local write "Sequence Storer"(w457) -> ()
      }
    }
    n993 = Not(x=w97) -> (.not. x?=w98:bool)
    n994 = Not(x="Output to SLM") -> (.not. x?=w99:bool)
    n995 = case shown="True" "Save" {
      frame False {
      }
      frame True {
        n996 = local read "Sequence Storer"() -> (w426:T1[][])
        n997 = call "SequenceSaver.vi"("Sequence Storer"=w426) -> ()  [unwired: 10 in, 1 out]
      }
    }
    n998 = And(x=w99, y=w98) -> (x .and. y?=w102:bool)
    n999 = case shown="True" "Load" {
      frame False {
      }
      frame True {
        n1000 = call "SequenceSaver.vi"() -> ("Sequence Storer 2"=w425:T1[][])  [unwired: 11 in]
        n1001 = local write "Sequence Storer"(w425) -> ()
      }
    }
    n1002 = local read "Initiate Creation 2"() -> (w55:dbl)
    n1003 = case shown="True" w102 {
      tunnel: w94 -> [w1887 _]
      frame False {
        n1004 = call "UDP Sender generic_2.vi"("Spots"=w1887) -> ()  [unwired: 2 in, 1 out]
      }
      frame True {
      }
    }
    n1005 = case shown="True" "Reset" {
      frame False {
      }
      frame True {
        n1006 = local write "Counter"(0) -> ()
      }
    }
    n1007 = case shown="True" "Add Additional Frames" {
      frame False {
      }
      frame True {
        # "This adds additional frames to the sequence."
        n1008 = for {
          N: "Additional Frames Wanted" -> [_]
          i -> [w439]
          n1009 = local read "Max Number of Bubbles 2"() -> (w443:dbl)
          n1010 = Add(x=1, y=w439) -> (x+y=w440:i32)
          n1011 = Add(x="Frame Location", y=w440) -> (x+y=w441:dbl)
          n1012 = Initialize Array(T11 {"Position"={"x"=nan, "y"=nan, "z"=nan}, "Intensity"=1.0, "Vortex Charge"=1, "Phase"=1.0, "NA Position"={"x"=0.0, "y"=0.0, "r"=1.0}, "Line Trapping"={"Vector"={"x"=0.0, "y"=0.0, "z"=0.0}, "Phase Gradient"=0.0}, "Amplitude Correction"=0.0} ("Cluster"), w443) -> (w444:T28)
          n1013 = local read "Sequence Storer"() -> (w445:T1[][])
          n1014 = Insert Into Array(array=w445, index (row)=w441, new element=w444) -> (w446:T1[][])  [unwired: 1 in]
          n1015 = local write "Sequence Storer"(w446) -> ()
        }
      }
    }
    n1016 = case shown="1" w55 {
      frame 0, Default {
      }
      frame 1 {
        # "This create the array needed for a sequential\narray."
        n1017 = local read "Number of Planned Sequence Frames 2"() -> (w450:dbl)
        n1018 = local read "Max Number of Bubbles 2"() -> (w449:dbl)
        n1019 = for {
          N: w450 -> [_]
          tunnel: w449 -> [w451]
          i -> [w454]
          n1020 = Initialize Array(T11 {"Position"={"x"=nan, "y"=nan, "z"=nan}, "Intensity"=1.0, "Vortex Charge"=1, "Phase"=1.0, "NA Position"={"x"=0.0, "y"=0.0, "r"=1.0}, "Line Trapping"={"Vector"={"x"=0.0, "y"=0.0, "z"=0.0}, "Phase Gradient"=0.0}, "Amplitude Correction"=0.0} ("Cluster"), w451) -> (w452:T28)
          n1021 = local read "Sequence Storer"() -> (w455:T1[][])
          n1022 = Insert Into Array(array=w455, index (row)=w454, new element=w452) -> (w456:T1[][])  [unwired: 1 in]
          n1023 = local write "Sequence Storer"(w456) -> ()
        }
        n1024 = local write "Initiate Creation 2"(0) -> ()
      }
    }
    n1025 = case shown="False" "Play Sequence" {
      frame False {
        n1026 = local write "Sequence On?"(FALSE) -> ()
      }
      frame True {
        "Sequence On?" <- TRUE
      }
    }
    n1027 = local read "Current Spot #"() -> (w77:dbl)
    n1028 = local read "Selection/Group"() -> (w78:T7[])
    n1029 = local read "# of Spots"() -> (w93:dbl)
    n1030 = Not Equal?(x=w77, y=-1) -> (x != y?=w79:bool)
    n1031 = local read "spots selected 2"() -> (w67:i32)
    n1032 = Index Array(array=w78, index=w77) -> (element=w76:T7)
    n1033 = Unbundle By Name(w76) -> ("Selected"=w75:bool)
    n1034 = local read "spots selected"() -> (w68:i32)
    n1035 = Not(x=w75) -> (.not. x?=w74:bool)
    n1036 = And(x=w74, y=w79) -> (x .and. y?=w69:bool)
    n1037 = Less?(x=w68, y=w67) -> (x < y?=w65:bool)
    n1038 = case shown="True" "Insert" {
      tunnel: w94 -> [_ w223]
      tunnel: w93 -> [_ w222]
      frame False {
      }
      frame True {
        n1039 = for {
          N: w222 -> [_]
          tunnel: w223 -> [w225]
          i -> [w224]
          n1040 = stacked-sequence {
            tunnel: w225 -> [w227 w232 _]
            tunnel: w224 -> [_ w228 _]
            frame #0 {
              n1041 = local read "Start at Which Frame?"() -> (→"Num":dbl)
              "Spot Storage 2" <- w227
            }
            frame #1 {
              n1042 = local read "Selection/Group"() -> (w231:T7[])
              n1043 = Index Array(array=w231, index=w228) -> (element=w230:T7)
              n1044 = Unbundle By Name(w230) -> ("Selected"=w229:bool)
              n1045 = case shown="True" w229 {
                tunnel: w232 -> [_ _]
                frame False {
                }
                frame True {
                  n1046 = stacked-sequence {
                    frame #0 {
                      n1047 = case shown="\"Line\"" "Tab Control" {
                        frame "Arc" {
                          n1048 = local read "Number of Planned Sequence Frames 2"() -> (w236:dbl)
                          n1049 = Subtract(x=w236, y=1) -> (x-y=w234:dbl)
                          n1050 = for {
                            N: w236 -> [_]
                            tunnel: w234 -> [w237]
                            i -> [w239]
                            # "What is this ^\n\nFor # of sequence\nframes, don't worry\nabout it"
                            # "How to make position x and y?\nIt's called a cluster, inser the new position to Position.x and Position.y"
                            n1051 = Equal?(x=w237, y=w239) -> (x = y?=w238:bool)
                            n1052 = case shown="False" w238 {
                              tunnel: [w262 w271] -> w241
                              tunnel: [w261 w270] -> w240
                              tunnel: w239 -> [w258 _]
                              frame False {
                                # "calculating new position"
                                n1053 = local read "Degree Rate"() -> (w260:dbl)
                                n1054 = Multiply(x=w260, y=w258) -> (x*y=w259:dbl)
                                n1055 = Cosine(x=w259) -> (cos(x)=w268:dbl)
                                n1056 = Sine(x=w259) -> (sin(x)=w269:dbl)
                                n1057 = local read "Radius X"() -> (w267:dbl)
                                n1058 = Multiply(x=w267, y=w269) -> (x*y=w266:dbl)
                                n1059 = Multiply(x=w268, y=w267) -> (x*y=w265:dbl)
                                n1060 = local read "Center X"() -> (w264:dbl)
                                n1061 = local read "Center Y"() -> (w263:dbl)
                                n1062 = Add(x=w264, y=w265) -> (x+y=w262:dbl)
                                n1063 = Add(x=w263, y=w266) -> (x+y=w261:dbl)
                              }
                              frame True {
                                n1064 = global read "red_tweezers_globals.vi" "Spots"() -> (w274:T1[])
                                n1065 = local read "Numeric"() -> (w273:dbl)
                                n1066 = Index Array(array=w274, index=w273) -> (element=w272:T1)
                                n1067 = Unbundle By Name(w272) -> ("Position.x"=w271:dbl, "Position.y"=w270:dbl)
                              }
                            }
                            n1068 = local read "Spot Storage 2"() -> (w257:T1[])
                            n1069 = local read "Numeric"() -> (w256:dbl)
                            n1070 = Index Array(array=w257, index=w256) -> (element=w243:T1)
                            n1071 = local read "Start at Which Frame?"() -> (w245:dbl)
                            n1072 = Bundle By Name(cluster=w243, "Position.x"=w241, "Position.y"=w240) -> (w242:T1)
                            n1073 = local read "Number of Planned Sequence Frames 2"() -> (w244:dbl)
                            n1074 = Subtract(x=w245, y=w239) -> (x-y=w254:dbl)
                            n1075 = local read "Sequence Storer"() -> (w255:T1[][])
                            n1076 = local read "Numeric"() -> (w250:dbl)
                            n1077 = Add(x=w254, y=w244) -> (x+y=w253:dbl)
                            n1078 = Subtract(x=w253, y=1) -> (x-y=w251:dbl)
                            n1079 = Replace Array Subset(array=w255, new element=w242, index (row)=w251, index (col)=w250) -> (w249:T1[][])
                            n1080 = Array Size(array=w249) -> (size(s)=w248:i32[])
                            n1081 = local write "Sequence Storer"(w249) -> ()
                            n1082 = Index Array(array=w248, index=0) -> (element=w246:i32)
                            n1083 = local write "Sequence Instances"(w246) -> ()
                          }
                        }
                        frame "Line" {
                          # "This is the automatic sequence generator which allows for the creation of the sequence. This calculates the LAST coordinates of each bubble first\nbefore going for the first few coordinates of the sequence."
                          n1084 = local read "Number of Planned Sequence Frames 2"() -> (w275:dbl)
                          n1085 = for {
                            N: w275 -> [_]
                            i -> [w278]
                            # "For why do we multiply?"
                            n1086 = local read "Spot Storage 2"() -> (w293:T1[])
                            n1087 = local read "Numeric"() -> (w283:dbl)
                            n1088 = local read "NewXYRates"() -> (w284:dbl[][])
                            n1089 = Index Array(array=w293, index=w283) -> (element=w291:T1)
                            n1090 = Index Array(array=w284, index (row)=w283, index (col)=1) -> (element=w279:dbl)
                            n1091 = Index Array(array=w284, index (row)=w283, index (col)=0) -> (element=w280:dbl)
                            n1092 = Unbundle By Name(w291) -> ("Position.x"=w298:dbl, "Position.y"=w296:dbl)
                            n1093 = Multiply(x=w280, y=w278) -> (x*y=w297:dbl)
                            n1094 = Multiply(x=w279, y=w278) -> (x*y=w292:dbl)
                            "probe" <- w292
                            n1095 = Subtract(x=w298, y=w297) -> (x-y=w295:dbl)
                            n1096 = Subtract(x=w296, y=w292) -> (x-y=w294:dbl)
                            n1097 = Bundle By Name(cluster=w291, "Position.x"=w295, "Position.y"=w294) -> (w286:T1)
                            n1098 = Add(x="Start at Which Frame?", y=w278) -> (x+y=w276:dbl)
                            n1099 = local read "Sequence Storer"() -> (w299:T1[][])
                            n1100 = local read "Numeric"() -> (w285:dbl)
                            n1101 = Replace Array Subset(array=w299, new element=w286, index (row)=w276, index (col)=w285) -> (w290:T1[][])
                            n1102 = Array Size(array=w290) -> (size(s)=w289:i32[])
                            n1103 = local write "Sequence Storer"(w290) -> ()
                            n1104 = Index Array(array=w289, index=0) -> (element=w287:i32)
                            n1105 = local write "Sequence Instances"(w287) -> ()
                          }
                        }
                      }
                    }
                    frame #1 {
                      n1106 = local write "Play Pressed"(FALSE) -> ()
                    }
                  }
                }
              }
              "Numeric" <- w228
            }
            frame #2 {
              n1107 = local write "Insert"(FALSE) -> ()
            }
          }
        }
      }
    }
    n1108 = And(x=w65, y=w69) -> (x .and. y?=w70:bool)
    n1109 = case shown="True" w70 {
      frame False {
      }
      frame True {
        n1110 = local read "# of Spots"() -> (w360:dbl)
        n1111 = for {
          N: w360 -> [_]
          i -> [w362]
          stop <- w361 stop-if-true
          n1112 = local read "Selection/Group"() -> (w364:T7[])
          n1113 = Index Array(array=w364, index=w362) -> (element=w363:T7)
          n1114 = Unbundle By Name(w363) -> ("Selected"=w361:bool)
          n1115 = case shown="True" w361 {
            tunnel: w362 -> [_ w366]
            frame False {
            }
            frame True {
              n1116 = local write "Current Spot #"(w366) -> ()
              "Induce check" <- TRUE
            }
          }
        }
      }
    }
    n1117 = local read "spots selected"() -> (w80:i32)
    n1118 = local read "spots selected 2"() -> (w81:i32)
    n1119 = local read "Prev Current Spot"() -> (w89:dbl)
    n1120 = local read "Current Spot #"() -> (w90:dbl)
    n1121 = Not Equal?(x=w90, y=w89) -> (x != y?=w88:bool)
    n1122 = Greater?(x=w81, y=w80) -> (0:w82:bool)
    n1123 = local read "Induce check"() -> (w71:bool)
    n1124 = Or(x=w88, y=w82) -> (x .or. y?=w73:bool)
    n1125 = Or(x=w73, y=w71) -> (x .or. y?=w72:bool)
    n1126 = case shown="True" w72 {
      frame False {
      }
      frame True {
        n1127 = stacked-sequence {
          frame #0 {
            # "A small 100 ms delay is given to provide enough time for the data to be processed properly."
            n1128 = local read "Null array"() -> (w372:dbl[])
            n1129 = local write "What to Check"(w372) -> ()
            n1130 = local write "ID"(w372) -> ()
            n1131 = local read "Current Spot #"() -> (w374:dbl)
            n1132 = local write "Potential Collisions"(0) -> ()
            n1133 = local read "Spot Checker"() -> (w373:T1[])
            n1134 = Index Array(array=w373, index=w374) -> (element=w375:T1)
            n1135 = Wait (ms)(milliseconds to wait=10) -> ()  [unwired: 1 out]
            n1136 = Unbundle By Name(w375) -> ("Position.x"=w369:dbl, "Position.y"=w370:dbl)
            n1137 = local write "Orig Y SC"(w370) -> ()
            n1138 = local write "Orig X SC"(w369) -> ()
            n1139 = local write "Induce check"(FALSE) -> ()
          }
          frame #1 {
            n1140 = local read "# of Spots"() -> (w376:dbl)
            n1141 = for {
              N: w376 -> [_]
              tunnel: w376 -> [w381]
              i -> [w377]
              n1142 = local read "Selection/Group"() -> (w380:T7[])
              n1143 = Index Array(array=w380, index=w377) -> (element=w379:T7)
              n1144 = Unbundle By Name(w379) -> ("Selected"=w378:bool)
              n1145 = case shown="True" w378 {
                tunnel: w381 -> [_ w383]
                tunnel: w377 -> [_ w382]
                frame False {
                }
                frame True {
                  n1146 = for {
                    N: w383 -> [_]
                    tunnel: w382 -> [w384]
                    i -> [w385]
                    # "If the bubble is not selected, find difference of bubble to bubble\nbeing checked"
                    n1147 = local read "Selection/Group"() -> (w389:T7[])
                    n1148 = Index Array(array=w389, index=w385) -> (element=w388:T7)
                    n1149 = Unbundle By Name(w388) -> ("Selected"=w386:bool)
                    n1150 = Not(x=w386) -> (.not. x?=w387:bool)
                    n1151 = case shown="True" w387 {
                      tunnel: w385 -> [_ w393]
                      tunnel: w384 -> [_ w392]
                      tunnel: w384 -> [_ w391]
                      frame False {
                      }
                      frame True {
                        n1152 = local read "Spot Checker"() -> (w410:T1[])
                        n1153 = Index Array(array=w410, index=w393) -> (element=w411:T1)
                        n1154 = Index Array(array=w410, index=w392) -> (element=w409:T1)
                        n1155 = Unbundle By Name(w409) -> ("Position.x"=w406:dbl, "Position.y"=w402:dbl)
                        n1156 = Unbundle By Name(w411) -> ("Position.x"=w403:dbl, "Position.y"=w399:dbl)
                        n1157 = local read "Area+ Buffer"() -> (w390:dbl)
                        n1158 = Subtract(x=w406, y=w390) -> (x-y=w407:dbl)
                        n1159 = Greater Or Equal?(x=w403, y=w407) -> (x >= y?=w408:bool)
                        n1160 = Add(x=w402, y=w390) -> (x+y=w401:dbl)
                        n1161 = Subtract(x=w402, y=w390) -> (x-y=w400:dbl)
                        n1162 = Add(x=w406, y=w390) -> (x+y=w404:dbl)
                        n1163 = Less Or Equal?(x=w399, y=w401) -> (x <= y?=w398:bool)
                        n1164 = Greater Or Equal?(x=w399, y=w400) -> (x >= y?=w397:bool)
                        n1165 = Less Or Equal?(x=w403, y=w404) -> (x <= y?=w405:bool)
                        n1166 = And(x=w408, y=w405) -> (x .and. y?=w395:bool)
                        n1167 = And(x=w398, y=w397) -> (x .and. y?=w396:bool)
                        n1168 = And(x=w395, y=w396) -> (x .and. y?=w394:bool)
                        n1169 = case shown="True" w394 {
                          tunnel: w393 -> [_ _]
                          tunnel: w393 -> [_ w413]
                          tunnel: w391 -> [_ w412]
                          frame False {
                          }
                          frame True {
                            n1170 = stacked-sequence {
                              tunnel: w413 -> [w414 _]
                              tunnel: w412 -> [w415 _]
                              frame #0 {
                                n1171 = local read "Potential Collisions"() -> (w418:dbl)
                                n1172 = local read "What to Check"() -> (w419:dbl[])
                                n1173 = Insert Into Array(array=w419, index=w418, new element=w414) -> (w420:dbl[])
                                n1174 = local read "ID"() -> (w417:dbl[])
                                n1175 = local write "What to Check"(w420) -> ()
                                n1176 = Insert Into Array(array=w417, index=w418, new element=w415) -> (w416:dbl[])
                                n1177 = local write "ID"(w416) -> ()
                              }
                              frame #1 {
                                n1178 = local read "Potential Collisions"() -> (w423:dbl)
                                n1179 = Add(x=w423, y=1) -> (x+y=w421:dbl)
                                n1180 = local write "Potential Collisions"(w421) -> ()
                              }
                            }
                          }
                        }
                      }
                    }
                  }
                }
              }
            }
          }
          frame #2 {
            n1181 = local read "Current Spot #"() -> (w424:dbl)
            n1182 = local write "Prev Current Spot"(w424) -> ()
          }
        }
      }
    }
    n1183 = local read "Buffer Zone"() -> (w86:dbl)
    n1184 = Multiply(x=w86, y=2) -> (x*y=w87:dbl)
    n1185 = Add(x="Area to check", y=w87) -> (x+y=→"Area+ Buffer":dbl)
    n1186 = feedback #11() -> (w59:dbl)  [unwired: 1 in]
    n1187 = Equal?(x=w59, y=10000) -> (x = y?=w60:bool)
    n1188 = call "Elapsed Time"("Reset"=w60) -> ("Elapsed Time (s)"=w58:dbl, "Time has Elapsed"=w63:bool)  [unwired: 11 in, 6 out]
    "Elapsed Time" <- w58
    n1189 = feedback-in #11(w58) -> ()
    n1190 = And(x="On", y=w63) -> (x .and. y?=w64:bool)
    n1191 = case shown="True" w64 {
      frame False {
      }
      frame True {
        n1192 = local read "Position"() -> (w359:cluster{"x":dbl, "y":dbl, "z":dbl})
        n1193 = Unbundle By Name(w359) -> ("x"=→"X Pos every 10 sec":dbl)
      }
    }
    n1194 = case shown="True" "OK Button" {
      frame False {
      }
      frame True {
        n1195 = script code="clear all;\nclc;\n\ng = gigecam('169.254.154.83');\n\ng.PixelFormat= 'BayerGR8'\n\nimg = snapshot(g);\n\nimshow(img);"() -> ()  [unwired: 1 in, 1 out]
      }
    }
    n1196 = case shown="True" "O Button" {
      frame False {
      }
      frame True {
        n1197 = script code="%\n    rslt = Hough1_data(img);\n\n    % Frame translation\n    %- omit this as of now \n    \n    % Control method\n    increment = 10; %assuming the diamiter of the agent around 20 pic \n    \n    %- NewLoc = [x,y] whose unit is px\n    %- update new location based on current location obtained by the camera\n    NewLoc(1)= rslt(1);\n    NewLoc(2)= rslt(2);\n    \n    \n    % Update microrobot location with NewLoc\n    % the single robot would move to oblique downword\n    \n    % wait seconds"() -> ("NewLoc"=w355:dbl[])  [unwired: 1 in, 1 out]
        n1198 = Index Array(array=w355, index=1) -> (element=→"Y":dbl)
        n1199 = Index Array(array=w355, index=0) -> (element=→"X":dbl)
      }
    }
    n1200 = Tick Count (ms)() -> (millisecond timer value=w36:u32)
  }
  n1201 = flat-sequence {
    tunnel: w9 -> [w1890]
    tunnel: w8 -> [w1889]
    tunnel: [w1888] -> w6
    frame #0 {
      n1202 = disable-structure shown="\"IMAQdx with ROI tool buttons (default)\"" {
        disable-tunnel: w1890 -> [_ _ _ _ _ _]
        disable-tunnel: w1889 -> [_ _ w1948 _ _ _]
        disable-tunnel: [_ _ w1947 _ _ _] -> w1888
        frame condition #0 {
          w1892 = u32 10 ("Number of buffers")
          (unwired) FALSE ("background subtraction")
          # "This subdiagram uses the IMAQ drivers, with a pre-allocated ringbuffer for images.  This is the code I use with my Mikrotron MC1362-CL"
          n1203 = call <vilib>:"IMAQ Init.vi"("Interface Name"="img0") -> ("IMAQ Session Out"=w1899:refnum<k11>)  [unwired: 9 in, 1 out]
          n1204 = call <vilib>:"IMAQ Configure List.vi"("Region of interest"="Global ROI (requires restart)", "Number of buffers"=w1892, "Continuous?"=enum16{"One-Shot", "Continuous"}."Continuous", "IMAQ Session In"=w1899) -> ("error out"=w1893:errorcluster, "IMAQ Session Out"=w1895:refnum<k11>)  [unwired: 6 in]
          n1205 = for {
            N: w1892 -> [_]
            tunnel: 0 ("Channel") -> [w1912]
            shift-right: [w1915] -> w1897
            shift-left: w1893 -> [w1911]
            shift-right: [w1914] -> w1896
            shift-left: w1895 -> [w1913]
            i -> [w1910]
            n1206 = Format Into String(format string="mikrotronbuffer%04d", w1910) -> (resulting string=w1908:string)  [unwired: 2 in, 1 out]
            n1207 = call "IMAQ Create"("Image Name"=w1908) -> ("New Image"=w1907:T8)  [unwired: 4 in, 1 out]
            n1208 = call <vilib>:"IMAQ Configure Buffer.vi"("Channel"=w1912, "error in (no error)"=w1911, "Buffer Number"=w1910, "Image In"=w1907, "IMAQ Session In"=w1913) -> ("error out"=w1915:errorcluster, "IMAQ Session Out"=w1914:refnum<k11>)  [unwired: 5 in]
          }
          n1209 = call <vilib>:"IMAQ Start.vi"("error in (no error)"=w1897, "IMAQ Session In"=w1896) -> ("error out"=w1903:errorcluster, "IMAQ Session Out"=w1904:refnum<k11>)  [unwired: 8 in]
          n1210 = call "IMAQ Create"("Image Name"="Red Tweezers live image") -> ("New Image"=w1905:T8)  [unwired: 3 in, 2 out]
          n1211 = while {
            tunnel: w1904 -> [w1923]
            tunnel: w1903 -> [w1922]
            tunnel: w1905 -> [_]
            tunnel: [w1924] -> w1901
            tunnel: [w1917] -> w1902
            i -> [w1919]
            stop <- w1925 stop-if-true
            n1212 = local read "stop"() -> (w1925:bool)
            n1213 = call <vilib>:"IMAQ Extract Buffer.vi"("error in (no error)"=w1922, "Buffer to extract"=w1919, "IMAQ Session In"=w1923) -> ("error out"=w1917:errorcluster, "Image Out"=w1916:T8, "IMAQ Session Out"=w1924:refnum<k11>)  [unwired: 3 in, 3 out]
            n1214 = call "imageQ_camera_hook.vi"("Image"=w1916) -> ()  [unwired: 11 in]
            n1215 = feedback #12() -> (w1920:T27)  [unwired: 1 in]
            n1216 = call "Smoothed Frame Rate.vi"("Feedback In"=w1920) -> ("Feedback Out"=w1921:T27, "Frame Rate"=w1918:dbl)  [unwired: 1 in, 4 out]
            n1217 = feedback-in #12(w1921) -> ()
            n1218 = global write "red_tweezers_globals_INTERNAL_VOLATILE.vi" "Video Frame Rate"(w1918) -> ()
          }
          n1219 = call <vilib>:"IMAQ Close.vi"("error in (no error)"=w1902, "IMAQ Session In"=w1901) -> ()  [unwired: 9 in, 1 out]
        }
        frame condition #1 {
          (unwired) FALSE ("background subtraction")
          # "This subdiagram acquires using the IMAQdx drivers.  This covers most FireWire and GigE cameras (at least the ones supporting the IIDC or GenICam standards)."
          n1220 = call <vilib>:"IMAQdx Open Camera.vi"("Session In"=T6 "dalsaGenie") -> ("error out"=w1928:errorcluster, "Session Out"=w1927:T6)  [unwired: 9 in]
          n1221 = call <vilib>:"IMAQdx Configure Grab.vi"("error in"=w1928, "Session In"=w1927) -> ("error out"=w1929:errorcluster, "Session Out"=w1930:T6)  [unwired: 8 in]
          n1222 = call "IMAQ Create"("Image Name"="Red Tweezers live image") -> ("New Image"=w1933:T8)  [unwired: 3 in, 2 out]
          n1223 = while {
            tunnel: w1930 -> [w1942]
            tunnel: w1929 -> [w1941]
            tunnel: w1933 -> [w1935]
            tunnel: [w1943] -> w1931
            tunnel: [w1937] -> w1932
            stop <- w1944 stop-if-true
            n1224 = local read "stop"() -> (w1944:bool)
            n1225 = call <vilib>:"IMAQdx Grab.vi"("error in"=w1941, "Image In"=w1935, "Session In"=w1942) -> ("error out"=w1937:errorcluster, "Image Out"=w1936:T8, "Session Out"=w1943:T6)  [unwired: 5 in, 1 out]
            n1226 = call "imageQ_camera_hook.vi"("Image"=w1936) -> ()  [unwired: 11 in]
            n1227 = feedback #13() -> (w1939:T27)  [unwired: 1 in]
            n1228 = call "Smoothed Frame Rate.vi"("Feedback In"=w1939) -> ("Feedback Out"=w1940:T27, "Frame Rate"=w1938:dbl)  [unwired: 1 in, 4 out]
            n1229 = feedback-in #13(w1940) -> ()
            n1230 = global write "red_tweezers_globals_INTERNAL_VOLATILE.vi" "Video Frame Rate"(w1938) -> ()
          }
          n1231 = call <vilib>:"IMAQdx Close Camera.vi"("error in"=w1932, "Session In"=w1931) -> ()  [unwired: 9 in, 1 out]
        }
        frame condition #2 {
          # "This subdiagram acquires using the IMAQdx drivers.  This covers most FireWire and GigE cameras (at least the ones supporting the IIDC or GenICam standards)."
          n1232 = call <vilib>:"IMAQdx Open Camera.vi"("Session In"="Camera") -> ("error out"=w1956:errorcluster, "Session Out"=w1955:T6)  [unwired: 9 in]
          n1233 = call <vilib>:"IMAQdx Configure Grab.vi"("error in"=w1956, "Session In"=w1955) -> ("error out"=w1952:errorcluster, "Session Out"=w1953:T6)  [unwired: 8 in]
          n1234 = call "IMAQ Create"("Image Name"="Red Tweezers live image") -> ("New Image"=w1950:T8)  [unwired: 3 in, 2 out]
          n1235 = call "IMAQdx_get_ROI.vi"("Session In"=w1953) -> ("ROI"=w1949:u32[], "Session Out"=w1951:T6)  [unwired: 8 in]
          n1236 = while {
            shift-right: [w1965] -> w1945
            shift-left: w1952 -> [w1966]
            shift-right: [w1962] -> w1946
            shift-left: w1951 -> [w1963]
            tunnel: w1950 -> [w1961]
            tunnel: w1949 -> [w1960]
            tunnel: w1948 -> [w1959]
            tunnel: [w1958] -> w1947
            stop <- w1972 stop-if-true
            n1237 = event shown="[0] Timeout" {
              selector: _ -> [_ _ _]
              dyn-events: _ -> [_ _ _]
              timeout: 0 -> [_ _ _]
              tunnel: w1966 -> [w1979 w1986 w2001]
              tunnel: [w1978 w1986 w2001] -> w1965
              tunnel: w1963 -> [w1977 w1987 w2002]
              tunnel: [w1976 w1987 w2002] -> w1962
              tunnel: w1961 -> [w1975 _ _]
              tunnel: w1960 -> [w1974 _ _]
              tunnel: w1959 -> [_ w1985 w2000]
              event Timeout {
                w1973 = 0  # timeout in ms
                # "Use a timeout of a few hundred ms if you want to acquire just fast enough to update the image- or a timeout of zero to run the camera at full speed."
                # "This VI sends the image to the loop above for display.\nIt's better to do this than to display here, because it separates the camera loop from the front panel a bit, and increases speed without sacrificing responsiveness of the UI.  Of course, using the event structure removes some of those benefits- but it is possible to write a high-performance camera loop with fast particle tracking, and still use this mechanism to display images without slowing down acquisition."
                # "If we're not dealing with other events, acquire from the camera."
                n1238 = event-data() -> ("Time"=w1984:u32)  [unwired: 1 in]
                n1239 = call <vilib>:"IMAQdx Grab.vi"("error in"=w1979, "Image In"=w1975, "Session In"=w1977) -> ("error out"=w1978:errorcluster, "Image Out"=w1981:T8, "Session Out"=w1976:T6)  [unwired: 5 in, 1 out]
                n1240 = call "IMAQ Clear Overlay"("Image"=w1981) -> ("Image Out"=w1980:T8)  [unwired: 9 in, 1 out]
                n1241 = Multiply(x=w1984, y=u32 1000) -> (x*y=w1982:u32)
                n1242 = call "imageQ_camera_hook.vi"("timeout in ms (0=don't wait if there are no requests)"=w1973, "Timestamp/us"=w1982, "ROI"=w1974, "Image"=w1980) -> ()  [unwired: 8 in]
              }
              event "Draw ROI", "Zoom": Value Change {
                # "This changes the current mouse mode on the image, allowing zooming/drawing of ROI (which can be useful if you want to window down a camera for particle tracking)."
                n1243 = event-data() -> ("CtlRef"=w1992:refnum<vi>)  [unwired: 1 in]
                n1244 = control-ref of="Draw ROI"() -> (w1993:refnum<vi>)
                n1245 = Equal?(x=w1993, y=w1992) -> (x = y?=w1991:bool)
                n1246 = case shown="True" w1991 {
                  tunnel: [w1996 w1999] -> w1990
                  tunnel: [TRUE ("stop") FALSE ("stop")] -> w1988
                  tunnel: [FALSE ("Update Indicators?") TRUE ("Update Indicators?")] -> w1989
                  frame False {
                    w1996 = u32 8 items=["Zoom Tool"=8, "Selection Tool"=0, "Pan Tool"=9, "Point Tool"=1, "Line Tool"=2, "Rectangle Tool"=3, "Rotated Rectangle Tool"=12, "Polyline Tool"=10, "Polygon Tool"=5, "Freehand Tool"=11, "Closed Freehand Tool"=6, "Ellipse Tool"=4, "Annulus Tool"=7] ("Current ROI Tool")
                  }
                  frame True {
                    w1999 = u32 3 items=["Zoom Tool"=8, "Selection Tool"=0, "Pan Tool"=9, "Point Tool"=1, "Line Tool"=2, "Rectangle Tool"=3, "Rotated Rectangle Tool"=12, "Polyline Tool"=10, "Polygon Tool"=5, "Freehand Tool"=11, "Closed Freehand Tool"=6, "Ellipse Tool"=4, "Annulus Tool"=7] ("Current ROI Tool")
                  }
                }
                n1247 = local write "Draw ROI"(w1989) -> ()
                n1248 = local write "Zoom"(w1988) -> ()
                n1249 = property on="Property Node" class="ImageControl"(reference=w1985, "Current ROI Tool"=w1990) -> ()  [unwired: 1 in, 2 out]
              }
              event "Zoom to Fit": Value Change {
                # "The various ROI tools are hidden, so the image control resizes nicely as the Red Tweezers window is resized.  The zoom to fit button/mouse mode buttons return some of this functionality."
                n1250 = event-data() -> ("NewVal"=w2003:bool)  [unwired: 1 in]
                n1251 = property on="Property Node" class="ImageControl"(reference=w2000, "Zoom to Fit Mode"=w2003) -> ()  [unwired: 1 in, 2 out]
              }
            }
            n1252 = feedback #14() -> (w1971:T27)  [unwired: 1 in]
            n1253 = call "Smoothed Frame Rate.vi"("Feedback In"=w1971, "Alpha"=0.05) -> ("Feedback Out"=w1970:T27, "Frame Rate"=w1967:dbl)  [unwired: 4 out]
            n1254 = feedback-in #14(w1970) -> ()
            n1255 = global write "red_tweezers_globals_INTERNAL_VOLATILE.vi" "Video Frame Rate"(w1967) -> ()
            n1256 = local read "stop"() -> (w1968:bool)
            n1257 = Unbundle By Name(w1965) -> ("status"=w1958:bool)
            n1258 = Or(x=w1958, y=w1968) -> (x .or. y?=w1972:bool)
          }
          n1259 = call <vilib>:"IMAQdx Close Camera.vi"("error in"=w1945, "Session In"=w1946) -> ()  [unwired: 9 in, 1 out]
        }
        frame condition #3 (active) {
          w2005 = 0 ("element")
          w2007 = 1920 ("dimension size")
          w2006 = 1080 ("dimension size")
          w2008 = T15 0 items=["Grayscale (U8)", "Grayscale (I16)", "Grayscale (SGL)", "Complex (CSG)", "RGB (U32)", "HSL (U32)", "RGB (U64)", "Grayscale (U16)"] ("Image Type")
          (unwired) FALSE ("background subtraction")
          # "This subdiagram generates a blank white image- useful if you don't have a camera"
          n1260 = Build Array(w2005, w2005, w2007, w2006) -> (w2004:i32[])
          n1261 = Initialize Array(u8 255 ("element"), w2006, w2007) -> (w2009:u8[][])
          n1262 = global write "red_tweezers_globals_INTERNAL.vi" "Global ROI"(w2004) -> ()
          n1263 = call "IMAQ Create"("Image Name"="red tweezers camera stub", "Image Type"=w2008) -> ("New Image"=w2010:T8)  [unwired: 2 in, 2 out]
          n1264 = call "IMAQ ArrayToImage"("Image Pixels (U8)"=w2009, "Image"=w2010) -> ("Image Out"=w2013:T8)  [unwired: 8 in, 1 out]
          n1265 = call "IMAQ Create"("Image Name"="Red Tweezers live image") -> ("New Image"=w2014:T8)  [unwired: 3 in, 2 out]
          n1266 = while {
            tunnel: w2013 -> [w2017]
            tunnel: w2014 -> [_]
            stop <- w2021 stop-if-true
            n1267 = local read "stop"() -> (w2021:bool)
            n1268 = Wait Until Next ms Multiple(millisecond multiple=u32 20) -> ()  [unwired: 1 out]
            n1269 = call "imageQ_camera_hook.vi"("Image"=w2017) -> ()  [unwired: 11 in]
            n1270 = feedback #15() -> (w2019:T27)  [unwired: 1 in]
            n1271 = call "Smoothed Frame Rate.vi"("Feedback In"=w2019) -> ("Feedback Out"=w2020:T27, "Frame Rate"=w2018:dbl)  [unwired: 1 in, 4 out]
            n1272 = feedback-in #15(w2020) -> ()
            n1273 = global write "red_tweezers_globals_INTERNAL_VOLATILE.vi" "Video Frame Rate"(w2018) -> ()
          }
        }
        frame condition #4 {
          # "Use this subdiagram if you have an external camera VI which writes to the image queue (using imageQ_camera_hook.vi)"
        }
        frame condition #5 {
          w2022 = path "C:/Users/Tweezer Cube/Desktop/red_tweezers_1_4_rc0/camera_for_rt136.llb/Particle Tracking.vi"  # Path to camera VI
          # "Use this subdiagram if you have an external camera VI which writes to the image queue (using imageQ_camera_hook.vi).  This is the slightly more sophisticated version, which checks that said external VI is running, and runs it if not."
          n1274 = Open VI Reference(vi path=w2022) -> (vi reference=w2023:refnum<vi>, error out=w2025:errorcluster)  [unwired: 5 in]
          n1275 = property class="VI"(reference=w2023) -> ("Path"=w2024:path)  [unwired: 1 in, 2 out]
          n1276 = global write "red_tweezers_globals_INTERNAL_VOLATILE.vi" "Current Camera VI"(w2024) -> ()
          n1277 = property class="VI"(reference=w2023, error in=w2025) -> (reference out=w2030:refnum<vi>, error out=w2029:errorcluster, "Exec.State"=w2027:T29)
          n1278 = Equal?(x=w2027, y=T29."Idle") -> (x = y?=w2031:bool)
          n1279 = case shown="True" w2031 {
            tunnel: w2030 -> [w2035 w2044]
            tunnel: w2029 -> [w2034 w2041]
            tunnel: [w2033 w2040] -> w2026
            tunnel: w2027 -> [w2037 _]
            frame False {
              n1280 = Close Reference(reference=w2035, error in (no error)=w2034) -> (error out=w2033:errorcluster)
              n1281 = Equal?(x=w2037, y=T29."Bad") -> (x = y?=w2036:bool)
              n1282 = case shown="False" w2036 {
                frame False {
                }
                frame True {
                  n1283 = One Button Dialog(message="The external camera VI is not running and cannot be started- it's probably broken or missing.  Check the static/dynamically loaded VI reference in the bottom loop on the block diagram.") -> ()  [unwired: 1 in, 1 out]
                }
              }
            }
            frame True {
              n1284 = invoke class="VI" method="Run VI"(reference=w2044, error in=w2041, "Wait until done"=FALSE ("Wait Until Done"), "Auto Dispose Ref"=TRUE ("Auto Dispose Reference")) -> (error out=w2040:errorcluster)  [unwired: 1 in, 4 out]
            }
          }
          n1285 = call <vilib>:"Simple Error Handler.vi"("error source (\" \")"="External camera VI (see the bottom loop in the block diagram)" ("error source (\" \")"), "error in (no error)"=w2026) -> ()  [unwired: 3 in, 5 out]
        }
      }
    }
  }
  n1286 = while {
    tunnel: w12 -> [w2062]
    shift-right: [w2061] -> w11
    shift-left: w13 -> [w2063]
    shift-right: [w2058] -> _
    shift-left: _ -> [w2051]
    shift-right: [w2057] -> _
    shift-left: _ -> [w2055]
    shift-right: [w2056] -> _
    shift-left: FALSE ("Saving") -> [w2052]
    stop <- w2060 stop-if-true
    w2049 = u32 50 ("millisecond multiple")
    # "Start/stop saving data, if necessary"
    n1287 = Divide(x=u32 1000, y=w2049) -> (x/y=w2047:dbl)
    n1288 = Wait Until Next ms Multiple(millisecond multiple=w2049) -> ()  [unwired: 1 out]
    n1289 = call "imageQ_dequeue.vi"("timeout in ms (-1)"=2000, "Return queue"=w2063, "Image Dst"=w2062) -> ("Timestamp/us"=w2053:u64, "Return queue out"=w2061:refnum<queue>, "Image Dst Out"=w2064:T8, "timed out?"=w2067:bool, "ROI"=w2046:u64[])  [unwired: 4 in]
    n1290 = Not(x=w2067) -> (.not. x?=w2065:bool)
    n1291 = case shown="True" w2065 {
      tunnel: w2064 -> [_ w2101]
      tunnel: w2055 -> [w2094 w2104]
      tunnel: w2052 -> [_ w2098]
      tunnel: [w2094 w2099] -> w2054
      tunnel: w2053 -> [_ w2102]
      tunnel: w2051 -> [w2095 w2103]
      tunnel: [w2095 w2100] -> w2050
      tunnel: w2046 -> [_ w2097]
      frame False {
      }
      frame True {
        n1292 = global read "red_tweezers_globals_INTERNAL.vi" "Image Overlay (extras from control loop)"() -> (w2112:T18[])
        n1293 = case shown="True" w2098 {
          tunnel: w2104 -> [w2113 w2115]
          tunnel: w2103 -> [w2114 w2121]
          tunnel: w2102 -> [_ w2120]
          tunnel: w2101 -> [_ w2119]
          tunnel: [w2114 w2118] -> w2100
          tunnel: [w2113 w2117] -> w2099
          frame False {
          }
          frame True {
            n1294 = call "save_data_save.vi"("Image"=w2119, "Timestamp"=w2120, "Avi Refnum"=w2115, "Data refnum"=w2121) -> ("error out"=w2116:errorcluster, "Avi Refnum (duplicate)"=w2117:T30, "Data refnum (duplicate)"=w2118:refnum<file>)  [unwired: 5 in]
            n1295 = case shown="Error" w2116 {
              selector: w2116 -> [_ w2123]
              frame No Error {
              }
              frame Error {
                n1296 = call <vilib>:"Clear Errors.vi"("error in (no error)"=w2123) -> ()  [unwired: 5 in, 2 out]
                n1297 = local write "Save Video"(FALSE ("Save")) -> ()
              }
            }
          }
        }
        n1298 = global write "red_tweezers_globals_INTERNAL.vi" "Global ROI"(w2097) -> ()
        n1299 = global read "red_tweezers_globals_INTERNAL_VOLATILE.vi" "Tracked Spot Positions (3D)"() -> (w2105:cluster{"x":dbl, "y":dbl, "Z":dbl}[])
        n1300 = global read "red_tweezers_globals.vi" "Selection/Group"() -> (w2111:T7[])
        n1301 = global read "red_tweezers_globals.vi" "Spots"() -> (w2110:T1[])
        n1302 = call "overlay_positions.vi"("Positions"=w2105, "Image"=w2101) -> ("Image 2"=w2107:T8)  [unwired: 9 in]
        n1303 = call "render_overlay_elements.vi"("Image Overlay (extras from control loop)"=w2112, "Image"=w2107) -> ("Image Out"=w2109:T8)  [unwired: 5 in]
        n1304 = call "grid_and_guides.vi"("Operation"=T12."Render on image", "Image"=w2109) -> ("Image Out"=w2096:T8)  [unwired: 9 in]
        n1305 = call "overlay_spots_on_image.vi"("Selection and Groups"=w2111, "Spots"=w2110, "image"=w2096) -> ("Image"=→"Image":T8)  [unwired: 3 in, 1 out]
      }
    }
    n1306 = global read "red_tweezers_globals_INTERNAL_VOLATILE.vi" "Video Frame Rate"() -> (→"Video Frame Rate":dbl)
    n1307 = case shown="True" "Save Video" {
      tunnel: [w2070 w2085] -> w2058
      tunnel: [w2069 w2079] -> w2057
      tunnel: [FALSE ("Saving") w2084] -> w2056
      tunnel: w2052 -> [w2073 w2083]
      tunnel: w2054 -> [w2071 w2082]
      tunnel: w2050 -> [w2072 w2081]
      tunnel: w2047 -> [_ w2080]
      frame False {
        n1308 = case shown="True" w2073 {
          tunnel: w2072 -> [w2075 w2078]
          tunnel: w2071 -> [w2074 w2077]
          tunnel: [w2075 _] -> w2070
          tunnel: [w2074 _] -> w2069
          frame False {
          }
          frame True {
            n1309 = local write "Save Video"(FALSE ("Save")) -> ()
            n1310 = call "save_data_stop.vi"("Avi Refnum"=w2077, "Data refnum"=w2078) -> ()  [unwired: 10 in]
          }
        }
      }
      frame True {
        n1311 = case shown="False" w2083 {
          selector: w2083 -> [_ w2093]
          tunnel: [w2090 w2091] -> w2085
          tunnel: [w2089 w2092] -> w2079
          tunnel: [w2086 w2093] -> w2084
          tunnel: w2082 -> [_ w2092]
          tunnel: w2081 -> [_ w2091]
          tunnel: w2080 -> [w2088 _]
          frame False {
            n1312 = call "save_data_start.vi"("Save Video"=TRUE, "Frames Per Second"=w2088) -> ("Saving"=w2086:bool, "Avi Refnum"=w2089:T30, "Data Refnum"=w2090:refnum<file>)  [unwired: 3 in]
            n1313 = local write "Save Video"(w2086) -> ()
          }
          frame True {
          }
        }
      }
    }
    n1314 = local read "stop"() -> (w2060:bool)
  }
  n1315 = Release Queue(queue=w11) -> ()  [unwired: 2 in, 3 out]
  n1316 = case shown="True" w6 {
    frame False {
    }
    frame True {
      n1317 = One Button Dialog(message="Warning: there was a camera error.  You may need to restart Red Tweezers.") -> ()  [unwired: 1 in, 1 out]
    }
  }
  n1318 = flat-sequence {
    tunnel: w21 -> [w2129]
    tunnel: w20 -> [_]
    frame #0 {
      # "This autosaves when we stop.  The sequence structures are necessary so that:\n1. loading settings doesn't stop the VI\n2. plugins are still open (and hence saved) when we save settings"
      n1319 = local read "Plugins"() -> (w2132:T3)
      n1320 = global read "red_tweezers_globals_INTERNAL_VOLATILE.vi" "Current Settings File"() -> (w2126:path)
      n1321 = global read "red_tweezers_globals_INTERNAL_VOLATILE.vi" "Save Settings On Exit"() -> (w2125:bool)
      n1322 = flat-sequence {
        tunnel: w2129 -> [w2135]
        tunnel: [w2135] -> w2128
        frame #0 {
          n1323 = local write "stop"(FALSE ("STOP")) -> ()
        }
      }
      n1324 = case shown="True" w2125 {
        tunnel: w2126 -> [_ w2140]
        tunnel: w2128 -> [w2137 w2138]
        tunnel: [w2137 w2138] -> w2127
        frame False {
        }
        frame True {
          n1325 = Path To String(path=w2140) -> (string=w2139:string)
          n1326 = call "settings_save_to_file.vi"("XML File Path"=w2140) -> ()  [unwired: 11 in]
          n1327 = call "settings_filename_to_registry.vi"("Last Used Settings File"=w2139) -> ()  [unwired: 11 in]
        }
      }
      n1328 = flat-sequence {
        tunnel: w2127 -> [w2133]
        tunnel: [w2133] -> _
        frame #0 {
          n1329 = local write "stop"(TRUE ("STOP")) -> ()
        }
      }
      n1330 = control-ref of="Plugin Pnl"() -> (w2130:refnum<vi>)
      n1331 = control-ref of="Plugin:"() -> (w2131:refnum<vi>)
      n1332 = call "plugins_unload.vi"("error in (no error)"=w2127, "Plugins"=w2132, "Sub Panel"=w2130, "Plugin Chooser"=w2131) -> ()  [unwired: 2 in, 2 out]
    }
  }
  n1333 = Subtract(x=w3, y=w1) -> (x-y=→"Execution Time":u32)
